vi "BIMS_SA.vi"() -> ()   [LabVIEW 2010]
doc: "This program is currently beta software. It is designed to address the data requirements defined primarily by the DHB Ballistic Test Report.\n\nThe general operation of this program is based on the Ballistics Version 2005 application developed internally by DuPont as a research tool for the Spruance Plant Ballistics Lab in Richmond, VA.\n\nPlease note that the original trigger control logic was modified and no longer depends on a safety interlock system to enable operation of a ballistic test.\n\nDuPont makes no warranties and assumes no liabilities in connection with any use of this program."
uses:
  Shot Record.ctl
  <vilib>/Utility/NIReport.llb/NI_report.lvclass
  <vilib>/Utility/config.llb/Write Key (String).vi
  <vilib>/Utility/NIReport.llb/Append Report Text (str wrap).vi
  <vilib>/Utility/NIReport.llb/Append Text Table to Report (wrap).vi
  <vilib>/addons/database/Connection.llb/DB Tools Open Connec (String).vi
  <vilib>/addons/database/Connection.llb/Conn Execute.vi
  <vilib>/addons/database/Recordset.llb/Rec Destroy - Connection.vi
  <vilib>/Utility/config.llb/Write Key (I32).vi
  <vilib>/addons/database/NI_Database_API.lvlib
  <vilib>/Utility/config.llb/NI_LVConfig.lvlib
  <vilib>/Analysis/NI_AALBase.lvlib
  <vilib>/Utility/NIReport.llb/Excel/NI_Excel.lvclass
panel:
  out "timestamp":string
  out "deployment":string
  in  "RESET All":bool
  in  "EXIT":bool
  in  "STOP":bool
  in  "mainTabCntrl":enum32{"SETUP", "MEASURE", "HISTORY", "ABOUT"}(tab)
  in  "setupTabCntrl":T1(tab)
  in  "rangeSetup":u16(ring) caption="Range\nSetup" items=["Select . . .", "Small frag (short)", "Handgun (standard)", "Rifle (long)"]
  out "mid_to_targ_dist":sgl=7.5 caption="Midpoint To Target (ft)"
  in  "Thickness":dbl caption="Thickness (in)" format="%.2f"
  in  "Model":u16(ring) caption="Model #"
  in  "clayCalArray":i16[](array[numeric])=[0, 0, 0, 0, 0] caption="Calibration" min=0 max=99 format="%02.0f"
  in  "Panel Dimensions":u16(ring)=6 caption="Panel Size" items=["15x15", "CHEST PLATE", "HELMET", "12x15", "16X16", "18X18", "20X16", "15\" x 18\"", "24 x 24", "13\"X13\"", "7.5\" X 7.5\"", "15x15", "VEST PANEL", "12X12", "101/4\" X 113/4\"", "15X16", "26X26", "NOT APPLICABLE", "8.5\" X 11\""]
  out "threatDetails":T2
  in  "projectileWt":u16(ring) caption="Weight (gr)" items=["Select . . .", "2", "4", "16", "17", "44", "45", "55", "62", "64", "85", "110", "115", "123", "124", "127", "148", "158", "166", "180", "207", "240"]
  out "clayAverage":sgl caption="Clay Average" format="%#.1f"
  in  "clayTemp":sgl caption="Clay Temperature" format="%.1f"
  in  "RoomT":sgl caption="Room Temperature" format="%.1f"
  in  "RoomHum":sgl caption="Room Humidity" min=0 max=100 format="%.1f"
  in  "Sample #":string
  in  "Comments":string caption="Remark"
  in  "recorder":u16(ring) caption="Recorder"
  in  "shooter":u16(ring) caption="Shooter"
  in  "rangeNum":u16(ring) caption="Range #" items=["1", "2", "Other"]
  in  "projectileType":u16(ring) caption="Projectile"
  in  "weapon":u16(ring) caption="Weapon"
  in  "minV50":i32=1500 caption="Min. V50"
  in  "covering":u16(ring) caption="Ballistic\nCover"
  in  "totalSampleWt":sgl caption="Total Wt (lbs)" format="%.2f"
  in  "serialNum":string caption="Serial #"
  in  "workType":u16(ring) caption="Work Type" items=["R&D", "QC", "Other"]
  in  "projNum":string caption="Project #"
  in  "projName":string caption="Project\nName"
  in  "standard":u16(ring) caption="Standard" items=["n/a", "NIJ 0101.04", "MIL-STD-662F"]
  in  "Powder Type":u16(ring) caption="Powder\nType" items=["WINCHESTER-231", "Alliant Herc. Bullseye", "Power Pistol", "ACCURATE, NO.9", "ACCURATE, NO. 2", "IMR-4756", "OTHER", "WINCHESTER-296", "Alliant 2400", "IMR-4198", "IMR-4895", "Hi-Skor 700x", "Hi-Skor 800x", "International Clay's", "Winchester Ball", "Hercules"]
  in  "Method":u16(ring) items=["V50", "N.I.J.", "Quasi N.I.J.", "VsVr", "CUSUM", "V(0)", "V(0) @ 1450", "V(0) @ 1500", "V(0) @ 1550"]
  in  "Layer_1":T3={"plyNum"=0, "LotNum"="n/a", "RollNum"="n/a", "Fabric.stitch"=1} caption="Fabric #1" {"plyNum" min=0 max=99 step=5}
  in  "Layer_2":T3={"plyNum"=0, "LotNum"="n/a", "RollNum"="n/a", "Fabric.stitch"=1} caption="Fabric #2" {"Fabric.stitch" items=["Corners", "Other", "n/a"]; "plyNum" min=0 max=99 step=5}
  in  "Layer_3":T3={"plyNum"=0, "LotNum"="n/a", "RollNum"="n/a", "Fabric.stitch"=1} caption="Fabric #3" {"Fabric.stitch" items=["Corners", "Other", "n/a"]; "plyNum" min=0 max=99 step=5}
  in  "Layer_4":T3={"plyNum"=0, "LotNum"="n/a", "RollNum"="n/a", "Fabric.stitch"=1} caption="Fabric #4" {"Fabric.stitch" items=["Corners", "Other", "n/a"]; "plyNum" min=0 max=99 step=5}
  in  "Layer_5":T3={"plyNum"=0, "LotNum"="n/a", "RollNum"="n/a", "Fabric.stitch"=1} caption="Fabric #5" {"Fabric.stitch" items=["Corners", "Other", "n/a"]; "plyNum" min=0 max=99 step=5}
  in  "Layer_6":T3={"plyNum"=0, "LotNum"="n/a", "RollNum"="n/a", "Fabric.stitch"=1} caption="Fabric #6" {"Fabric.stitch" items=["Corners", "Other", "n/a"]; "plyNum" min=0 max=99 step=5}
  out "fabAttribs_1":T4 caption="fabricAttribs_1"
  out "fabAttribs_2":T4 caption="fabricAttribs_2"
  out "fabAttribs_3":T4 caption="fabricAttribs_3"
  out "fabAttribs_4":T4 caption="fabricAttribs_4"
  out "fabAttribs_5":T4 caption="fabricAttribs_5"
  out "fabAttribs_6":T4 caption="fabricAttribs_6"
  in  "fabStyle_1":u16(ring)
  in  "fabStyle_2":u16(ring)
  in  "fabStyle_3":u16(ring)
  in  "fabStyle_4":u16(ring)
  in  "fabStyle_5":u16(ring)
  in  "fabStyle_6":u16(ring)
  in  "fabVendor_1":u16(ring) caption="vendor" items=[" Select Vendor . . .", "Barrday", "Cushman", "DSM", "FMS", "Hexcell", "Honeywell", "Lincoln", "Pro Systems", "TEIJIN", "TexTech"]
  in  "fabVendor_2":u16(ring) caption="vendor" items=[" Select Vendor . . .", "Barrday", "Cushman", "DSM", "FMS", "Hexcell", "Honeywell", "Lincoln", "Pro Systems", "TEIJIN", "TexTech"]
  in  "fabVendor_3":u16(ring) caption="vendor" items=[" Select Vendor . . .", "Barrday", "Cushman", "DSM", "FMS", "Hexcell", "Honeywell", "Lincoln", "Pro Systems", "TEIJIN", "TexTech"]
  in  "fabVendor_4":u16(ring) caption="vendor" items=[" Select Vendor . . .", "Barrday", "Cushman", "DSM", "FMS", "Hexcell", "Honeywell", "Lincoln", "Pro Systems", "TEIJIN", "TexTech"]
  in  "fabVendor_5":u16(ring) caption="vendor" items=[" Select Vendor . . .", "Barrday", "Cushman", "DSM", "FMS", "Hexcell", "Honeywell", "Lincoln", "Pro Systems", "TEIJIN", "TexTech"]
  in  "fabVendor_6":u16(ring) caption="vendor" items=[" Select Vendor . . .", "Barrday", "Cushman", "DSM", "FMS", "Hexcell", "Honeywell", "Lincoln", "Pro Systems", "TEIJIN", "TexTech"]
  out "fab6_totalWt":sgl caption="Fab6 Wt" min=0 max=99 step=5 format="%.2f"
  out "fab5_totalWt":sgl caption="Fab5 Wt" min=0 max=99 step=5 format="%.2f"
  out "fab4_totalWt":sgl caption="Fab4 Wt" min=0 max=99 step=5 format="%.2f"
  out "fab3_totalWt":sgl caption="Fab3 Wt" min=0 max=99 step=5 format="%.2f"
  out "fab2_totalWt":sgl caption="Fab2 Wt" min=0 max=99 step=5 format="%.2f"
  out "fab1_totalWt":sgl caption="Fab1 Wt" min=0 max=99 step=5 format="%.2f"
  out "totalNumPlies":i32 caption="Total # of Plies" min=0 max=100 step=5
  out "totalBAW":sgl caption="Total BAW (psf)" format="%.2f"
  in  "Next Shot":bool
  in  "Delete Button":bool
  in  "SHOTS":T5[](array[typedef]) {"UncorrectedAvgVel_PB" format="%.1f"; "strikeVel_PB" format="%.1f"; "velLoss_PB" format="%.1f"; "avgVel_PB" format="%.1f"; "Redundant_Velocity" format="%.1f"; "Energy Loss (J)" format="%.3e"; "Projectile Mass" min=0 step=1 format="%.4f"; "Corrected residual" format="%.2f"; "Uncorrected Residual" format="%.2f"; "Corrected Impact" format="%.2f"; "Uncorrected Impact" format="%.2f"; "Shot Angle" max=90 step=1; "SHOT STATUS" items=["Partial", "Complete"]; "IMPACT VELOCITY" min=0 max=10000 step=0.1 format="%.1f"; "Barrel Temperature" format="%.1f"; "Powder Loading" format="%.4f"; "RESIDUAL  VELOCITY" min=0 max=10000 step=0.1 format="%.1f"}
  in  "Refresh":bool
  in  "Accept Data":bool caption="RANGE SETUP must be selected before shots can be added."
  in  "Clear":bool
  out "Shot":i32
  out "Panel":i32
  out "rangeOfResults":i32 caption="Range of Results" min=0 max=10000 step=1
  out "lowComplete":i32 caption="LOW Complete" min=0 max=10000 step=1
  out "highPartial":i32 caption="HIGH Partial" min=0 max=10000 step=1
  out "Avg/speed":sgl caption="Average" min=0 max=10000 step=0.1 format="%.1f"
  in  "Current/avg/speed":sgl caption="Average" min=0 max=1000000 step=0.1 format="%.1f"
  out "Redundant/speed":sgl caption="Chronograph 2" min=0 max=10000 step=0.1 format="%.1f"
  in  "backfacedia":sgl caption="BF Diameter"
  in  "backdepth":sgl caption="BF Depth"
  out "% Difference":sgl format="%.1f"
  out "zmr 2":sgl caption="Z.M.R." format="%.1f"
  out "Pairs":i16 min=0 max=100 step=1
  out "computed_V50":sgl caption="Value" format="%.1f"
  in  "maxDev":sgl=125.0 caption="Maximum\nDeviation" min=0 max=300 step=25 format="%.1f"
  in  "B.F.S (mm)":u16 caption="B.F.S"
  in  "N.I.J":u16(ring) items=["Not Tested", "PASS", "FAIL"]
  in  "Projectile Mass":sgl caption="Proj Mass (g)" min=0 step=1 format="%.4f"
  in  "Shot Angle":u16 max=90 step=1
  in  "Powder Loading":sgl min=0 max=100 step=0.1 format="%.3f"
  in  "Shot Decription":string
  in  "Barrel Temp":sgl format="%.1f"
  out "DC_ factor":sgl caption="Correction Factor (Mid-Chrono 1&2)" format="%.4f"
  in  "Current/redundant/speed":sgl caption="Chronograph 2" min=0 max=1000000 step=0.1 format="%.1f"
  in  "currentDateTime":string caption="SUBMIT DATE/TIME"
  in  "Current/residual/speed":sgl caption="Residual" min=0 max=10000 step=0.1 format="%.1f"
  in  "Current/sthotstatus":u16(ring) caption="Penetration" items=["Partial", "Complete"]
  in  "Current/impact/speed":sgl caption="Chronograph 1" min=0 max=10000 step=0.1 format="%.1f"
  out "BACKFACE DEPTH":sgl caption="Backface\nDepth" min=0 max=200 step=5
  out "BACKFACE DIAMETER":sgl caption="Backface\nDiameter" min=0 max=100 step=5
  in  "Reject shot":bool
  out "SUBMIT DATE/TIME":string
  out "residual/speed":sgl caption="Residual" min=0 max=10000 step=0.1 format="%.1f"
  out "SHOT STATUS":u16(ring) caption="Penetration" items=["Partial", "Complete"]
  out "Impact/speed":sgl caption="Chronograph 1" min=0 max=10000 step=0.1 format="%.1f"
  in  "Table of Shots":string[][](table) caption="Shot Table"
  in  "RANGE RESET":bool=TRUE caption="ARMED"
  in  "Save":bool caption="Number of plies must be in FABRIC INFORMATION and \nSHOTS must exst in above table to enable saving"
  in  "Report_PB":bool caption="Report"
  in  "Report Path":path=path "c:/ballistics"
  out "instruct_addShot":string="RANGE SETUP must be selected before shots can be added."
  in  "historyTabCntrl":T6(tab)
  in  "srchParams":T7={"maxPanels"=1001, "lkupPanelStartDate"=timestamp(0 s since 1904-01-01), "lkupPanelEndDate"=timestamp(3253624514.0909824 s since 1904-01-01), "qWorkType"=0, "Model"=0, "fabStyle_0"=0, "fabVendor_0"=0} {"fabVendor_0" items=[" Select Vendor . . .", "Barrday", "Cushman", "DSM", "FMS", "Hexcell", "Honeywell", "Lincoln", "Pro Systems", "TEIJIN", "TexTech"]; "Model" items=["All Models", "n/a", "undefined", "other"]; "qWorkType" items=["All Types", "R&D", "QC", "Other"]; "lkupPanelEndDate" format="%<%x>T"; "lkupPanelStartDate" format="%<%x>T"; "maxPanels" min=1 max=10000 step=100}
  out "actualNumPanels":i32=1001 caption="Actual # Returned"
  out "pastPanels":string[][](table)
  in  "Record #":i32=1 min=0 max=37
  in  "getRecord":bool
  out "fabAttribs_0":T4 caption="fabricAttribs_1"
  in  "QueryLoad":bool
  in  "lkupEndDate":timestamp caption="End Date" format="%<%x>T"
  in  "lkupStartDate":timestamp caption="Begin Date" format="%<%x>T"
  out "Vel.vs.Loading":cluster{dbl[], dbl[]}(graph)
  out "v50_table":string[][](table)
  in  "maxRecs":u16=1001 caption="Max # of SHOT Records" min=1 max=10000 step=100
  out "ActualNumRecs":i32=1001 caption="Actual # Returned"
  out "Previous V50 Data":cluster{dbl, dbl, dbl[][]}(graph)={0.0, 1.0, []}
  out "v50 data":string[][](table)
  out "Average Velocity":dbl format="%.1f"
  out "CUSUM_lastVel":dbl caption="Latest Velocity" format="%.1f"
  out "CUSUM_stdDev":dbl caption="Std. Deviation" format="%.1f"
  in  "queryThreat":u16(ring) caption="Threat" items=["115-GRAIN,9mm LUGER,REFERENCE ROUND,10\" .38 cal TEST BBL.", "158-grain,WIN. 357 MAG, JHP REFERENCE ROUND, 10\" SAMMI TEST BBL.", "180-grain,WIN. 308 POWER-POINT REFERENCE ROUND, 308 TEST BBL.", "240-grain,REM. .44 mag, JSP REFERENCE ROUND, 8\" SAMMI TEST BBL."]
  out "In Control":bool=TRUE caption="Control Status"
  in  "Panel Search":bool
  in  "beginCUSUM":string="1/1/1900" caption="Begin Date"
  in  "endCUSUM":string="1/1/2100" caption="End Date"
  in  "aboutTabCntrl":T8(tab)
  out "Device S/N":string="DEVICE NOT READY!" caption="Timing Device S/N"
  in  "Data Source":u16(ring)=2 items=["Simulated", "Radar", "Screens", "Manual"]
  out "Distance Units":string="FEET"
  out "Weight Units":string="GRAMS"
  out "dbConn":string caption="Database Connection"
  in  "Sort by AVG":bool=TRUE caption="Sort shots by average velocity"
  out "configPath":path caption="Configuration Path (INI)"
  in  "Add Disclaimer":bool
  in  "Report":bool
  out "Shot Graph":cluster{i32[], sgl[]}[](graph)
  out "Corrected Average":sgl=2206.6846 format="%.2f"
  out "Corrected Redundant":sgl=2256.401 format="%.2f"
  out "conversion factor":sgl=0.3048037 format="%.5f"
  out "number of completes":i32=2
  out "number of partials":i32=2
  in  "percent warning":sgl=1.0 format="%.2f"
  in  "Version":dbl format="%.2f"
  out "impact/ID":u32=83886081 format="%.0x"
  out "residual/ID":u32=83951617 format="%.0x"
  out "Red/ID":u32=84017153 format="%.0x"
  out "correction coefficient":sgl=0.0252 format="%.8f"
  out "Corrected Residual":sgl=1210.3492 format="%.2f"
  out "Corrected Impact":sgl=2171.1157 format="%.2f"
  out "Impact/Separation":sgl=4.0 format="%.2f"
  out "Barrel to Screen":sgl=7.8333 format="%.2f"
  in  "Impact/Target Dist":sgl=7.083333 format="%.2f"
  out "Residual/Separation":sgl=4.0 format="%.2f"
  in  "Residual/Target Dist":sgl=7.083333 format="%.2f"
  out "Z.M.R.":sgl min=0 step=0.1 format="%.1f"
  in  "old threat":u16
  out "Complete":sgl[](array[numeric]) format="%.2f"
  out "factor array":sgl[](array[numeric])=[0.0252, 0.0191, 0.0191, 0.0441, 0.0425, 0.0131, 0.018] format="%.4f"
  out "Partial":sgl[](array[numeric]) format="%.2f"
  in  "DAQ Card":i16=1
  in  "Impact Timer":i16 min=0 max=3 step=1
  in  "Redundant Timer":i16=1 min=0 max=3 step=1
  in  "Residual  Timer":i16=2 min=0 max=3 step=1
  in  "Drag Corrected":bool
  out "Impact factor":sgl=0.94704616 caption="Impact" min=0 max=1 format="%.5f"
  out "Residual factor":sgl=1.0559148 caption="Residual" min=0 max=1 format="%.5f"
  in  "ballistician":u16(ring) caption="Ballistician" items=["n.a."]
  in  "Threat 2":u16(ring) caption="Threat" items=["110-grain(non-toxic)NYLON, 38 SPECIAL, POLY-TUNGSTEN, 10\" SAMMI TEST BBL.", "115-GRAIN,9mm LUGER,REFERENCE ROUND,.38 caliber chamber,10\" TEST BBL.", "115-GRAIN,9mm LUGER,REFERENCE ROUND,10\", 9mm, TEST BBL.", "115-grain, 9 mm, HI-SHOK JHP, +P+ FEDERAL, 10\" SAMMI TEST BBL.", "115-grain, 9 mm, HI-SHOK JHP, +P+ FEDERAL, 5\" SAMMI TEST BBL.", "115-grain,9mm,SMJ,SVENKA-BULLET,CHILE,S.A. 10\"SAMMI TEST BBL.", "123-grain,7.62mm AK-47            7.62mm SAAMI test bbl.", "124-grain,9mm FMJ Rem.#23558, 10\".357cal.SAAMI test bbl.", "124-grain,9mm,FMJ,Rem.#23558, .38 caliber chamber, 10\"SAAMI test bbl.1/10\" TWIST", "124-grain,9mm,FMJ,Rem.#23558, 10\"SAAMI test bbl.", "124-grain,9mm,FMJ,Rem.#23558, 5\"SAAMI test bbl.", "127-grain,9mm,SXT/Blck Tln, +P+,Win.RA9SXT SAAMI test bbl.", "148 grain 7.62 x 51 mm M80 ball", "148-grain,7.62mm FMJ  M80     7.62mm SAAMI test bbl.", "158-grain,0.357, JSP, Rem.#22487 10\"SAAMI test bbl.", "158-grain,0.357, JSP,SPEER.#4217,10\"SAAMI test bbl.", "158-grain,WIN. 357 MAG, JHP REFERENCE ROUND, 10\" SAMMI TEST BBL.", "16-grain,  saboted RCC,.308cal.SAAMI test bbl.,DC", "166-grain,.30 cal. M2 AP, 7.62mm SAAMI test bbl.", "17-grain,sabot,STANAG 2920, FSP,.308 cal. SAMMI test bbl., DC", "17-grain,sabot.Type 1,FSP,.308cal.SAAMI test bbl.,DC", "17-grain,sabot.Type 2,FSP,.308cal.SAAMI test bbl.,DC", "180-grain,40 cal. S&W, 5\"SAMMI test bbl.", "180-grain,WIN. 308 POWER-POINT REFERENCE ROUND, 308 TEST BBL.", "2-grain, saboted RCC FSP,.223cal.SAAMI test bbl.,DC", "207 grain, FSP, 50 Cal", "240 grain,0.44, SWC Speer #4660 no gc,8\"SAAMI test bbl.", "240-grain,0.44, FMJ Speer #4459, 8\" SAMMI test bbl.", "240-grain,0.44, JSP Speer #4457       8\"SAAMI test bbl.", "240-grain,0.44, SJHP,  REM.  # 23592,   8\"SAAMI test bbl.", "240-grain,0.44, SWC PMC w/Gas Check   8\"SAAMI test bbl.", "240-grain,REM. .44 mag, JSP REFERENCE ROUND, 8\" SAMMI TEST BBL.", "4-grain, saboted RCC FSP ,.223cal.SAAMI test bbl.,DC", "44-grain, 0.30-cal FSP - no sabot", "44-grain, 0.30-cal FSP - no sabot", "44-grain,sabot.      FSP,.458cal.SAAMI test bbl.,DC", "45-grain,JHP(WIN), .223 cal. SAMMI test bbl.", "55-grain, 0.223 M-193 FMJ        .223cal.SAAMI test bbl.", "62-grain, 0.223 M-855 Green Tip  .223cal SAAMI test bbl.", "64-grain,sabot.  RCC,.458cal.SAAMI test bbl.,DC", "85-grain(non-toxic), 38 SPECIAL FRANGIBLE,WIN # RA38DF,10\" SAMMI TEST BBL.", "85-grain(non-toxic), 9mm FRANGIBLE +P+,WIN # RA9DF, 5\" SAMMI TEST BBL.", "85-grain(non-toxic), 9mm FRANGIBLE +P+,WIN # RA9DF,10\" SAMMI TEST BBL.", "85-grain, 7.62mm Tokarev(LEAD CORE-STEEL JACKET,1992)Tokarev SAAMI test bbl."]
  in  "Panel Backing":u16(ring) items=["miscellaneous", "Clay (ROMA Plastilina # 1)", "Aluminum, 24 ga. (.020,.2024-T3) Witness Plate", "None"]
  in  "Submitter":u16(ring) items=["other"]
  in  "Test Conditions":u16(ring) items=["Dry", "Wet", "Hot 160 DEG. F", "Cold", "WEAPON LUBRICANT", "MOTOR OIL", "CONDITIONED", "ACCELERATED AGEING"]
  in  "Panel Stitch":u16(ring)=5 items=["TEST PANEL/NORMAL STITCH", "TEST PANEL/CUSTOM STITCH", "VEST PANEL/CUSTOM STITCH", "HARD PANEL", "CAR ARMOR LAMINATE PANEL", "N.A."]
  in  "Panel Type":u16(ring)=4 items=["FABRIC ARMOR", "COMPOSITE ARMOR", "LG.RIGHT FRONT VEST PANEL", "HELMET", "N.A."]
  in  "Type":u16(ring) items=["none"]
  in  "Manufacturer":u16(ring)=1 caption="Mfr" items=["Point Blank-Marine Interceptor"]
  in  "Areal Density":dbl format="%.2f"
  in  "Areal density text":string
  in  "Fabric Description":string
  in  "Weight of Panel":dbl format="%.4f"
  in  "Panel Technician":u16(ring) items=["Not Known", "none", "POINT BLANK"]
  in  "clayCalib":string="##-##-##-##-##" caption="Calibration"
  in  "lookupRec":bool caption="lookup"
  out "connStr":string
  in  "message control":bool
  # "yes"
  # "BIMS"
  # "Version 2011 for"
  # "No"
  # "GENERAL"
  # "SAMPLE"
  # "THREAT"
  # "RANGE"
  # "° F"
  # "%"
  # "° F"
  # "mm"
  # "mm"
  # "in"
  # "STRIKE FACE -------------------------------------------------------- MODEL CONSTRUCTION -------------------------------------------------------- BODY SIDE"
  # "Fabric 1"
  # "Fabric 2"
  # "Fabric 3"
  # "Fabric 4"
  # "Fabric 5"
  # "Fabric 6"
  # "Vendor"
  # "Style #"
  # "# of Plies"
  # "Lot#"
  # "Roll#"
  # "Stitch"
  # "ID#"
  # "Fiber"
  # "Denier"
  # "Pick"
  # "Weave"
  # "Finish"
  # "oz/yd²"
  # "Total Wt"
  # "Edit any non-date field by placing cursor in field. \n\nProperties not listed are controlled by the current shot, test description or Fabric information.  \nIf the entry is changed for the current shot, then all previous shots are changed"
  # "V50"
  # "Current Shot Data"
  # "(mm)"
  # "Number of plies must be in FABRIC INFORMATION and \nSHOTS must exst in above table to enable saving"
  # "Last Assigned\nRecord Numbers"
  # "ID#"
  # "Fiber"
  # "Denier"
  # "Pick"
  # "Weave"
  # "Finish"
  # "oz/yd²"
  # "BIMS\n\nBallistics Information Management System\n\nVersion 2011 (stand-alone)\n\nDecember 2006"
  # "Copyright © 2011 DuPont Company\n\nTech Support\n+1-302-545-3539"
  # "This software may be subject to revisions as additional experience and knowledge are gained. It is offered solely to provide possible suggestions for your own experimentation. It is not intended, however, to substitute for any testing you may need to conduct to determine for yourself the suitability of our software for your particular purposes. It is the user’s responsibility to determine the level of risk and the proper personal protection equipment needed. Because conditions are outside of our control, DUPONT MAKES NO WARRANTIES, EXPRESSED OR IMPLIED, AND ASSUMES NO LIABILITY WHATSOEVER AS TO THE PERFORMANCE OF THIS PRODUCT FOR A PARTICULAR USE. Nothing in this software is to be considered as a license to operate under or a recommendation to infringe any patent or trademark right. © 2011 E.I. du Pont de Nemours and Company. All rights reserved. DuPont™, the DuPont oval, the miracles of science®, KEVLAR ®, KEVLAR KM2 ®, are all trademarks or registered  trademarks of DuPont or its affiliates."
  # "Correction Factors"
  # "Yes"
  # "No"
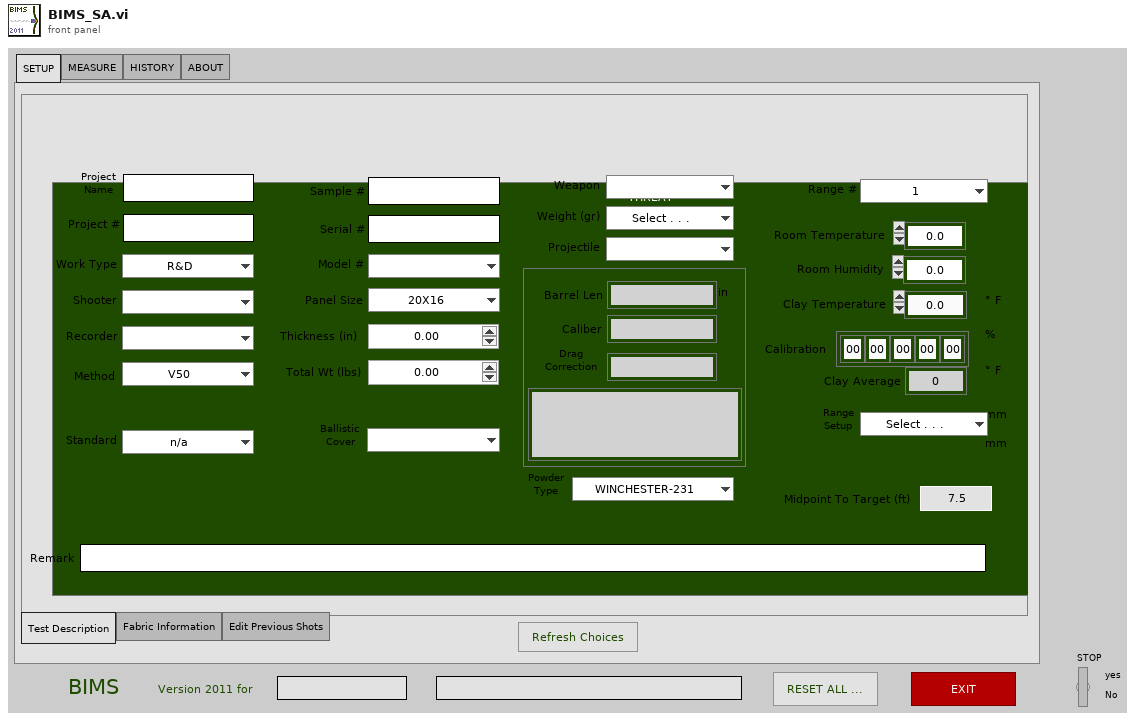
[diagram p1: front panel]
types:
  T1 = enum32{"Test Description", "Fabric Information", "Edit Previous Shots"}
  T2 = cluster{"barrelLength":string, "barrelCaliber":string, "dragCorrection":string, "detailDescription":string, "FK_threat":string}
  T3 = cluster{"plyNum":i32, "LotNum":string, "RollNum":string, "Fabric.stitch":u16}
  T4 = cluster{"Fabric.fiber":string, "Fabric.denier":string, "pick":string, "weave":string, "finish":string, "ozPerYd2":string, "fabricID_DHB":string, "SAK_fabric":string}
  T5 = typedef "Shot Record.ctl" = cluster{"avgVel_PB":sgl, "IMPACT VELOCITY":sgl, "RESIDUAL  VELOCITY ":sgl, "Shot Description":string, "Powder Loading ":sgl, "Barrel Temperature":sgl, "TIME / DATE":string, "shot order":i32, "SHOT STATUS":u16, "Shot Angle":u16, "Uncorrected Impact":sgl, "Corrected Impact":sgl, "Uncorrected Residual":sgl, "Corrected residual":sgl, "Projectile Mass":sgl, "usedv50":bool, "Energy Loss (J)":sgl, "BackFace\nDepth":sgl, "BackFace\nDiameter":sgl, "Redundant_Velocity":sgl, "velLoss_PB":sgl, "strikeVel_PB":sgl, "UncorrectedRed_PB":sgl, "CorrectedRed_PB":sgl, "UncorrectedAvgVel_PB":sgl}
  T6 = enum32{"Panel Lookup", "Powder Loading", "CUSUM"}
  T7 = cluster{"maxPanels":u16, "lkupPanelStartDate":timestamp, "lkupPanelEndDate":timestamp, "qWorkType":u16, "Model":u16, "fabStyle_0":u16, "fabVendor_0":u16}
  T8 = enum32{"About BIMS", "NIJ Reference", "MIL Spec", "System", "Internal Use"}
  T9 = cluster{"impactCntrID":u32, "redundantCntrID":u32, "residualCntrID":u32}
  T10 = cluster{"Charset (-1)":i16, "Weight (-1)":i16, "Name":string, "Size":string}
  T11 = cluster{"Italic":enum16{"Italic Unchanged", "Italic On", "Italic Off"}, "Strike Through":enum16{"Strike Through Unchanged", "Strike Through On", "Strike Through Off"}, "Underline":enum16{"Underline Unchanged", "Underline On", "Underline Off"}, "Bold":enum16{"Bold Unchanged", "Bold On", "Bold Off"}}
  T12 = enum16{"Standard Report", "HTML", "Word", "Excel"}
  T13 = cluster{"[0]":string, "[1]":string, "[2]":string, "[3]":string, "[4]":string, "[5]":string, "[6]":string, "[7]":string, "[8]":string, "[9]":string}[]
  T14 = cluster{"plyNum":i32, "LotNum":string, "RollNum":string, "Fabric.stitch":u16}[]
  T15 = cluster{"Fabric.fiber":string, "Fabric.denier":string, "pick":string, "weave":string, "finish":string, "ozPerYd2":string, "fabricID_DHB":string, "SAK_fabric":string}[]
  T16 = cluster{string, string, string, string, string, string, string, string, "clayCalib":string, string}
  T17 = cluster{string, string, string, string, string, string, string}
  T18 = cluster{"Sample #":string, "element":string, "element":string, "serialNum":string, "element":string, string, string, string, "element":string, string}
  T19 = cluster{"[0]":string, "[1]":string, "[2]":string, "[3]":string, "[4]":string, "[5]":string, "[6]":string, "[7]":string, "[8]":string, "[9]":string}
  T20 = cluster{"element":string, "element":string, "element":string, "element":string, "barrelLength":string, string, "element":string, "element":string, "element":string}
  T21 = typedef "NI_Database_API.lvlib/Conn ObjectReference.ctl" = refnum<k1>
  T22 = typedef "NI_Database_API.lvlib/Rec ObjectReference.ctl" = refnum<k1>
  T23 = typedef "NI_LVConfig.lvlib/Config Data RefNum.ctl" = refnum<k1>
  T24 = cluster{"task ID out":u32, "task ID out":u32, "task ID out":u32}
  T25 = enum32{"invalid app kind", "Development System", "Run Time System", "Student Edition", "Embedded LabVIEW", "Evaluation", "Custom"}
  T26 = typedef "LVRowAndColumnTypeDef.ctl" = cluster{"Row":i32, "Column":i32}
  T27 = cluster{"fiber":string, "denier":string, "pick":string, "weave":string, "finish":string, "ozPerYd2":string, "fabricStyle_DHB":string, "fabricStyle_DHB 2":string}
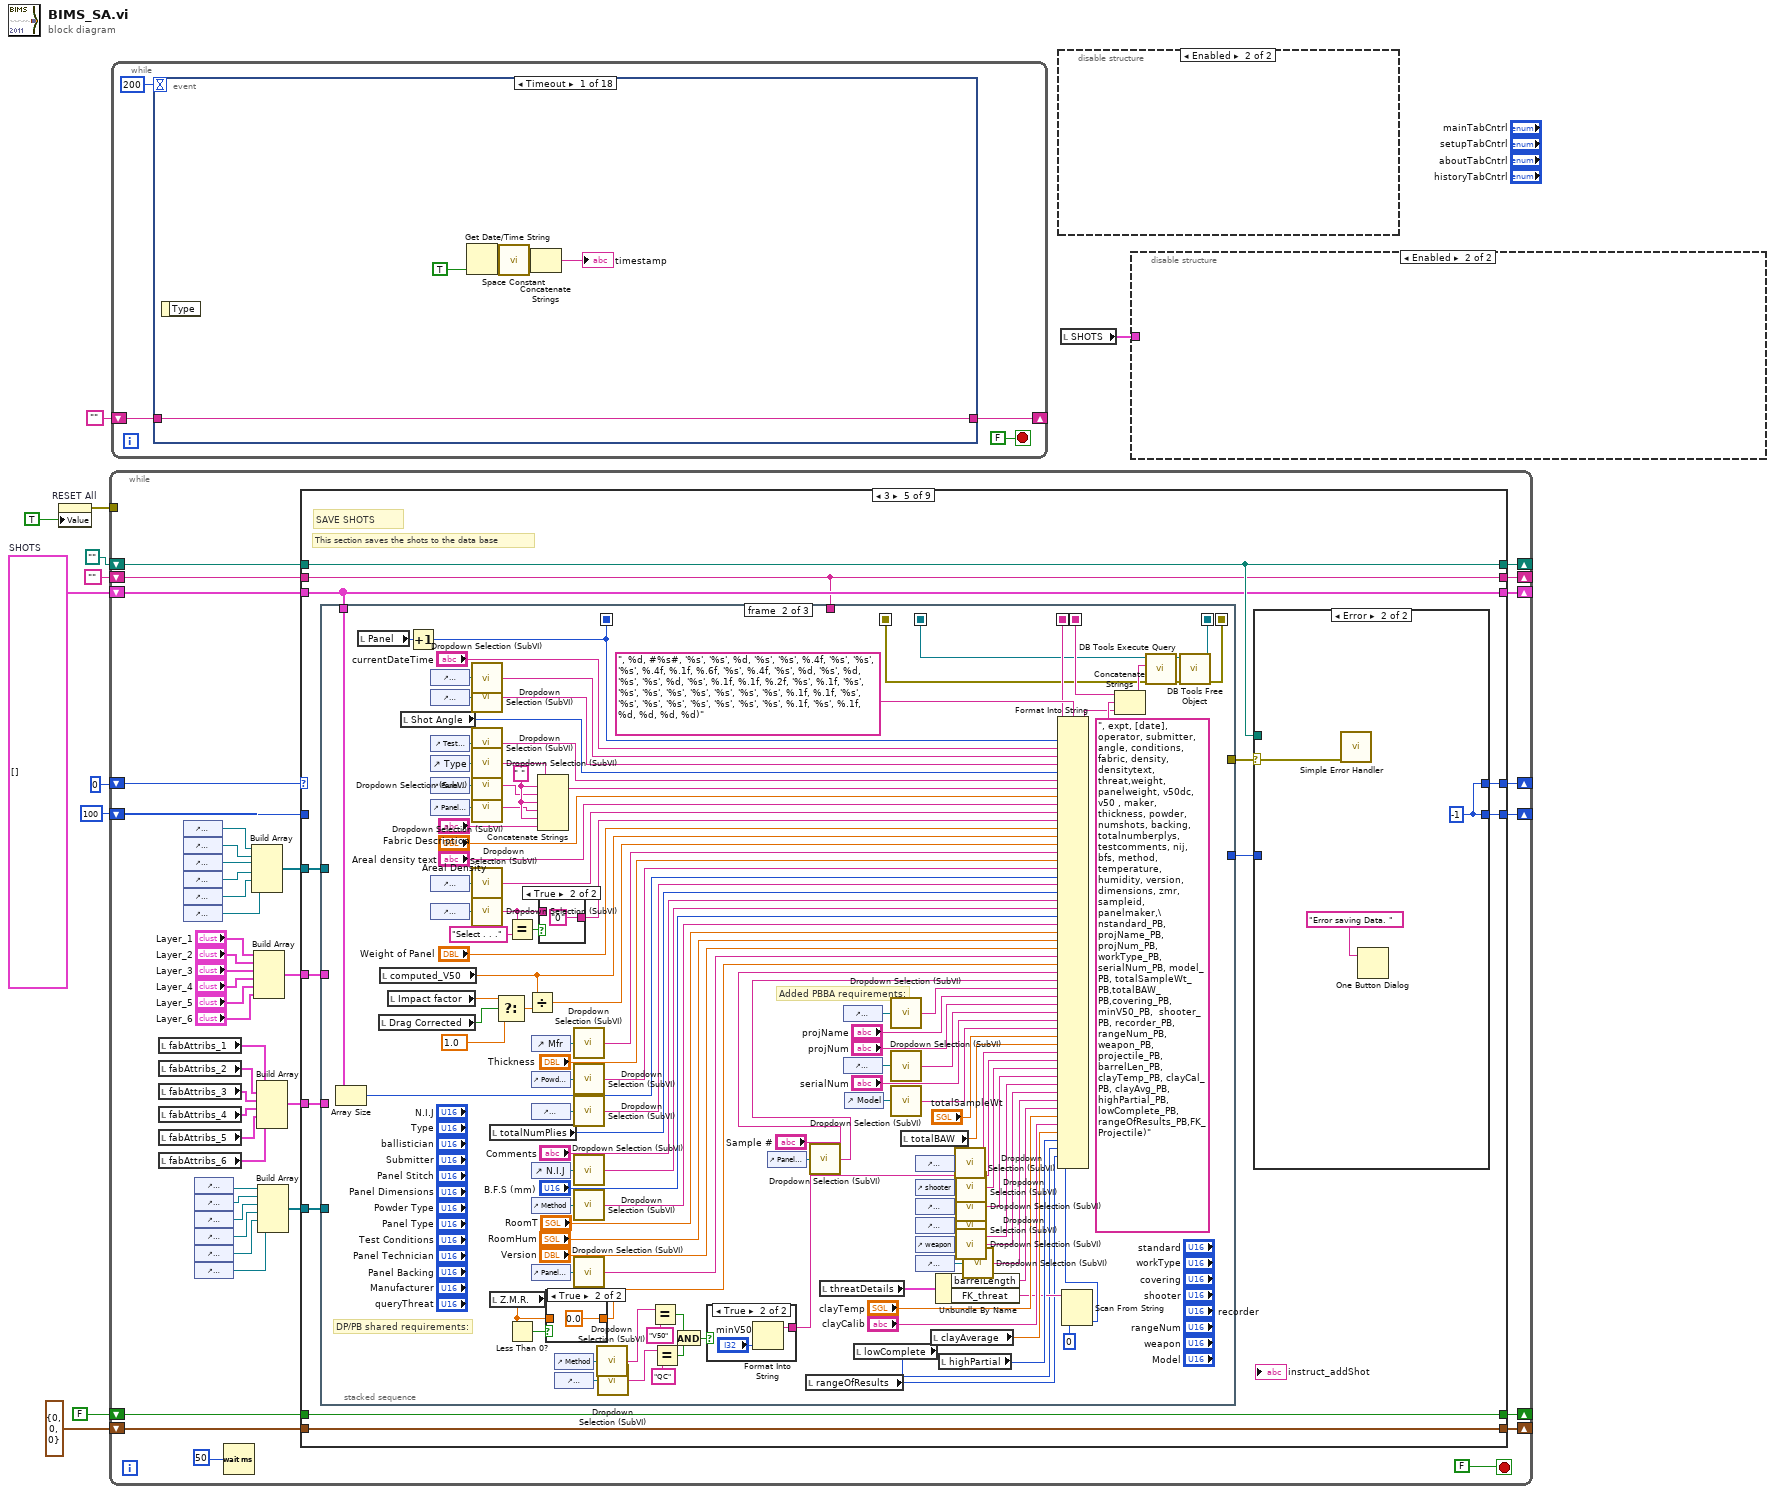
[diagram p0: block diagram]
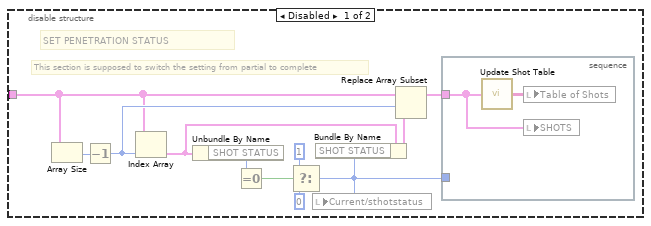
[diagram p2: hidden frame]
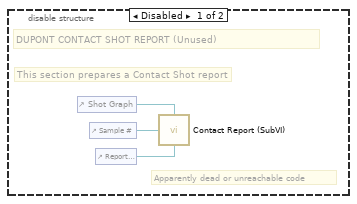
[diagram p3: hidden frame]
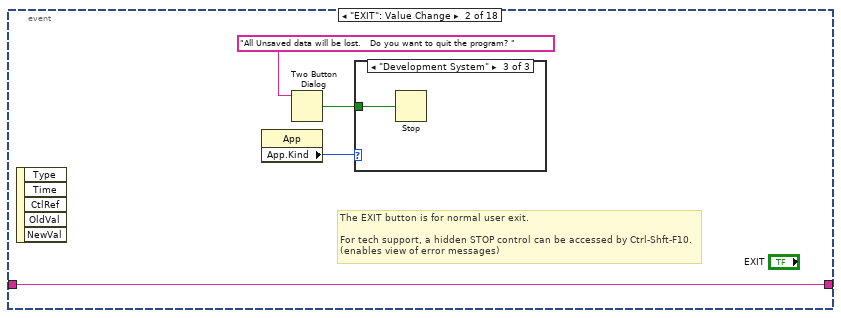
[diagram p4: hidden frame]
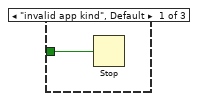
[diagram p5: hidden frame]
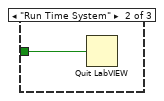
[diagram p6: hidden frame]
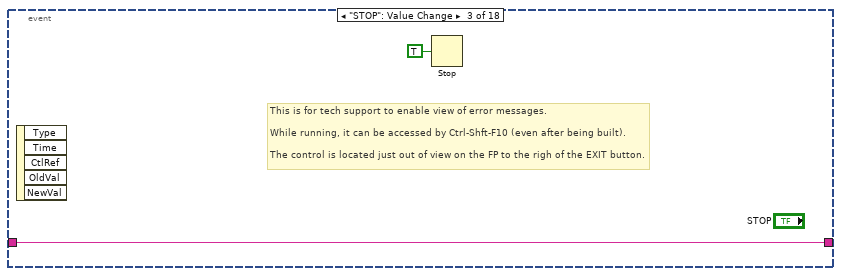
[diagram p7: hidden frame]
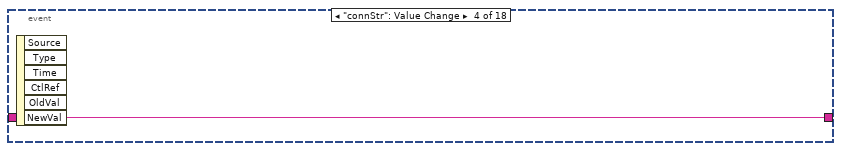
[diagram p8: hidden frame]
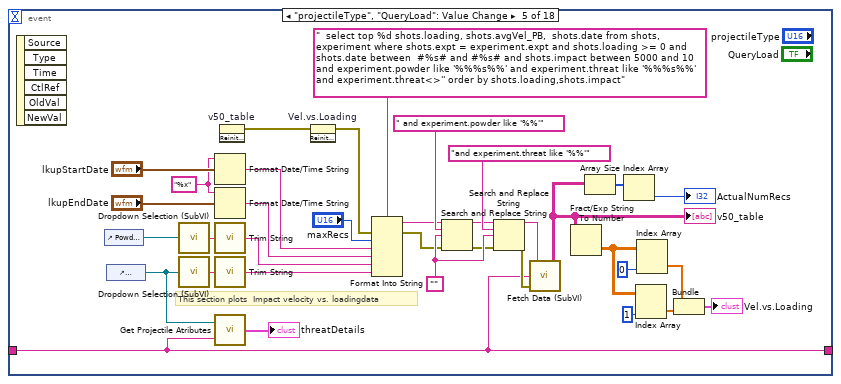
[diagram p9: hidden frame]
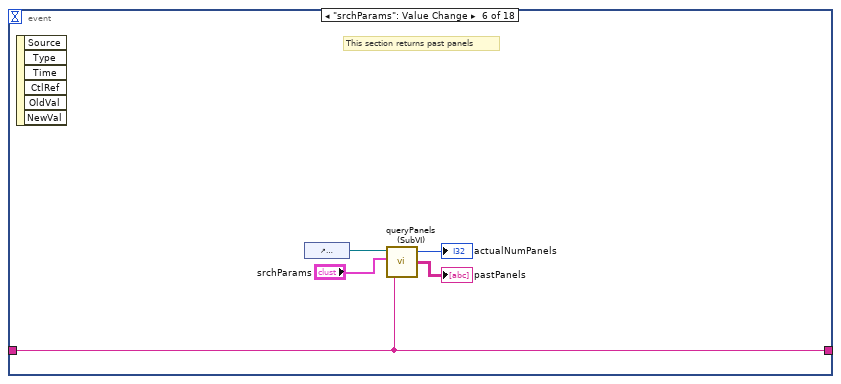
[diagram p10: hidden frame]
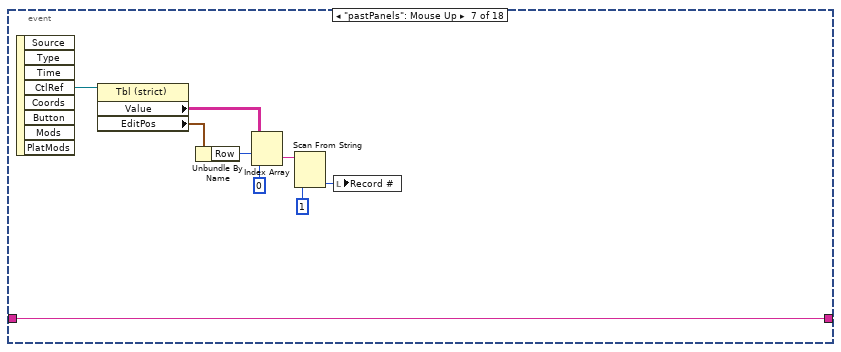
[diagram p11: hidden frame]
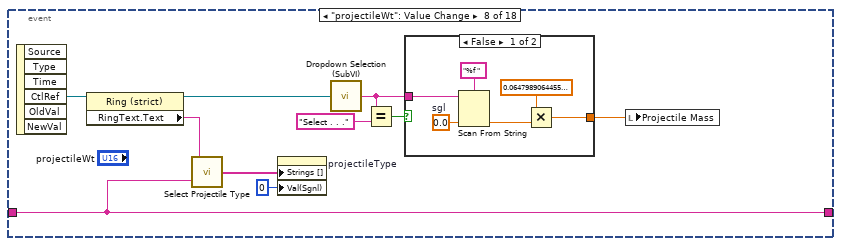
[diagram p12: hidden frame]
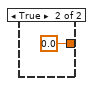
[diagram p13: hidden frame]
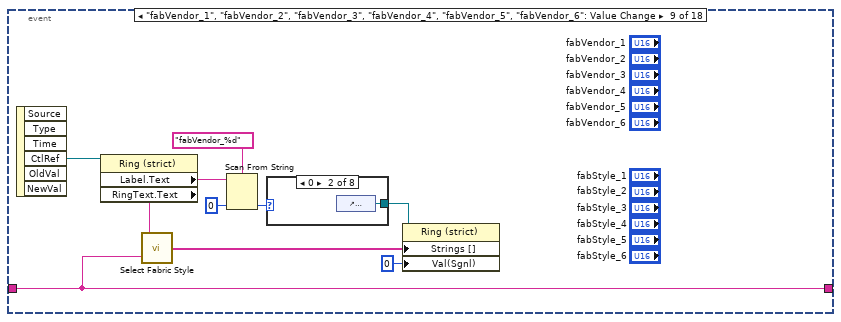
[diagram p14: hidden frame]
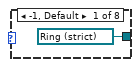
[diagram p15: hidden frame]
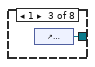
[diagram p16: hidden frame]
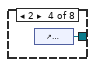
[diagram p17: hidden frame]
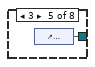
[diagram p18: hidden frame]
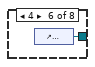
[diagram p19: hidden frame]
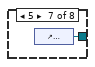
[diagram p20: hidden frame]
diagram:
  w5 = T5[] []  # SHOTS
  n1 = property on="RESET All" class="Bool (strict)"("Value"=TRUE ("RESET")) -> (error out=w8:errorcluster)  [unwired: 2 in, 1 out]
  n2 = while {
    shift-left: 100 -> [w51]
    shift-right: [w52] -> _
    shift-left: 0 ("index of element") -> [w55]
    shift-right: [w53] -> _
    tunnel: w8 -> [_]
    shift-right: [w49] -> _
    shift-left: T9 {"impactCntrID"=0, "redundantCntrID"=0, "residualCntrID"=0} -> [w48]
    shift-right: [w46] -> _
    shift-left: FALSE ("old drag") -> [w47]
    shift-right: [w44] -> _
    shift-left: w5 -> [w45]
    shift-right: [w15] -> _
    shift-left: path "" ("appended path OUT") -> [w14]
    shift-right: [w12] -> _
    shift-left: "" ("connectString") -> [w13]
    stop <- FALSE stop-if-true
    n3 = local read "fabAttribs_1"() -> (w43:T4)
    n4 = local read "fabAttribs_2"() -> (w41:T4)
    n5 = local read "fabAttribs_3"() -> (w40:T4)
    n6 = local read "fabAttribs_4"() -> (w39:T4)
    n7 = local read "fabAttribs_5"() -> (w38:T4)
    n8 = local read "fabAttribs_6"() -> (w42:T4)
    n9 = control-ref of="fabStyle_1"() -> (w22:refnum<vi>)
    n10 = control-ref of="fabStyle_2"() -> (w21:refnum<vi>)
    n11 = control-ref of="fabStyle_3"() -> (w20:refnum<vi>)
    n12 = control-ref of="fabStyle_4"() -> (w19:refnum<vi>)
    n13 = control-ref of="fabStyle_5"() -> (w18:refnum<vi>)
    n14 = control-ref of="fabStyle_6"() -> (w17:refnum<vi>)
    n15 = control-ref of="fabVendor_1"() -> (w29:refnum<vi>)
    n16 = control-ref of="fabVendor_2"() -> (w28:refnum<vi>)
    n17 = control-ref of="fabVendor_3"() -> (w27:refnum<vi>)
    n18 = control-ref of="fabVendor_4"() -> (w26:refnum<vi>)
    n19 = control-ref of="fabVendor_5"() -> (w25:refnum<vi>)
    n20 = control-ref of="fabVendor_6"() -> (w24:refnum<vi>)
    n21 = Wait (ms)(milliseconds to wait=u32 50 ("millisecond timer value")) -> ()  [unwired: 1 out]
    n22 = Build Array(w22, w21, w20, w19, w18, w17) -> (w16:refnum<vi>[])
    n23 = Build Array("Layer_1", "Layer_2", "Layer_3", "Layer_4", "Layer_5", "Layer_6") -> (w30:T14)
    n24 = Build Array(w43, w41, w40, w39, w38, w42) -> (w37:T15)
    n25 = Build Array(w29, w28, w27, w26, w25, w24) -> (w23:refnum<vi>[])
    n26 = case shown="3" w55 {
      tunnel: [w62 w470 w745 w797 w1102 w1418 w1424 w1434 w1491] -> w53
      tunnel: [w63 w470 w745 w797 w1101 w1418 w1424 w1434 w1491] -> w52
      tunnel: w51 -> [_ w473 _ _ _ _ _ _ _]
      tunnel: w45 -> [w64 w467 w605 w760 w1091 w1379 _ w1432 w1483]
      tunnel: w14 -> [w56 w472 w603 w762 w1092 w1377 w1420 w1428 w1482]
      tunnel: w13 -> [w57 w471 w602 w761 w1090 w1376 w1419 w1427 w1481]
      tunnel: [w61 w469 w623 w796 w1099 w1395 w1426 w1431 w1487] -> w49
      tunnel: w48 -> [w61 w469 w623 w796 w1099 w1395 w1426 w1431 w1486]
      tunnel: w47 -> [w59 w468 w606 w774 w1097 w1381 w1425 w1430 w1484]
      tunnel: [w60 w468 w606 w774 w1097 w1380 w1425 w1430 w1484] -> w46
      tunnel: [w58 w466 w605 w760 w1091 w1378 T5[] [] ("SHOTS") w1429 w1483] -> w44
      tunnel: w37 -> [_ _ _ w773 w1095 _ _ _ _]
      tunnel: w30 -> [_ _ _ w772 w1096 _ _ _ _]
      tunnel: w23 -> [_ w461 _ w771 w1093 _ _ _ _]
      tunnel: w16 -> [_ w465 _ w770 w1094 _ _ _ _]
      tunnel: [w56 w464 w603 w762 w1092 w1377 w1420 w1428 w1482] -> w15
      tunnel: [w57 w463 w602 w761 w1090 w1376 w1419 w1427 w1481] -> w12
      frame -1, Default {
        # "POLL"
        # "This section checks for any buttons, maintains routine check of the paramters"
        n27 = stacked-sequence {
          seq-local: [_ _ _ w339 _ _] -> [_ _ _ _ w373 _]
          seq-local: [_ _ w254 _ _ _] -> [_ _ _ w339 _ _]
          seq-local: [w67 _ _ _ _ _] -> [_ _ w232 _ _ _]
          tunnel: w64 -> [_ _ w231 _ w364 _]
          tunnel: [_ _ _ _ _ w430] -> w62
          tunnel: [_ _ _ _ _ -1] -> w63
          tunnel: w61 -> [w68 _ _ _ _ _]
          tunnel: [_ _ w233 _ _ _] -> w60
          tunnel: w59 -> [w66 _ _ _ _ _]
          tunnel: [_ _ _ _ w362 _] -> w58
          tunnel: w57 -> [_ _ _ _ _ w426]
          frame #0 {
            # "This section checks to see if the counters have been fired.  If they have then the counter times are read"
            n28 = local read "Data Source"() -> (w72:u16)
            n29 = Concatenate Strings("-1|", "F0|") -> (w69:string)
            n30 = case shown="3" w72 {
              tunnel: [errorcluster {"status"=FALSE, "code"=0, "source"=""} ("error out") errorcluster {"status"=FALSE, "code"=0, "source"=""} ("error out") w117 errorcluster {"status"=FALSE, "code"=0, "source"=""} ("error out")] -> w71
              tunnel: w69 -> [_ _ w113 _]
              tunnel: w68 -> [_ _ w109 _]
              tunnel: w66 -> [w74 w105 w108 w189]
              tunnel: [w73 w105 w107 w189] -> w67
              frame 0, Default {
                # "Simulated"
                n31 = local read "minV50"() -> (w78:i32)
                n32 = local read "Powder Loading"() -> (w98:sgl)
                n33 = To Single Precision Float(number=w78) -> (single precision float=w77:sgl)
                n34 = Not(x=w74) -> (.not. x?=w73:bool)
                n35 = call "Get Shell Speed.vi"("loading"=w98, "v50"=w77) -> ("impact"=w83:sgl, "residual"=w92:sgl)  [unwired: 2 in, 1 out]
                n36 = Random Number (0-1)() -> (number: 0 to 1=w90:dbl)
                n37 = To Single Precision Float(number=w90) -> (single precision float=w84:sgl)
                n38 = Multiply(x=w84, y=sgl 0.1) -> (x*y=w89:sgl)
                n39 = Add(x=w89, y=sgl 0.95) -> (x+y=w87:sgl)
                n40 = Greater Than 0?(x=w92) -> (x > 0?=w95:bool)
                n41 = Multiply(x=w83, y=w87) -> (x*y=w82:sgl)
                n42 = Add(x=w83, y=w82) -> (x+y=w80:sgl)
                n43 = Select(t=u16 1, s=w95, f=u16 0) -> (s? t:f=w93:u16)
                n44 = Divide(x=w80, y=sgl 2.0 ("v50")) -> (x/y=w79:sgl)
                n45 = local write "Current/impact/speed"(w83) -> ()
                n46 = local write "Current/residual/speed"(w92) -> ()
                n47 = local write "Current/sthotstatus"(w93) -> ()
                n48 = local write "SHOT STATUS"(w93) -> ()
                n49 = local write "Current/redundant/speed"(w82) -> ()
                n50 = local write "Current/avg/speed"(w79) -> ()
                n51 = Divide(x=sgl 2000.0, y=sgl 2.0 ("v50")) -> (x/y=w99:sgl)
                n52 = To Unsigned Long Integer(number=w99) -> (unsigned 32bit integer=w85:u32)
                n53 = local write "RANGE RESET"(TRUE ("RANGE RESET")) -> ()
                n54 = Wait (ms)(milliseconds to wait=w85) -> ()  [unwired: 1 out]
              }
              frame 1 {
                # "Radar -- (future)"
                n55 = local read "Current/redundant/speed"() -> (w100:sgl)
                n56 = local read "Current/impact/speed"() -> (w101:sgl)
                n57 = Add(x=w101, y=w100) -> (x+y=w103:sgl)
                n58 = Divide(x=w103, y=sgl 2.0) -> (x/y=w102:sgl)
                n59 = local write "Current/avg/speed"(w102) -> ()
              }
              frame 2 {
                # "Error -10600 occurrs in \"Read Count.vi\"\n\n  Possible reason(s):\n\n  NI-DAQ LV:\n    No setup operation has been performed for the specified resources. Or, some resources require a specific ordering of calls for proper setup.  \n\n  Solution: \n  To avoid this error, you must call the Dig_Line_Config function to setup the direction for each digital line prior to calling the Dig_Grp_Config function."
                # "Screens"
                n60 = Concatenate Strings(w113, "2|") -> (w112:string)
                n61 = Unbundle By Name(w109) -> ("impactCntrID"=w110:u32)
                n62 = call "Check Status.vi"("error in (no error)"=errorcluster {"status"=FALSE, "code"=0, "source"=""}, "TL Calling Location"=w112, "Task ID"=w110) -> ("error out"=w115:errorcluster, "Armed?"=w111:bool)  [unwired: 1 in]
                n63 = case shown="False" w111 {
                  tunnel: w115 -> [w143 w187]
                  tunnel: [w120 w187] -> w117
                  tunnel: w110 -> [w126 _]
                  tunnel: w112 -> [w139 _]
                  tunnel: w109 -> [w129 _]
                  tunnel: w108 -> [w119 w181]
                  tunnel: [w118 w181] -> w107
                  frame False {
                    n64 = Concatenate Strings(w139, "F|") -> (w134:string)
                    n65 = Not(x=w119) -> (.not. x?=w118:bool)
                    n66 = local read "Impact/Separation"() -> (w146:sgl)
                    n67 = call "Read Counter.vi"("TL Calling Location"=w134, "error In"=w143, "TASK ID"=w126) -> ("error out"=w128:errorcluster, "time (secs)"=w148:sgl)  [unwired: 3 in, 2 out]
                    n68 = Divide(x=w146, y=w148) -> (x/y=w122:sgl)
                    n69 = call "Arm One Channel.vi"("error IN"=w128, "task ID IN"=w126) -> ("error out"=w127:errorcluster)  [unwired: 2 in, 1 out]
                    n70 = Unbundle By Name(w129) -> ("redundantCntrID"=w131:u32)
                    n71 = Concatenate Strings(w134, "a|") -> (w137:string)
                    n72 = call "Check Status.vi"("error in (no error)"=w127, "TL Calling Location"=w137, "Task ID"=w131) -> ("error out"=w142:errorcluster, "Armed?"=w133:bool)  [unwired: 1 in]
                    n73 = case shown="False" w133 {
                      tunnel: [w159 sgl 0.0] -> w123
                      tunnel: w142 -> [w158 w163]
                      tunnel: [w153 w163] -> w144
                      tunnel: w131 -> [w152 _]
                      tunnel: w134 -> [w156 _]
                      frame False {
                        n74 = local read "Impact/Separation"() -> (w160:sgl)
                        n75 = Concatenate Strings(w156, "Fa|") -> (w155:string)
                        n76 = call "Read Counter.vi"("TL Calling Location"=w155, "error In"=w158, "TASK ID"=w152) -> ("error out"=w154:errorcluster, "time (secs)"=w161:sgl)  [unwired: 3 in, 2 out]
                        n77 = Divide(x=w160, y=w161) -> (x/y=w159:sgl)
                        n78 = call "Arm One Channel.vi"("error IN"=w154, "task ID IN"=w152) -> ("error out"=w153:errorcluster)  [unwired: 2 in, 1 out]
                      }
                      frame True {
                      }
                    }
                    n79 = Unbundle By Name(w129) -> ("residualCntrID"=w130:u32)
                    n80 = Concatenate Strings(w134, "b|") -> (w135:string)
                    n81 = call "Check Status.vi"("error in (no error)"=w144, "TL Calling Location"=w135, "Task ID"=w130) -> ("error out"=w141:errorcluster, "Armed?"=w132:bool)  [unwired: 1 in]
                    n82 = case shown="False" w132 {
                      tunnel: w141 -> [w170 w179]
                      tunnel: [w175 w180] -> w147
                      tunnel: w130 -> [w165 _]
                      tunnel: [w164 w179] -> w120
                      tunnel: [w172 sgl 0.0] -> w145
                      tunnel: w134 -> [w167 _]
                      frame False {
                        w176 = u16 1 items=["Partial", "Complete"] ("SHOT STATUS")
                        w177 = u16 0 items=["Partial", "Complete"] ("SHOT STATUS")
                        n83 = local read "Residual/Separation"() -> (w171:sgl)
                        n84 = Concatenate Strings(w167, "Fb|") -> (w168:string)
                        n85 = call "Read Counter.vi"("TL Calling Location"=w168, "error In"=w170, "TASK ID"=w165) -> ("error out"=w166:errorcluster, "counter overflow?"=w173:bool, "time (secs)"=w174:sgl)  [unwired: 3 in, 1 out]
                        n86 = Divide(x=w171, y=w174) -> (x/y=w172:sgl)
                        n87 = call "Arm One Channel.vi"("error IN"=w166, "task ID IN"=w165) -> ("error out"=w164:errorcluster)  [unwired: 2 in, 1 out]
                        n88 = Select(t=w177, s=w173, f=w176) -> (s? t:f=w175:u16)
                      }
                      frame True {
                        w180 = u16 1 items=["Partial", "Complete"] ("SHOT STATUS")
                      }
                    }
                    n89 = Add(x=w122, y=w123) -> (x+y=w124:sgl)
                    n90 = Divide(x=w124, y=sgl 2.0) -> (x/y=w121:sgl)
                    n91 = local write "Current/impact/speed"(w122) -> ()
                    n92 = local write "Current/avg/speed"(w121) -> ()
                    n93 = local write "Current/redundant/speed"(w123) -> ()
                    n94 = local write "Current/residual/speed"(w145) -> ()
                    n95 = local write "Current/sthotstatus"(w147) -> ()
                    n96 = local write "SHOT STATUS"(w147) -> ()
                    n97 = case shown="No Error" w120 {
                      selector: w120 -> [w151 _]
                      frame No Error {
                        n98 = Unbundle By Name(w151) -> ("status"=w150:bool)
                        n99 = Not(x=w150) -> (.not. x?=w149:bool)
                        n100 = local write "RANGE RESET"(w149) -> ()
                      }
                      frame Error {
                      }
                    }
                  }
                  frame True {
                    n101 = local read "Current/redundant/speed"() -> (w182:sgl)
                    n102 = local read "Current/impact/speed"() -> (w183:sgl)
                    n103 = Add(x=w183, y=w182) -> (x+y=w185:sgl)
                    n104 = Divide(x=w185, y=sgl 2.0) -> (x/y=w184:sgl)
                    n105 = local write "Current/avg/speed"(w184) -> ()
                  }
                }
              }
              frame 3 {
                n106 = local read "Current/redundant/speed"() -> (w190:sgl)
                n107 = local read "Current/impact/speed"() -> (w191:sgl)
                n108 = Add(x=w191, y=w190) -> (x+y=w193:sgl)
                n109 = Divide(x=w193, y=sgl 2.0) -> (x/y=w192:sgl)
                n110 = local write "Current/avg/speed"(w192) -> ()
              }
            }
            n111 = call <vilib>:"Simple Error Handler.vi"("error in (no error)"=w71) -> ()  [unwired: 4 in, 5 out]
          }
          frame #1 {
            n112 = local read "Current/impact/speed"() -> (w214:sgl)
            n113 = local read "Z.M.R."() -> (w217:sgl)
            n114 = local read "Current/redundant/speed"() -> (w215:sgl)
            n115 = Absolute Value(x=w217) -> (abs(x)=→"zmr 2":sgl)
            n116 = Add(x=w215, y=w214) -> (x+y=w213:sgl)
            n117 = Subtract(x=w215, y=w214) -> (x-y=w216:sgl)
            n118 = Divide(x=w213, y=sgl 200.0) -> (x/y=w212:sgl)
            n119 = Divide(x=w216, y=w212) -> (x/y=w208:sgl)
            "% Difference" <- w208
            n120 = Less Than 0?(x=w217) -> (x < 0?=w223:bool)
            n121 = Select(t="Lo C.- Hi P.", s=w223, f="Z.M.R.") -> (s? t:f=w220:string)
            n122 = Absolute Value(x=w208) -> (abs(x)=w205:sgl)
            n123 = Select(t=u32 65336, s=w223, f=u32 16755266) -> (s? t:f=w219:u32)
            n124 = Less?(x=w205, y="percent warning") -> (x < y?=w206:bool)
            n125 = property on="zmr 2" class="DigNum (strict)"("Caption.Text"=w220, "Numeric Text.Text Colors:BG Color"=w219) -> ()  [unwired: 2 in, 2 out]
            n126 = Select(t=u32 65343, s=w206, f=u32 15668992) -> (s? t:f=w204:u32)
            n127 = property on="% Difference" class="DigNum (strict)"("Numeric Text.Text Colors:BG Color"=w204) -> ()  [unwired: 2 in, 2 out]
            n128 = local read "Data Source"() -> (w195:u16)
            n129 = case shown="..2" w195 {
              frame 3, Default {
              }
              frame ..2 {
                n130 = Get Date/Time In Seconds() -> (seconds since 1Jan1904=w227:timestamp)
                n131 = To Double Precision Float(number=w227) -> (double precision float=w229:dbl)
                n132 = Format Date/Time String(time format string (%c)="%x   %H:%M:%S", seconds (now)=w229) -> (date/time string=w226:string)  [unwired: 1 in]
                n133 = local write "currentDateTime"(w226) -> ()
              }
            }
            n134 = local read "Fabric Description"() -> (w201:string)
            n135 = local read "Shot Decription"() -> (w198:string)
            n136 = String Subset(string=w201, length (rest)=75 ("length (rest)")) -> (substring=w200:string)  [unwired: 1 in]
            n137 = String Subset(string=w198, length (rest)=30 ("length (rest)")) -> (substring=w196:string)  [unwired: 1 in]
            n138 = local write "Fabric Description"(w200) -> ()
            n139 = local write "Shot Decription"(w196) -> ()
            "BACKFACE DIAMETER" <- "backfacedia"
            "BACKFACE DEPTH" <- "backdepth"
          }
          frame #2 {
            n140 = disable-structure shown="Enabled" {
              disable-tunnel: "Threat 2" -> [w264 _]
              disable-tunnel: [w262 w268] -> w239
              frame Disabled {
                n141 = local read "factor array"() -> (w265:sgl[])
                n142 = To Long Integer(number=w264) -> (32bit integer=w263:i32)
                n143 = Index Array(array=w265, index=w263) -> (element=w262:sgl)
              }
              frame Enabled {
                n144 = local read "threatDetails"() -> (w266:T2)
                n145 = Unbundle By Name(w266) -> ("dragCorrection"=w267:string)
                n146 = Scan From String(input string=w267, default 1=sgl 0.0 ("default value 1")) -> (output 1=w268:sgl)  [unwired: 3 in, 3 out]
              }
            }
            "correction coefficient" <- w239
            n147 = local read "mid_to_targ_dist"() -> (w230:sgl)
            n148 = local read "Distance Units"() -> (w240:string)
            n149 = call "Compute Strike Velocity.vi"("drag coefficient"=w239, "decay distance"=w230, "raw velocity"="Current/avg/speed", "distance units"=w240) -> ("correction factor"=w234:sgl, "strike velocity"=w235:sgl)  [unwired: 1 out]
            "DC_ factor" <- w234
            "Corrected Average" <- w235
            n150 = call "Velocity Correction.vi"("raw impact"="Current/impact/speed", "distance units"=w240, "raw redundant"="Current/redundant/speed", "raw residual"="Current/residual/speed", "impact screen to target"="Impact/Target Dist", "residual screen to target"="Residual/Target Dist", "correction coefficient"=w239) -> ("corrected impact"=w250:sgl, "corrected redundant"=w243:sgl, "corrected residual"=w248:sgl, "impact factor"=w246:sgl, "conversion factor"=→"conversion factor":sgl, "residual factor"=w245:sgl)  [unwired: 3 in]
            "Residual factor" <- w245
            "Impact factor" <- w246
            "Corrected Impact" <- w250
            "Corrected Residual" <- w248
            "Corrected Redundant" <- w243
            n151 = Not Equal?(x="Drag Corrected", y=w232) -> (x != y?=w256:bool)
            n152 = Select(t=w243, s="Drag Corrected", f="Current/redundant/speed") -> (s? t:f=→"Redundant/speed":sgl)
            n153 = Select(t=w235, s="Drag Corrected", f="Current/avg/speed") -> (s? t:f=→"Avg/speed":sgl)
            n154 = Select(t=w250, s="Drag Corrected", f="Current/impact/speed") -> (s? t:f=→"Impact/speed":sgl)
            n155 = Select(t=w248, s="Drag Corrected", f="Current/residual/speed") -> (s? t:f=→"residual/speed":sgl)
            n156 = Not Equal?(x="Threat 2", y="old threat") -> (x != y?=w257:bool)
            n157 = Or(x=w257, y=w256) -> (x .or. y?=w255:bool)
            n158 = case shown="True" w255 {
              tunnel: "Threat 2" -> [_ w278]
              tunnel: w231 -> [w271 w277]
              tunnel: w245 -> [_ w276]
              tunnel: w246 -> [_ w275]
              tunnel: "Drag Corrected" -> [w270 w272]
              tunnel: [w271 w274] -> w254
              tunnel: w234 -> [_ w273]
              tunnel: [w270 w272] -> w233
              frame False {
              }
              frame True {
                n159 = local write "old threat"(w278) -> ()
                n160 = disable-structure shown="Disabled" {
                  frame Disabled {
                    w279 = sgl 0.0  # sgl
                    n161 = property on="Threat 2" class="Ring (strict)"() -> ("Strings []"=w287:string[], "Value"=w286:u16)  [unwired: 2 in, 2 out]
                    n162 = To Long Integer(number=w286) -> (32bit integer=w281:i32)
                    n163 = Index Array(array=w287, index=w281) -> (element=w285:string)
                    n164 = Scan From String(format string="%f " ("Format String"), input string=w285, default 1=w279) -> (output 1=w280:sgl)  [unwired: 2 in, 3 out]
                    n165 = Multiply(x=sgl 0.06479891, y=w280) -> (x*y=w282:sgl)
                    n166 = local write "Projectile Mass"(w282) -> ()
                  }
                  frame Enabled {
                  }
                }
                n167 = for {
                  tunnel: w277 -> [w294] mode=indexing
                  tunnel: w276 -> [w304]
                  tunnel: w275 -> [w299]
                  tunnel: w272 -> [w291]
                  tunnel: [w306] -> w274 mode=indexing
                  tunnel: w273 -> [w292]
                  n168 = Unbundle By Name(w294) -> ("UncorrectedAvgVel_PB"=w293:sgl)
                  n169 = Unbundle By Name(w294) -> ("UncorrectedRed_PB"=w301:sgl)
                  n170 = Unbundle By Name(w294) -> ("Uncorrected Impact"=w298:sgl)
                  n171 = Unbundle By Name(w294) -> ("Uncorrected Residual"=w303:sgl)
                  n172 = Multiply(x=w292, y=w293) -> (x*y=w289:sgl)
                  n173 = Multiply(x=w299, y=w301) -> (x*y=w300:sgl)
                  n174 = Multiply(x=w299, y=w298) -> (x*y=w296:sgl)
                  n175 = Multiply(x=w304, y=w303) -> (x*y=w295:sgl)
                  n176 = Select(t=w289, s=w291, f=w293) -> (s? t:f=w290:sgl)
                  n177 = Select(t=w300, s=w291, f=w301) -> (s? t:f=w302:sgl)
                  n178 = Select(t=w295, s=w291, f=w303) -> (s? t:f=w305:sgl)
                  n179 = Select(t=w296, s=w291, f=w298) -> (s? t:f=w297:sgl)
                  n180 = Subtract(x=w290, y=w289) -> (x-y=w288:sgl)
                  n181 = Bundle By Name(cluster=w294, "velLoss_PB"=w288, "strikeVel_PB"=w289, "avgVel_PB"=w290, "CorrectedRed_PB"=w300, "Redundant_Velocity"=w302, "Corrected Impact"=w296, "IMPACT VELOCITY"=w297, "Corrected residual"=w295, "RESIDUAL  VELOCITY"=w305) -> (w306:T5)
                }
              }
            }
            "SHOT STATUS" <- "Current/sthotstatus"
          }
          frame #3 {
            w308 = sgl[] [] ("Partial")
            # "This section calculates the V50"
            n182 = Array Size(array=w339) -> (size(s)=w338:i32)
            n183 = local read "totalNumPlies"() -> (w335:i32)
            n184 = Equal To 0?(x=w338) -> (x = 0?=w329:bool)
            n185 = Equal To 0?(x=w335) -> (x = 0?=w334:bool)
            n186 = Or(x=w329, y=w334) -> (x .or. y?=w307:bool)
            n187 = Select(t=u8 2, s=w329, f=u8 0) -> (s? t:f=w330:u8)
            n188 = Select(t=u8 2, s=w307, f=u8 0) -> (s? t:f=w333:u8)
            n189 = property on="Save" class="Bool"("Disabled"=w333) -> ()  [unwired: 2 in, 2 out]
            n190 = property on="Clear" class="Bool"("Disabled"=w330) -> ()  [unwired: 2 in, 2 out]
            n191 = for {
              shift-right: [w348] -> w311
              shift-left: w308 -> [w349]
              shift-right: [w346] -> w310
              shift-left: w308 -> [w347]
              tunnel: w339 -> [w344] mode=indexing
              shift-right: [w342] -> w309
              shift-left: w308 -> [w341]
              # "Here, DuPont uses:\n\nIMPACT VELOCITY"
              n192 = Unbundle By Name(w344) -> ("strikeVel_PB"=w340:sgl, "SHOT STATUS"=w345:u16)
              n193 = Unbundle By Name(w344) -> ("usedv50"=w343:bool)
              n194 = case shown="True" w343 {
                tunnel: [w350 w353] -> w342
                tunnel: w341 -> [w350 w352]
                tunnel: w340 -> [_ w351]
                frame False {
                }
                frame True {
                  n195 = Build Array (concatenate)(w352, w351) -> (w353:sgl[])
                }
              }
              n196 = case shown="0, Default" w345 {
                tunnel: w340 -> [w354 w358]
                tunnel: [w357 w359] -> w348
                tunnel: w349 -> [w356 w359]
                tunnel: w347 -> [w355 w361]
                tunnel: [w355 w360] -> w346
                frame 0, Default {
                  n197 = Build Array (concatenate)(w356, w354) -> (w357:sgl[])
                }
                frame 1 {
                  n198 = Build Array (concatenate)(w361, w358) -> (w360:sgl[])
                }
              }
            }
            n199 = Sort 1D Array(array=w311) -> (sorted array=w328:sgl[])
            n200 = Sort 1D Array(array=w310) -> (sorted array=w316:sgl[])
            "Complete" <- w316
            n201 = Array Max & Min(array=w309) -> (max value=w320:sgl, min value=w319:sgl)  [unwired: 2 out]
            n202 = Array Size(array=w316) -> (size(s)=→"number of completes":i32)
            n203 = Reverse 1D Array(array=w328) -> (reversed array=w314:sgl[])
            "Partial" <- w314
            n204 = Array Max & Min(array=w316) -> (min value=w322:sgl)  [unwired: 3 out]
            n205 = Subtract(x=w320, y=w319) -> (x-y=w318:sgl)
            n206 = Array Size(array=w314) -> (size(s)=→"number of partials":i32)
            n207 = Array Max & Min(array=w314) -> (max value=w324:sgl)  [unwired: 3 out]
            n208 = call "Compute V50.vi"("Maximum Deviation"="maxDev", "Partial"=w314, "Complete"=w316) -> ("zmr"=→"Z.M.R.":sgl, "Points"=→"Pairs":i16, "V50"=→"computed_V50":sgl)
            n209 = To Long Integer(number=w318) -> (32bit integer=→"rangeOfResults":i32)
            n210 = To Long Integer(number=w324) -> (32bit integer=→"highPartial":i32)
            n211 = To Long Integer(number=w322) -> (32bit integer=→"lowComplete":i32)
          }
          frame #4 {
            n212 = local read "Pairs"() -> (w370:i16)
            n213 = Sort 1D Array(array=w373) -> (sorted array=w367:T5[])
            n214 = for {
              tunnel: w367 -> [w418] mode=indexing
              tunnel: w370 -> [w409]
              shift-right: [w408] -> _
              shift-left: i16 0 -> [w407]
              tunnel: [w401] -> w368 mode=indexing
              # "this section marks the lowest completes that are used in V50"
              n215 = Unbundle By Name(w418) -> ("SHOT STATUS"=w405:u16, "Projectile Mass"=w403:sgl, "avgVel_PB"=w402:sgl, "RESIDUAL  VELOCITY"=w404:sgl)
              n216 = local read "conversion factor"() -> (w411:sgl)
              n217 = case shown="1" w405 {
                tunnel: w409 -> [_ w425]
                tunnel: [FALSE w424] -> w406
                tunnel: [w420 w423] -> w408
                tunnel: w407 -> [w420 w421]
                frame 0, Default {
                }
                frame 1 {
                  n218 = Less?(x=w421, y=w425) -> (x < y?=w424:bool)
                  n219 = Add(x=w421, y=i16 1 ("t")) -> (x+y=w423:i16)
                }
              }
              n220 = Multiply(x=w411, y=w404) -> (x*y=w412:sgl)
              n221 = Multiply(x=w402, y=w411) -> (x*y=w413:sgl)
              n222 = Multiply(x=w413, y=w413) -> (x*y=w417:sgl)
              n223 = Multiply(x=w412, y=w412) -> (x*y=w416:sgl)
              n224 = Subtract(x=w417, y=w416) -> (x-y=w415:sgl)
              n225 = Compound Arithmetic op=MULTIPLY(w403, w415, sgl 0.0005 ("Input")) -> (w410:sgl)
              n226 = Bundle By Name(cluster=w418, "usedv50"=w406, "Energy Loss (J)"=w410) -> (w401:T5)
            }
            n227 = Reverse 1D Array(array=w368) -> (reversed array=w366:T5[])
            n228 = for {
              tunnel: w366 -> [w378] mode=indexing
              tunnel: w370 -> [w381]
              shift-right: [w379] -> _
              shift-left: i16 0 -> [w380]
              tunnel: [w376] -> w363 mode=indexing
              # "chooses highest partials used in v50"
              n229 = Unbundle By Name(w378) -> ("SHOT STATUS"=w382:u16, "usedv50"=w375:bool)
              n230 = case shown="0, Default" w382 {
                tunnel: w381 -> [w386 _]
                tunnel: [w385 w389] -> w377
                tunnel: w380 -> [w383 w388]
                tunnel: [w384 w388] -> w379
                tunnel: w375 -> [_ w389]
                frame 0, Default {
                  n231 = Less?(x=w383, y=w386) -> (x < y?=w385:bool)
                  n232 = Add(x=w383, y=i16 1) -> (x+y=w384:i16)
                }
                frame 1 {
                }
              }
              n233 = Bundle By Name(cluster=w378, "usedv50"=w377) -> (w376:T5)
            }
            n234 = case shown="True" "Next Shot" {
              tunnel: w363 -> [w390 w392]
              tunnel: [w390 w391] -> w362
              frame False {
              }
              frame True {
                n235 = property on="SHOTS" class="Arr (strict)"() -> ("Index Values"=w394:u32[])  [unwired: 2 in, 2 out]
                n236 = local write "Next Shot"(FALSE ("Boolean")) -> ()
                n237 = Array Size(array=w392) -> (size(s)=w397:i32)
                n238 = Index Array(array=w394) -> (element=w399:u32)  [unwired: 1 in]
                n239 = To Unsigned Long Integer(number=w397) -> (unsigned 32bit integer=w393:u32)
                n240 = Increment(x=w399) -> (x+1=w398:u32)
                n241 = Quotient & Remainder(x=w398, y=w393) -> (x-y*floor(x/y)=w396:u32)  [unwired: 1 out]
                n242 = Replace Array Subset(array=w394, new element=w396) -> (w395:u32[])  [unwired: 1 in]
                n243 = property on="SHOTS" class="Arr (strict)"("Index Values"=w395) -> ("Value"=w391:T5[])  [unwired: 2 in, 2 out]
              }
            }
            n244 = Not Equal?(x=w364, y=w362) -> (x != y?=w365:bool)
            n245 = case shown="True" w365 {
              tunnel: w362 -> [_ w374]
              frame False {
              }
              frame True {
                n246 = property on="SHOTS" class="Arr (strict)"("Val(Sgnl)"=w374) -> ()  [unwired: 2 in, 2 out]
              }
            }
          }
          frame #5 {
            w438 = TRUE  # element
            n247 = Or(x="RESET All", y="Refresh") -> (x .or. y?=w446:bool)
            n248 = Or(x="Report_PB", y="getRecord") -> (x .or. y?=w428:bool)
            n249 = Or(x="Reject shot", y="Delete Button") -> (x .or. y?=w441:bool)
            n250 = Build Array(w446, "Report", w428, "Save", "Accept Data", "Clear", w441, "RANGE RESET") -> (w437:bool[])
            n251 = Search 1D Array(1D array=w437, element=w438) -> (index of element=w431:i32)  [unwired: 1 in]
            n252 = Equal?(x=w431, y=3) -> (x = y?=w432:bool)
            n253 = case shown="False" w432 {
              tunnel: w431 -> [w448 w453]
              tunnel: [w448 w458] -> w430
              tunnel: w426 -> [_ w449]
              frame False {
              }
              frame True {
                # "Before allowing data record to be saved,\nprompt user to validate."
                n254 = call "Get Last Record (SubVI).vi"("connect Str"=w449) -> ("shot record"=w451:i32, "experiment record"=w450:i32)  [unwired: 1 out]
                n255 = Two Button Dialog(message="Are ALL Data Valid?", 1:"NO" ("F button name (\"Cancel\")"), 2:"YES" ("T button name (\"OK\")")) -> (T button?=w457:bool)
                n256 = To Double Precision Float(number=w450) -> (double precision float=w452:dbl)
                n257 = case shown="False" w457 {
                  tunnel: [-1 ("index of element") w460] -> w458
                  tunnel: w453 -> [_ w460]
                  frame False {
                  }
                  frame True {
                  }
                }
                n258 = local write "Shot"(w451) -> ()
                n259 = local write "Panel"(w450) -> ()
                n260 = property on="Record #" class="DigNum (strict)"("Maximum"=w452) -> ()  [unwired: 2 in, 2 out]
              }
            }
          }
        }
      }
      frame 0 {
        # "INITIALIZE"
        # "This section reads the ini file"
        n261 = case shown="0, Default" w473 {
          tunnel: [w477 w482] -> w474
          tunnel: [w475 w482] -> w462
          frame 0, Default {
            n262 = local read "RESET All"() -> (w476:bool)
            n263 = case shown="True" w476 {
              tunnel: [TRUE w480] -> w477
              tunnel: [FALSE w480] -> w475
              frame False {
                # "Refresh"
              }
              frame True {
                n264 = Two Button Dialog(message="Reset will remove all unsaved data.  Do you want to RESET? ") -> (T button?=w480:bool)  [unwired: 2 in]
              }
            }
          }
          frame 100 {
            w482 = TRUE
          }
        }
        n265 = case shown="True" w474 {
          tunnel: w472 -> [w484 w505]
          tunnel: w471 -> [w483 w504]
          tunnel: [-1 ("index of element") w503] -> w470
          tunnel: w467 -> [w485 w501]
          tunnel: [w485 w500] -> w466
          tunnel: w461 -> [_ w499]
          tunnel: w465 -> [_ w498]
          tunnel: [w484 w493] -> w464
          tunnel: [w483 w490] -> w463
          tunnel: w462 -> [_ w488]
          frame False {
            n266 = local write "RESET All"(FALSE ("RESET")) -> ()
          }
          frame True {
            n267 = flat-sequence {
              tunnel: w498 -> [w508]
              tunnel: w499 -> [w511]
              tunnel: w501 -> [_]
              tunnel: w504 -> [w514]
              tunnel: w505 -> [w516]
              tunnel: [w506] -> w497
              tunnel: [w510] -> w496
              tunnel: [w507] -> w495
              tunnel: w488 -> [w517]
              tunnel: [w515] -> w492
              tunnel: [w513] -> w489
              tunnel: [w561] -> w502
              tunnel: w497 -> [w533]
              tunnel: w496 -> [w541]
              tunnel: w495 -> [w538]
              tunnel: [w533] -> w494
              tunnel: w492 -> [w536]
              tunnel: [w536] -> w491
              tunnel: w489 -> [w537]
              tunnel: [w601] -> w503
              tunnel: w502 -> [w601]
              tunnel: ["SHOTS"] -> w500
              tunnel: [w598] -> w493
              tunnel: w494 -> [w598]
              tunnel: [w597] -> w490
              tunnel: w491 -> [w597]
              frame #0 {
                n268 = case shown="True" w517 {
                  tunnel: [w520 w525] -> w506
                  tunnel: w516 -> [w520 _]
                  tunnel: [w519 w524] -> w515
                  tunnel: w514 -> [w519 _]
                  tunnel: [w518 w522] -> w513
                  frame False {
                    w518 = FALSE  # Reset All
                    # "Refresh"
                  }
                  frame True {
                    w522 = TRUE
                    # "Is the message center needed?"
                    # "This section resets\nentire program"
                    n269 = control-ref of="This VI"() -> (w529:refnum<vi>)
                    n270 = invoke class="VI" method="Default Vals.Reinit All"(reference=w529) -> (error out=w523:errorcluster)  [unwired: 2 in, 2 out]
                    n271 = call "Initialize (SubVI).vi"("error IN"=w523) -> ("appended path OUT"=w525:path, "connectString"=w524:string, "Database Connection"=→"dbConn":string, "Weight Units"=→"Weight Units":string, "Distance Units"=→"Distance Units":string)  [unwired: 2 in]
                    n272 = local write "message control"(FALSE ("message control")) -> ()
                    n273 = property on="minV50" class="DigNum (strict)"("Visible"=w522) -> ()  [unwired: 2 in, 2 out]
                  }
                }
                "configPath" <- w506
                n274 = control-ref of="fabStyle_0"() -> (w509:refnum<vi>)
                n275 = control-ref of="fabVendor_0"() -> (w512:refnum<vi>)
                n276 = Build Array (concatenate)(w509, w508) -> (w507:refnum<vi>[])
                n277 = Build Array (concatenate)(w512, w511) -> (w510:refnum<vi>[])
              }
              frame #1 {
                # "New for PBBA"
                n278 = call "Load Vendors.vi"("Vendor array"=w541, "connectString"=w536) -> ()  [unwired: 1 out]
                n279 = property on="connStr" class="Str"("Val(Sgnl)"=w536) -> ()  [unwired: 2 in, 2 out]
                n280 = control-ref of="ballistician"() -> (w553:refnum<vi>)
                n281 = control-ref of="Panel Technician"() -> (w552:refnum<vi>)
                n282 = control-ref of="Manufacturer"() -> (w551:refnum<vi>)
                n283 = control-ref of="Test Conditions"() -> (w550:refnum<vi>)
                n284 = control-ref of="Type"() -> (w549:refnum<vi>)
                n285 = call "Read INI Section 2.vi"("section"="Threat with Correction Factor", "configuration file path"=w533) -> ("Array"=w571:string[])  [unwired: 4 in, 1 out]
                n286 = control-ref of="Panel Backing"() -> (w542:refnum<vi>)
                n287 = control-ref of="Submitter"() -> (w543:refnum<vi>)
                n288 = control-ref of="Panel Dimensions"() -> (w544:refnum<vi>)
                n289 = control-ref of="Powder Type"() -> (w545:refnum<vi>)
                n290 = control-ref of="Panel Type"() -> (w546:refnum<vi>)
                n291 = control-ref of="Method"() -> (w547:refnum<vi>)
                n292 = control-ref of="Panel Stitch"() -> (w548:refnum<vi>)
                n293 = call "Get INI Section.vi"("Ring Refnum"=w553, "configuration file path"=w533) -> ()  [unwired: 4 in, 2 out]
                n294 = call "Get INI Section.vi"("Ring Refnum"=w552, "configuration file path"=w533) -> ()  [unwired: 4 in, 2 out]
                n295 = call "Get INI Section.vi"("Ring Refnum"=w551, "configuration file path"=w533) -> ()  [unwired: 4 in, 2 out]
                n296 = call "Get INI Section.vi"("Ring Refnum"=w550, "configuration file path"=w533) -> ()  [unwired: 4 in, 2 out]
                n297 = call "Get INI Section.vi"("Ring Refnum"=w549, "configuration file path"=w533) -> ()  [unwired: 4 in, 2 out]
                n298 = call "Split Factor Array.vi"("Split character"=":", "STRING INPUT"=w571) -> ("FACTOR OUTPUT"=→"factor array":sgl[], "STRING OUTPUT"=w569:string[])
                n299 = call "Read Parameters.vi"("appended path"=w533) -> ("midpt_to_target_dist"=→"mid_to_targ_dist":sgl, "max dev"=w565:sgl, "residual separation"=→"Residual/Separation":sgl, "impact separation"=→"Impact/Separation":sgl, "barrel screen dist"=→"Barrel to Screen":sgl, "impact target dist"=w564:sgl, "resid target dist"=w563:sgl)  [unwired: 3 in]
                n300 = call "Get INI Section.vi"("Ring Refnum"=w542, "configuration file path"=w533) -> ()  [unwired: 4 in, 2 out]
                n301 = call "Get INI Section.vi"("Ring Refnum"=w543, "configuration file path"=w533) -> ()  [unwired: 4 in, 2 out]
                n302 = call "Get INI Section.vi"("Ring Refnum"=w544, "configuration file path"=w533) -> ()  [unwired: 4 in, 2 out]
                n303 = call "Get INI Section.vi"("Ring Refnum"=w545, "configuration file path"=w533) -> ()  [unwired: 4 in, 2 out]
                n304 = call "Get INI Section.vi"("Ring Refnum"=w546, "configuration file path"=w533) -> ()  [unwired: 4 in, 2 out]
                n305 = call "Get INI Section.vi"("Ring Refnum"=w547, "configuration file path"=w533) -> ()  [unwired: 4 in, 2 out]
                n306 = call "Get INI Section.vi"("Ring Refnum"=w548, "configuration file path"=w533) -> ()  [unwired: 4 in, 2 out]
                n307 = property on="Threat 2" class="Ring (strict)"("Strings []"=w569) -> ()  [unwired: 2 in, 2 out]
                n308 = local write "Impact/Target Dist"(w564) -> ()
                n309 = local write "maxDev"(w565) -> ()
                n310 = local write "Residual/Target Dist"(w563) -> ()
                n311 = control-ref of="deployment"() -> (w531:refnum<vi>)
                n312 = Bundle("deployment"=w531) -> (w530:cluster{"deployment":refnum<vi>})  [unwired: 1 in]
                n313 = control-ref of="covering"() -> (w554:refnum<vi>)
                n314 = control-ref of="shooter"() -> (w555:refnum<vi>)
                n315 = control-ref of="recorder"() -> (w556:refnum<vi>)
                n316 = control-ref of="weapon"() -> (w557:refnum<vi>)
                n317 = control-ref of="Fabric.stitch"() -> (w540:refnum<vi>)
                n318 = control-ref of="Model"() -> (w534:refnum<vi>)
                n319 = call "Initialize Variables.vi"("subkey"="Software\\DuPont\\BIMS", "InitCluster"=w530) -> ()  [unwired: 7 in, 1 out]
                n320 = case shown="True" w537 {
                  tunnel: [errorcluster {"status"=FALSE, "code"=0, "source"=""} ("error out") w587] -> w562
                  tunnel: [-1 ("index of element") w585] -> w561
                  tunnel: w536 -> [_ w584]
                  tunnel: w538 -> [_ w581]
                  frame False {
                    # "Refresh"
                  }
                  frame True {
                    w583 = u8 2 ("Disabled")
                    n321 = control-ref of="projectileType"() -> (w577:refnum<vi>)
                    n322 = local read "Data Source"() -> (w586:u16)
                    n323 = call "Get Last Record (SubVI).vi"("connect Str"=w584) -> ("shot record"=→"Shot":i32, "experiment record"=w579:i32, "error out"=w587:errorcluster)
                    "Panel" <- w579
                    n324 = Build Array (concatenate)(w581, w577) -> (w580:refnum<vi>[])
                    n325 = for {
                      tunnel: w580 -> [w589] mode=indexing
                      n326 = property class="Ring (strict)"(reference=w589, "Strings []"=string[] []) -> ()  [unwired: 1 in, 2 out]
                    }
                    n327 = To Double Precision Float(number=w579) -> (double precision float=w578:dbl)
                    n328 = case shown="2" w586 {
                      tunnel: [-1 ("index of element") -1 ("index of element") 7 ("index of element") -1 ("index of element")] -> w585
                      frame 0, Default {
                        # "Simulated"
                      }
                      frame 1 {
                        # "Radar"
                      }
                      frame 2 {
                        # "check for\nPCI 6602"
                      }
                      frame 3 {
                        # "Manual"
                      }
                    }
                    n329 = property on="Accept Data" class="Bool (strict)"("Disabled"=u8 0) -> ()  [unwired: 2 in, 2 out]
                    n330 = property on="Reject shot" class="Bool"("Disabled"=w583) -> ()  [unwired: 2 in, 2 out]
                    n331 = property on="Save" class="Bool"("Disabled"=w583) -> ()  [unwired: 2 in, 2 out]
                    n332 = property on="Clear" class="Bool"("Disabled"=w583) -> ()  [unwired: 2 in, 2 out]
                    n333 = property on="Record #" class="DigNum (strict)"("Maximum"=w578) -> ()  [unwired: 2 in, 2 out]
                  }
                }
                n334 = call "Get INI Section.vi"("Ring Refnum"=w554, "configuration file path"=w533) -> ()  [unwired: 4 in, 2 out]
                n335 = call "Get INI Section.vi"("Ring Refnum"=w555, "configuration file path"=w533) -> ()  [unwired: 4 in, 2 out]
                n336 = call "Get INI Section.vi"("Ring Refnum"=w556, "configuration file path"=w533) -> ()  [unwired: 4 in, 2 out]
                n337 = call "Get INI Section.vi"("Ring Refnum"=w557, "configuration file path"=w533) -> ()  [unwired: 4 in, 2 out]
                n338 = call "Get INI Section.vi"("Ring Refnum"=w540, "configuration file path"=w533) -> ()  [unwired: 4 in, 2 out]
                n339 = call "Get INI Section.vi"("Ring Refnum"=w534, "configuration file path"=w533) -> ()  [unwired: 4 in, 2 out]
                n340 = Path To String(path=w533) -> (string=w566:string)
                n341 = case shown="True" "message control" {
                  tunnel: w562 -> [_ _]
                  tunnel: w566 -> [_ w573]
                  frame False {
                  }
                  frame True {
                    n342 = local write "message control"(FALSE) -> ()
                    n343 = call "Ballistics Message Center.vi"("INI File Name"=w573) -> ()
                  }
                }
                n344 = control-ref of="projectileWt"() -> (w539:refnum<vi>)
                n345 = call "Load Threats.vi"("projectileWt"=w539, "connectString"=w536) -> ()  [unwired: 1 out]
                "connStr" <- w536
              }
              frame #2 {
                n346 = property on="rangeSetup" class="Ring (strict)"("Val(Sgnl)"=u16 0 ("Value (Signaling)")) -> ()  [unwired: 2 in, 2 out]
                n347 = property on="workType" class="Ring (strict)"("Val(Sgnl)"=u16 0 ("Value (Signaling)")) -> ()  [unwired: 2 in, 2 out]
                n348 = One Button Dialog(message="Ready") -> ()  [unwired: 1 in, 1 out]
              }
            }
          }
        }
      }
      frame 1 {
        w661 = TRUE  # append on new line? (F)
        w701 = TRUE  # append on new line? (F)
        w733 = FALSE  # show grid lines
        w745 = -1 ("index of element")
        # "DUPONT V50 REPORT"
        # "This section prepares a DuPont V50 report (HTML)"
        # "add graph to 3rd box"
        n349 = invoke on="Shot Graph" class="XYGraph (strict)" method="Reinit To Default"() -> (error out=w714:errorcluster)  [unwired: 3 in, 2 out]
        n350 = property on="Submitter" class="Ring (strict)"() -> ("Strings []"=w648:string[], "Value"=w647:u16)  [unwired: 2 in, 2 out]
        n351 = control-ref of="Complete"() -> (w622:refnum<vi>)
        n352 = control-ref of="Points"() -> (w711:refnum<vi>)
        n353 = control-ref of="Partial"() -> (w710:refnum<vi>)
        n354 = To Long Integer(number=w647) -> (32bit integer=w621:i32)
        n355 = control-ref of="Value"() -> (w712:refnum<vi>)
        n356 = call "Graph V50.vi"("valueRef"=w712, "completeRef"=w622, "pointsRef"=w711, "partialRef"=w710, "error IN"=w714) -> ("shotGraph"=→"Shot Graph":cluster{i32[], sgl[]}[])
        n357 = Index Array(array=w648, index=w621) -> (element=w644:string)
        n358 = call <vilib>:"New Report.vi"("report type"=T12."HTML", "error in (no error)"=w714) -> ("report out"=w735:refnum<class "NI_report.lvclass">, "error out"=w734:errorcluster)  [unwired: 12 in]
        n359 = local read "Panel"() -> (w643:i32)
        n360 = Format Into String(format string="Serial Number: %5d<newline>Submitter: %s" ("Format String"), w643, w644) -> (resulting string=w642:string)  [unwired: 2 in, 1 out]
        n361 = call-dynamic "Set Report Font.vi"("report in"=w735, "text options"=T11 {"Italic"=enum."Italic Unchanged", "Strike Through"=enum."Strike Through Unchanged", "Underline"=enum."Underline Unchanged", "Bold"=enum."Bold On"}, "font settings"=T10 {"Charset (-1)"=-1, "Weight (-1)"=-1, "Name"="Arial", "Size"="4 "}, "error in (no error)"=w734) -> ("report out"=w719:refnum<class "NI_report.lvclass">, "error out"=w720:errorcluster)  [unwired: 9 in, 1 out]
        n362 = call-dynamic "Set Report Header Text.vi"("report in"=w719, "left header text"=w642, "center header text"="Ballistic V50 Report", "error in (no error)"=w720, "HTML header size"=enum16{"H1", "H2", "H3", "H4", "H5", "H6", "H7"}."H2") -> ("report out"=w722:refnum<class "NI_report.lvclass">, "error out"=w723:errorcluster)  [unwired: 9 in]
        n363 = local read "Fabric Description"() -> (w673:string)
        n364 = local read "Impact factor"() -> (w670:sgl)
        n365 = local read "Projectile Mass"() -> (w627:sgl)
        n366 = property on="Manufacturer" class="Ring (strict)"() -> ("Strings []"=w680:string[], "Value"=w679:u16)  [unwired: 2 in, 2 out]
        n367 = property on="Panel Backing" class="Ring (strict)"() -> ("Strings []"=w678:string[], "Value"=w677:u16)  [unwired: 2 in, 2 out]
        n368 = property on="Powder Type" class="Ring (strict)"() -> ("Strings []"=w676:string[], "Value"=w675:u16)  [unwired: 2 in, 2 out]
        n369 = property on="Threat 2" class="Ring (strict)"() -> ("Strings []"=w672:string[], "Value"=w671:u16)  [unwired: 2 in, 2 out]
        n370 = local read "RoomT"() -> (w629:sgl)
        n371 = call-dynamic "Set Report Font.vi"("report in"=w722, "text options"=T11 {"Italic"=enum."Italic Unchanged", "Strike Through"=enum."Strike Through Unchanged", "Underline"=enum."Underline Unchanged", "Bold"=enum."Bold Off"}, "font settings"=T10 {"Charset (-1)"=-1, "Weight (-1)"=-1, "Name"="Arial", "Size"="1"}, "error in (no error)"=w723) -> ("report out"=w698:refnum<class "NI_report.lvclass">, "error out"=w699:errorcluster)  [unwired: 9 in, 1 out]
        n372 = Select(t="Disclosure on Ballistic and Stab Test Data<newline>The attached ballistic test data was generated by DuPont and corresponds to DuPont's current knowledge on the performance of the subject test panels against certain ballistic threats.  This information is offered solely to provide possible suggestions for your own experimentation and validation.  It is not intended as a substitute for your own testing or any testing you may need to submit for a bid package, you should undertake your own testing whether you do so yourself with the supplier of the materials to be tested or with an independent, third party, certified testing facility and the supplier of the materials to be tested (i.e., the fabric weaver).  DuPont makes no warranties, and assumes no liabilities in connection with any use of the information supplied with this disclosure statement." ("text"), s="Add Disclaimer", f="" ("t")) -> (s? t:f=w657:string)
        n373 = To Long Integer(number=w679) -> (32bit integer=w610:i32)
        n374 = To Long Integer(number=w677) -> (32bit integer=w613:i32)
        n375 = To Long Integer(number=w675) -> (32bit integer=w612:i32)
        n376 = To Long Integer(number=w671) -> (32bit integer=w611:i32)
        n377 = Index Array(array=w680, index=w610) -> (element=w674:string)
        n378 = call-poly <vilib>:"Append Report Text.vi"("report in"=w698, "text"=w657, "error in (no error)"=w699) -> ("report out"=w697:refnum<class "NI_report.lvclass">, "error out"=w695:errorcluster)  [unwired: 9 in, 2 out]
        n379 = Index Array(array=w678, index=w613) -> (element=w626:string)
        n380 = Index Array(array=w676, index=w612) -> (element=w664:string)
        n381 = Index Array(array=w672, index=w611) -> (element=w632:string)
        n382 = property on="Test Conditions" class="Ring (strict)"() -> ("Strings []"=w669:string[], "Value"=w668:u16)  [unwired: 2 in, 2 out]
        n383 = property on="Panel Type" class="Ring (strict)"() -> ("Strings []"=w667:string[], "Value"=w666:u16)  [unwired: 2 in, 2 out]
        n384 = call-dynamic "Set Report Font.vi"("report in"=w697, "text options"=T11 {"Italic"=enum."Italic Unchanged", "Strike Through"=enum."Strike Through Unchanged", "Underline"=enum."Underline Unchanged", "Bold"=enum."Bold Unchanged"}, "font settings"=T10 {"Charset (-1)"=-1, "Weight (-1)"=-1, "Name"="Arial", "Size"="3 "}, "error in (no error)"=w695) -> ("report out"=w696:refnum<class "NI_report.lvclass">, "error out"=w694:errorcluster)  [unwired: 9 in, 1 out]
        n385 = local read "Z.M.R."() -> (w655:sgl)
        n386 = local read "Areal Density"() -> (w625:dbl)
        n387 = local read "Weight of Panel"() -> (w628:dbl)
        n388 = local read "Sample #"() -> (w624:string)
        n389 = local read "Shot Angle"() -> (w663:u16)
        n390 = local read "RoomHum"() -> (w631:sgl)
        n391 = call-dynamic "New Report Line.vi"("report in"=w696, "error in (no error)"=w694) -> ("report out"=w736:refnum<class "NI_report.lvclass">, "error out"=w737:errorcluster)  [unwired: 12 in]
        n392 = To Long Integer(number=w668) -> (32bit integer=w609:i32)
        n393 = To Long Integer(number=w666) -> (32bit integer=w608:i32)
        n394 = Index Array(array=w669, index=w609) -> (element=w662:string)
        n395 = call-dynamic "New Report Line.vi"("report in"=w736, "error in (no error)"=w737) -> ("report out"=w703:refnum<class "NI_report.lvclass">, "error out"=w702:errorcluster)  [unwired: 12 in]
        n396 = Index Array(array=w667, index=w608) -> (element=w630:string)
        n397 = Format Into String(format string="<table border=\"0\" cellspacing=\"6\"><tr><td align=\"left\"><b>Fabric Parameters</b></td><td>&nbsp;</td><td>&nbsp;</td><td align=\"left\"><b>Test Parameters</b></td><td>&nbsp;</td></tr><tr><td align=\"right\">Sample ID: </td><td align=\"left\">%s</td><td>&nbsp;</td><td align=\"right\">Method: </td><td align=\"left\">V50</td></tr><tr><td align=\"right\">Areal Density: </td><td align=\"left\">%.3f</td><td>&nbsp;</td><td align=\"right\">Threat: </td><td align=\"left\">%s</td></tr><tr><td align=\"right\">Manufacturer: </td><td align=\"left\">%s</td><td>&nbsp;</td><td align=\"right\">Room Temperature: </td><td align=\"left\">%.0f</td></tr><tr><td align=\"right\">Group Data: </td><td align=\"left\">%s</td><td>&nbsp;</td><td align=\"right\">Correction Factor: </td><td align=\"left\">%0.4f</td></tr><tr><td align=\"right\">Projectile Weight: </td><td align=\"left\">%0.3f</td><td>&nbsp;</td><td align=\"right\">Panel Backing: </td><td align=\"left\">%s</td></tr><tr><td align=\"right\">Powder Type: </td><td align=\"left\">%s</td><td>&nbsp;</td><td align=\"right\">Shot Angle: </td><td align=\"left\">%.0f</td></tr><tr><td align=\"right\">Test Conditions: </td><td align=\"left\">%s</td><td>&nbsp;</td><td align=\"right\">Room Humidity: </td><td align=\"left\">%.0f</td></tr><tr><td align=\"right\">Panel Weight: </td><td align=\"left\">%.4f</td><td>&nbsp;</td><td>&nbsp;</td></tr><tr><td align=\"right\">Descripton: </td><td align=\"left\">%s</td><td>&nbsp;</td><td>&nbsp;</td></tr></table>", w624, w625, w632, w674, w629, w673, w670, w627, w626, w664, w663, w662, w631, w628, w630) -> (resulting string=w659:string)  [unwired: 2 in, 1 out]
        n398 = property on="ballistician" class="Ring (strict)"() -> ("Strings []"=w684:string[], "Value"=w683:u16)  [unwired: 2 in, 2 out]
        n399 = call-poly <vilib>:"Append Report Text.vi"("report in"=w703, "text"=w659, "append on new line? (F)"=w701, "error in (no error)"=w702) -> ("report out"=w636:refnum<class "NI_report.lvclass">, "error out"=w637:errorcluster)  [unwired: 8 in, 2 out]
        n400 = To Long Integer(number=w683) -> (32bit integer=w607:i32)
        n401 = call-dynamic "New Report Line.vi"("report in"=w636, "error in (no error)"=w637) -> ("report out"=w730:refnum<class "NI_report.lvclass">, "error out"=w731:errorcluster)  [unwired: 12 in]
        n402 = local read "computed_V50"() -> (w700:sgl)
        n403 = Get Date/Time String(date format (0)=enum16{"short", "long", "abbreviated"}."abbreviated") -> (date string=w691:string)  [unwired: 2 in, 1 out]
        n404 = Index Array(array=w684, index=w607) -> (element=w682:string)
        n405 = local read "Sample #"() -> (w646:string)
        n406 = property on="Table of Shots" class="Tbl (strict)"() -> ("Column Header Strings[]"=w713:string[])  [unwired: 2 in, 2 out]
        n407 = Less Than 0?(x=w655) -> (x < 0?=w656:bool)
        n408 = call-dynamic "New Report Line.vi"("report in"=w730, "error in (no error)"=w731) -> ("report out"=w729:refnum<class "NI_report.lvclass">, "error out"=w728:errorcluster)  [unwired: 12 in]
        n409 = Concatenate Strings(w691, " © " ("right footer text"), "  DuPont ") -> (w707:string)
        n410 = local read "Pairs"() -> (w681:i16)
        n411 = Select(t="Low Complete-High Partial: ", s=w656, f="Zone of Mixed Results: ") -> (s? t:f=w651:string)
        n412 = Format Value(format string="Panel %s.html  " ("string (\"\")"), value (0)=w646) -> (output string=w706:string)  [unwired: 1 in]
        n413 = call-poly <vilib>:"Append Table to Report.vi"("report in"=w729, "column width (1)"=1.1, "column headers"=w713, "text data"="Table of Shots", "error in (no error)"=w728, "show grid lines"=w733) -> ("report out"=w685:refnum<class "NI_report.lvclass">, "error out"=w689:errorcluster)  [unwired: 6 in, 2 out]
        n414 = Build Path(base path="Report Path", name or relative path=w706) -> (appended path=w704:path)
        n415 = Concatenate Strings(" V50:  %10.1f<newline>Number of Pairs Used: %d<newline>  ", w651, "%.1f<newline><newline>Ballistician:%s<newline> ") -> (w649:string)
        n416 = Format Into String(format string=w649, w700, w681, w655, w682) -> (resulting string=w620:string)  [unwired: 2 in, 1 out]
        n417 = call-dynamic "Set Report Font.vi"("report in"=w685, "text options"=T11 {"Italic"=enum."Italic Unchanged", "Strike Through"=enum."Strike Through Unchanged", "Underline"=enum."Underline On", "Bold"=enum."Bold Off"}, "font settings"=T10 {"Charset (-1)"=-1, "Weight (-1)"=-1, "Name"="Arial", "Size"="3 "}, "error in (no error)"=w689) -> ("report out"=w686:refnum<class "NI_report.lvclass">, "error out"=w687:errorcluster)  [unwired: 9 in, 1 out]
        n418 = call-dynamic "New Report Line.vi"("report in"=w686, "error in (no error)"=w687) -> ("report out"=w727:refnum<class "NI_report.lvclass">, "error out"=w726:errorcluster)  [unwired: 12 in]
        n419 = control-ref of="Shot Graph"() -> (w660:refnum<vi>)
        n420 = call-poly <vilib>:"Append Report Text.vi"("report in"=w727, "text"=w620, "append on new line? (F)"=w661, "error in (no error)"=w726) -> ("report out"=w634:refnum<class "NI_report.lvclass">, "error out"=w633:errorcluster)  [unwired: 8 in, 2 out]
        n421 = call-dynamic "Append Control Image to Report.vi"("report in"=w634, "image file type (.jpg)"=enum16{".jpg", ".png"}.".jpg" ("image file type(.png)"), "ctrl reference"=w660, "description"="Graph of Test Results" ("control name"), "error in (no error)"=w633) -> ("report out"=w619:refnum<class "NI_report.lvclass">, "error out"=w618:errorcluster)  [unwired: 7 in, 2 out]
        n422 = call-dynamic "Set Report Footer Text.vi"("report in"=w619, "right footer text"=w707, "error in (no error)"=w618) -> ("report out"=w724:refnum<class "NI_report.lvclass">, "error out"=w725:errorcluster)  [unwired: 11 in]
        n423 = call-dynamic "Get Report Type.vi"("report in"=w724, "error in (no error)"=w725) -> ("report out"=w741:refnum<class "NI_report.lvclass">, "report type"=w740:T12, "error out"=w744:errorcluster)  [unwired: 11 in]
        n424 = case shown="\"Standard Report\", Default" w740 {
          tunnel: w741 -> [w750 w755 w757 w759]
          tunnel: [w749 w754 w757 w759] -> w742
          tunnel: [w748 w753 w756 w758] -> w743
          tunnel: w744 -> [w747 w752 w756 w758]
          tunnel: w704 -> [_ w751 _ _]
          frame "Standard Report", Default {
            n425 = call-dynamic "Print Report.vi"("report in"=w750, "error in (no error)"=w747) -> ("report out"=w749:refnum<class "NI_report.lvclass">, "error out"=w748:errorcluster)  [unwired: 12 in]
          }
          frame "HTML" {
            n426 = call-dynamic "Save Report to File.vi"("report in"=w755, "report file path"=w751, "error in (no error)"=w752) -> ("report out"=w754:refnum<class "NI_report.lvclass">, "error out"=w753:errorcluster)  [unwired: 11 in]
          }
          frame "Word" {
          }
          frame "Excel" {
          }
        }
        n427 = call-dynamic "Dispose Report.vi"("report in"=w742, "error in (no error)"=w743) -> ("error out"=w638:errorcluster)  [unwired: 13 in]
        n428 = call <vilib>:"Simple Error Handler.vi"("error in (no error)"=w638) -> ("error out"=w639:errorcluster)  [unwired: 4 in, 4 out]
        n429 = case shown="No Error" w639 {
          frame No Error {
            n430 = One Button Dialog(message="A V50 Report is ready.") -> ()  [unwired: 1 in, 1 out]
          }
          frame Error {
          }
        }
      }
      frame 2 {
        w794 = TRUE  # Enable
        w797 = -1 ("index of element")
        # "DHB BALLISTIC TEST REPORT"
        # "The custom Excel template file is \nexpected in the C:\\Ballistics folder."
        # "Create DHB Ballistic Test Report"
        n431 = case shown="False" "lookupRec" {
          selector: "lookupRec" -> [_ w1079]
          tunnel: [w815 w1058] -> w792
          tunnel: [w814 w1042] -> w791
          tunnel: [w813 w1062] -> w790
          tunnel: [w812 w1067] -> w789
          tunnel: [w811 w1060] -> w788
          tunnel: [w810 w1064] -> w787
          tunnel: w773 -> [w809 _]
          tunnel: w772 -> [w808 _]
          tunnel: w771 -> [w807 _]
          tunnel: w770 -> [w806 _]
          tunnel: [w805 w1070] -> w769
          tunnel: [w804 w1074] -> w768
          tunnel: [w803 w1073] -> w767
          tunnel: [w802 "Record #"] -> w766
          tunnel: [w801 w1061] -> w765
          tunnel: [w800 w1072] -> w764
          tunnel: w761 -> [_ w1059]
          tunnel: w760 -> [w799 _]
          frame False {
            n432 = stacked-sequence {
              tunnel: [_ _ _ _ _ w1002 _] -> w810
              tunnel: [_ w878 _ _ _ _ _] -> w814
              tunnel: [_ _ _ _ w961 _ _] -> w811
              tunnel: [_ _ _ w927 _ _ _] -> w812
              tunnel: [_ _ w899 _ _ _ _] -> w813
              tunnel: [w820 _ _ _ _ _ _] -> w815
              tunnel: w808 -> [w819 _ _ _ _ _ _]
              tunnel: w809 -> [w818 _ _ _ _ _ _]
              tunnel: w807 -> [w817 _ _ _ _ _ _]
              tunnel: w806 -> [w816 _ _ _ _ _ _]
              tunnel: [_ _ _ _ _ _ w1027] -> w805
              tunnel: [_ _ _ _ _ _ w1026] -> w804
              tunnel: [_ _ _ _ _ _ w1025] -> w803
              tunnel: [_ _ _ _ _ _ w1024] -> w802
              tunnel: [_ _ _ _ _ _ w1023] -> w801
              tunnel: [_ _ _ _ _ _ w1022] -> w800
              tunnel: w799 -> [_ _ w898 _ w954 _ _]
              tunnel: "Method" -> [_ _ w889 _ w953 _ _]
              frame #0 {
                # "FABRIC"
                n433 = local read "fab1_totalWt"() -> (w823:sgl)
                n434 = local read "fab3_totalWt"() -> (w825:sgl)
                n435 = local read "fab5_totalWt"() -> (w827:sgl)
                n436 = local read "fab2_totalWt"() -> (w824:sgl)
                n437 = local read "fab4_totalWt"() -> (w826:sgl)
                n438 = local read "fab6_totalWt"() -> (w828:sgl)
                n439 = Build Array(w823, w824, w825, w826, w827, w828) -> (w822:sgl[])
                n440 = for {
                  tunnel: w822 -> [w829] mode=indexing
                  tunnel: [w836] -> w821 mode=indexing
                  tunnel: w818 -> [w834] mode=indexing
                  tunnel: w819 -> [w833] mode=indexing
                  tunnel: w817 -> [w832] mode=indexing
                  tunnel: w816 -> [w831] mode=indexing
                  n441 = Unbundle By Name(w833) -> ("plyNum"=w830:i32)
                  n442 = Less Or Equal To 0?(x=w829) -> (x <= 0?=w835:bool)
                  n443 = case shown="True" w835 {
                    tunnel: [w860 w862] -> w836
                    tunnel: w829 -> [w859 _]
                    tunnel: w834 -> [w855 _]
                    tunnel: w833 -> [w854 _]
                    tunnel: w832 -> [w847 _]
                    tunnel: w831 -> [w844 _]
                    tunnel: w830 -> [w840 _]
                    frame False {
                      n444 = Unbundle By Name(w855) -> ("fabricID_DHB"=w841:string, "Fabric.fiber"=w842:string, "Fabric.denier"=w849:string, "pick"=w848:string, "weave"=w837:string, "finish"=w838:string, "ozPerYd2"=w852:string)
                      n445 = Unbundle By Name(w854) -> ("LotNum"=w850:string, "RollNum"=w851:string, "Fabric.stitch"=w853:u16)
                      n446 = Format Into String(w840) -> (resulting string=w846:string)  [unwired: 3 in, 1 out]
                      n447 = To Long Integer(number=w853) -> (32bit integer=w858:i32)
                      n448 = call "Dropdown Selection (SubVI).vi"("reference"=w847) -> ("element"=w845:string)
                      n449 = call "Dropdown Selection (SubVI).vi"("reference"=w844) -> ("element"=w843:string)
                      n450 = property on="Fabric.stitch" class="Ring (strict)"() -> ("Strings []"=w839:string[])  [unwired: 2 in, 2 out]
                      n451 = Index Array(array=w839, index=w858) -> (element=w856:string)
                      n452 = Format Into String(w859) -> (resulting string=w857:string)  [unwired: 3 in, 1 out]
                      n453 = Build Array(w846, w845, w843, w841, w842, w849, w848, w837, w838, w850, w851, w852, w857, w856) -> (w860:string[])
                    }
                    frame True {
                      n454 = call <vilib>:"Space Constant.vi"() -> ("String"=w863:string)
                      n455 = Initialize Array(w863, 12 ("dimension size")) -> (w862:string[])
                    }
                  }
                }
                n456 = Transpose 2D Array(2D array=w821) -> (transposed array=w820:string[][])
              }
              frame #1 {
                w864 = "%.1f" ("format string")
                # "muzzel / midpoint"
                # "muzzle / scr#1"
                # "muzzle / target"
                # "scr#2 / target"
                # "RANGE"
                n457 = local read "Impact/Separation"() -> (w871:sgl)
                n458 = local read "mid_to_targ_dist"() -> (w868:sgl)
                n459 = local read "Barrel to Screen"() -> (w865:sgl)
                n460 = Divide(x=w871, y=sgl 2.0) -> (x/y=w866:sgl)
                n461 = local read "clayAverage"() -> (w886:sgl)
                n462 = local read "RoomHum"() -> (w881:sgl)
                n463 = local read "clayTemp"() -> (w884:sgl)
                n464 = local read "clayCalib"() -> (w887:string)
                n465 = local read "RoomT"() -> (w882:sgl)
                n466 = Add(x=w865, y=w868) -> (x+y=w872:sgl)
                n467 = Subtract(x=w865, y=w866) -> (x-y=w867:sgl)
                n468 = Subtract(x=w868, y=w866) -> (x-y=w869:sgl)
                n469 = Format Into String(w872) -> (resulting string=w873:string)  [unwired: 3 in, 1 out]
                n470 = Format Into String(w867) -> (resulting string=w874:string)  [unwired: 3 in, 1 out]
                n471 = Format Into String(w871) -> (resulting string=w875:string)  [unwired: 3 in, 1 out]
                n472 = Format Into String(w869) -> (resulting string=w876:string)  [unwired: 3 in, 1 out]
                n473 = Format Into String(w868) -> (resulting string=w877:string)  [unwired: 3 in, 1 out]
                n474 = Format Into String(w881) -> (resulting string=w879:string)  [unwired: 3 in, 1 out]
                n475 = Format Into String(format string=w864, w882) -> (resulting string=w880:string)  [unwired: 2 in, 1 out]
                n476 = Format Into String(format string=w864, w884) -> (resulting string=w883:string)  [unwired: 2 in, 1 out]
                n477 = Format Into String(format string=w864, w886) -> (resulting string=w885:string)  [unwired: 2 in, 1 out]
                n478 = Bundle(w873, w874, w875, w876, w877, w879, w880, w883, "clayCalib"=w887, w885) -> (w888:T16)  [unwired: 1 in]
                n479 = Cluster To Array(cluster=w888) -> (array=w878:string[])
              }
              frame #2 {
                # "RESULTS"
                n480 = for {
                  tunnel: w898 -> [w926] mode=indexing
                  tunnel: [w925] -> w897 mode=indexing
                  tunnel: [w924] -> w896
                  i -> [w924]
                  n481 = Unbundle By Name(w926) -> ("BackFace\nDepth"=w925:sgl)
                }
                n482 = Increment(x=w896) -> (x+1=w894:i32)
                n483 = Add Array Elements(numeric array=w897) -> (sum=w895:sgl)
                n484 = To Single Precision Float(number=w894) -> (single precision float=w893:sgl)
                n485 = Divide(x=w895, y=w893) -> (x/y=w892:sgl)
                n486 = Format Into String(format string="%1.1f", w892) -> (resulting string=w891:string)  [unwired: 2 in, 1 out]
                n487 = case shown="0, Default" w889 {
                  tunnel: [w914 w923] -> w901
                  tunnel: w891 -> [w902 w922]
                  frame 0, Default {
                    w908 = "%1d" ("format string")
                    n488 = local read "Z.M.R."() -> (w906:sgl)
                    n489 = Less Than 0?(x=w906) -> (x < 0?=w907:bool)
                    n490 = local read "rangeOfResults"() -> (w910:i32)
                    n491 = local read "computed_V50"() -> (w913:sgl)
                    n492 = local read "lowComplete"() -> (w911:i32)
                    n493 = local read "highPartial"() -> (w912:i32)
                    n494 = case shown="True" w907 {
                      tunnel: w906 -> [w919 _]
                      tunnel: [w919 sgl 0.0 ("Z.M.R.")] -> w905
                      frame False {
                      }
                      frame True {
                      }
                    }
                    n495 = Format Into String(format string="%1.1f", w913) -> (resulting string=w917:string)  [unwired: 2 in, 1 out]
                    n496 = Format Into String(format string=w908, w912) -> (resulting string=w916:string)  [unwired: 2 in, 1 out]
                    n497 = Format Into String(format string=w908, w911) -> (resulting string=w915:string)  [unwired: 2 in, 1 out]
                    n498 = Format Into String(format string=w908, w910) -> (resulting string=w918:string)  [unwired: 2 in, 1 out]
                    n499 = Format Into String(format string="%1.1f", w905) -> (resulting string=w904:string)  [unwired: 2 in, 1 out]
                    n500 = Bundle(w917, w916, w915, w918, w904, w902, w902) -> (w914:T17)  [unwired: 1 in]
                  }
                  frame 1, 2 {
                    w921 = ""
                    n501 = Bundle(w921, w921, w921, w921, w921, w922, w922) -> (w923:T17)  [unwired: 1 in]
                  }
                }
                n502 = Cluster To Array(cluster=w901) -> (array=w900:string[])
                n503 = Build Array(w900) -> (w899:string[][])
              }
              frame #3 {
                # "SAMPLE"
                n504 = control-ref of="Method"() -> (w928:refnum<vi>)
                n505 = call "Dropdown Selection (SubVI).vi"("reference"=w928) -> ("element"=w930:string)
                n506 = Equal?(x=w930, y="V50") -> (x = y?=w929:bool)
                n507 = local read "totalSampleWt"() -> (w940:sgl)
                n508 = case shown="True" w929 {
                  tunnel: ["n/a" w952] -> w934
                  frame False {
                  }
                  frame True {
                    n509 = local read "minV50"() -> (w951:i32)
                    n510 = Format Into String(w951) -> (resulting string=w952:string)  [unwired: 3 in, 1 out]
                  }
                }
                n511 = control-ref of="Panel Dimensions"() -> (w947:refnum<vi>)
                n512 = control-ref of="workType"() -> (w948:refnum<vi>)
                n513 = control-ref of="covering"() -> (w949:refnum<vi>)
                n514 = control-ref of="Model"() -> (w933:refnum<vi>)
                n515 = local read "Sample #"() -> (w945:string)
                n516 = local read "serialNum"() -> (w942:string)
                n517 = local read "Thickness"() -> (w937:dbl)
                n518 = local read "totalBAW"() -> (w936:sgl)
                n519 = call "Dropdown Selection (SubVI).vi"("reference"=w947) -> ("element"=w944:string)
                n520 = call "Dropdown Selection (SubVI).vi"("reference"=w948) -> ("element"=w943:string)
                n521 = call "Dropdown Selection (SubVI).vi"("reference"=w933) -> ("element"=w932:string)
                n522 = call "Dropdown Selection (SubVI).vi"("reference"=w949) -> ("element"=w941:string)
                n523 = Format Into String(w940) -> (resulting string=w939:string)  [unwired: 3 in, 1 out]
                n524 = Format Into String(w937) -> (resulting string=w938:string)  [unwired: 3 in, 1 out]
                n525 = Format Into String(w936) -> (resulting string=w935:string)  [unwired: 3 in, 1 out]
                n526 = Bundle("Sample #"=w945, "element"=w944, "element"=w943, "serialNum"=w942, "element"=w932, w939, w938, w935, "element"=w941, w934) -> (w946:T18)  [unwired: 1 in]
                n527 = Cluster To Array(cluster=w946) -> (array=w927:string[])
              }
              frame #4 {
                # "SHOT TABLE"
                n528 = for {
                  tunnel: w954 -> [w993] mode=indexing
                  shift-right: [w970] -> _
                  shift-left: T13 [] -> [w972]
                  tunnel: [w970] -> w957
                  tunnel: w953 -> [w966]
                  n529 = Unbundle By Name(w993) -> ("shot order"=w992:i32, "Powder Loading"=w991:sgl, "Uncorrected Impact"=w990:sgl, "UncorrectedRed_PB"=w989:sgl, "UncorrectedAvgVel_PB"=w988:sgl, "velLoss_PB"=w987:sgl, "strikeVel_PB"=w986:sgl, "SHOT STATUS"=w975:u16, "usedv50"=w985:bool, "Shot Angle"=w967:u16, "BackFace\nDepth"=w968:sgl)
                  n530 = case shown="0, Default" w966 {
                    tunnel: w985 -> [w995 _]
                    tunnel: [w994 w999] -> w984
                    tunnel: w967 -> [_ w998]
                    frame 0, Default {
                      n531 = case shown="True" w995 {
                        tunnel: ["" ("Empty String Constant") "*"] -> w994
                        frame False {
                        }
                        frame True {
                        }
                      }
                    }
                    frame 1, 2 {
                      n532 = Format Into String(w998) -> (resulting string=w999:string)  [unwired: 3 in, 1 out]
                    }
                  }
                  n533 = case shown="1" w975 {
                    tunnel: ["P" "C"] -> w974
                    frame 0, Default {
                    }
                    frame 1 {
                    }
                  }
                  n534 = Format Into String(format string="%2d", w992) -> (resulting string=w977:string)  [unwired: 2 in, 1 out]
                  n535 = Format Into String(w991) -> (resulting string=w978:string)  [unwired: 3 in, 1 out]
                  n536 = Format Into String(w990) -> (resulting string=w979:string)  [unwired: 3 in, 1 out]
                  n537 = Format Into String(w989) -> (resulting string=w980:string)  [unwired: 3 in, 1 out]
                  n538 = Format Into String(w988) -> (resulting string=w981:string)  [unwired: 3 in, 1 out]
                  n539 = Format Into String(w987) -> (resulting string=w982:string)  [unwired: 3 in, 1 out]
                  n540 = Format Into String(w986) -> (resulting string=w983:string)  [unwired: 3 in, 1 out]
                  n541 = Format Into String(w968) -> (resulting string=w976:string)  [unwired: 3 in, 1 out]
                  n542 = Build Array(w977, w978, w979, w980, w981, w982, w983, w974, w984, w976) -> (w971:string[])
                  n543 = Array To Cluster(array=w971) -> (cluster=w973:T19)
                  n544 = Build Array (concatenate)(w972, w973) -> (w970:T13)
                }
                n545 = Array Size(array=w957) -> (size(s)=w959:i32)
                n546 = Equal To 0?(x=w959) -> (x = 0?=w955:bool)
                n547 = case shown="True" w955 {
                  tunnel: [w962 T13 [{"[0]"="", "[1]"="", "[2]"="", "[3]"="", "[4]"="", "[5]"="", "[6]"="", "[7]"="", "[8]"="", "[9]"=""}]] -> w956
                  tunnel: w957 -> [w962 _]
                  frame False {
                  }
                  frame True {
                  }
                }
                n548 = Sort 1D Array(array=w956) -> (sorted array=w958:T13)
                n549 = for {
                  tunnel: w958 -> [w965] mode=indexing
                  tunnel: [w964] -> w961 mode=indexing
                  n550 = Cluster To Array(cluster=w965) -> (array=w964:string[])
                }
              }
              frame #5 {
                # "THREAT"
                n551 = local read "threatDetails"() -> (w1006:T2)
                n552 = Unbundle By Name(w1006) -> ("barrelLength"=w1005:string)
                n553 = local read "Shot Angle"() -> (w1007:u16)
                n554 = control-ref of="weapon"() -> (w1018:refnum<vi>)
                n555 = control-ref of="projectileType"() -> (w1017:refnum<vi>)
                n556 = control-ref of="projectileWt"() -> (w1003:refnum<vi>)
                n557 = control-ref of="Powder Type"() -> (w1016:refnum<vi>)
                n558 = control-ref of="rangeNum"() -> (w1019:refnum<vi>)
                n559 = control-ref of="shooter"() -> (w1021:refnum<vi>)
                n560 = control-ref of="recorder"() -> (w1020:refnum<vi>)
                n561 = Format Into String(w1007) -> (resulting string=w1008:string)  [unwired: 3 in, 1 out]
                n562 = call "Dropdown Selection (SubVI).vi"("reference"=w1018) -> ("element"=w1014:string)
                n563 = call "Dropdown Selection (SubVI).vi"("reference"=w1017) -> ("element"=w1013:string)
                n564 = call "Dropdown Selection (SubVI).vi"("reference"=w1003) -> ("element"=w1004:string)
                n565 = call "Dropdown Selection (SubVI).vi"("reference"=w1016) -> ("element"=w1012:string)
                n566 = call "Dropdown Selection (SubVI).vi"("reference"=w1019) -> ("element"=w1011:string)
                n567 = call "Dropdown Selection (SubVI).vi"("reference"=w1021) -> ("element"=w1010:string)
                n568 = call "Dropdown Selection (SubVI).vi"("reference"=w1020) -> ("element"=w1009:string)
                n569 = Bundle("element"=w1014, "element"=w1013, "element"=w1004, "element"=w1012, "barrelLength"=w1005, w1008, "element"=w1011, "element"=w1010, "element"=w1009) -> (w1015:T20)  [unwired: 1 in]
                n570 = Cluster To Array(cluster=w1015) -> (array=w1002:string[])
              }
              frame #6 {
                # "GENERAL"
                n571 = control-ref of="Method"() -> (w1028:refnum<vi>)
                n572 = control-ref of="standard"() -> (w1029:refnum<vi>)
                n573 = local read "Comments"() -> (w1023:string)
                n574 = local read "projName"() -> (w1026:string)
                n575 = local read "projNum"() -> (w1025:string)
                n576 = local read "Panel"() -> (w1030:i32)
                n577 = call "Dropdown Selection (SubVI).vi"("reference"=w1028) -> ("element"=w1027:string)
                n578 = call "Dropdown Selection (SubVI).vi"("reference"=w1029) -> ("element"=w1022:string)
                n579 = Increment(x=w1030) -> (x+1=w1024:i32)
              }
            }
          }
          frame True {
            # "method"
            # "general"
            # "remark"
            # "threat"
            # "shots"
            # "sample"
            # "results"
            # "range"
            # "fabric"
            # "query db with the entered record number and use result to populate the xlt"
            n580 = Not(x=w1079) -> (.not. x?=w1078:bool)
            n581 = local write "lookupRec"(w1078) -> ()
            n582 = Format Into String(format string="SELECT * FROM Experiment\nWHERE expt=%d;" ("query string"), "Record #") -> (resulting string=w1075:string)  [unwired: 2 in, 1 out]
            n583 = call "Fetch Data (SubVI).vi"("connectString"=w1059, "query string"=w1075) -> ("recordset data"=w1077:string[][])  [unwired: 1 in, 1 out]
            n584 = Index Array(array=w1077) -> (element=w1035:string[])  [unwired: 2 in]
            n585 = Index Array(array=w1035, index=4) -> (element=w1032:string)
            n586 = local read "Impact/Separation"() -> (w1049:sgl)
            n587 = call "Load Shots (SubVI).vi"("connectString"=w1059, "Record #"="Record #", "Method"=w1032) -> ("Shot Array"=w1060:string[][], "avgDef"=w1038:dbl)
            n588 = local read "mid_to_targ_dist"() -> (w1052:sgl)
            n589 = local read "Barrel to Screen"() -> (w1055:sgl)
            n590 = Format Into String(w1038) -> (resulting string=w1036:string)  [unwired: 3 in, 1 out]
            n591 = Match Pattern(string=w1032, regular expression="N.I.J.") -> (offset past match=w1034:i32)  [unwired: 1 in, 3 out]
            n592 = Greater Or Equal To 0?(x=w1034) -> (x >= 0?=w1031:bool)
            n593 = Divide(x=w1049, y=sgl 2.0) -> (x/y=w1054:sgl)
            n594 = case shown="True" w1031 {
              tunnel: [w1082 w1086] -> w1037
              tunnel: w1036 -> [w1081 w1088]
              tunnel: w1035 -> [w1080 _]
              frame False {
                n595 = Array Subset(array=w1080, index=141, length=5) -> (w1083:string[])
                n596 = Build Array (concatenate)(w1083, w1081, w1081) -> (w1082:string[])
              }
              frame True {
                w1087 = ""
                n597 = Build Array(w1087, w1087, w1087, w1087, w1087, w1088, w1088) -> (w1086:string[])
              }
            }
            n598 = Add(x=w1055, y=w1052) -> (x+y=w1048:sgl)
            n599 = Subtract(x=w1055, y=w1054) -> (x-y=w1053:sgl)
            n600 = Subtract(x=w1052, y=w1054) -> (x-y=w1051:sgl)
            n601 = Array Subset(array=w1035, index=33, length=5) -> (w1041:string[])
            n602 = Format Into String(w1048) -> (resulting string=w1047:string)  [unwired: 3 in, 1 out]
            n603 = Format Into String(w1053) -> (resulting string=w1046:string)  [unwired: 3 in, 1 out]
            n604 = Format Into String(w1049) -> (resulting string=w1045:string)  [unwired: 3 in, 1 out]
            n605 = Format Into String(w1051) -> (resulting string=w1044:string)  [unwired: 3 in, 1 out]
            n606 = Format Into String(w1052) -> (resulting string=w1043:string)  [unwired: 3 in, 1 out]
            n607 = Array Subset(array=w1035, index=9, length=10) -> (w1067:string[])
            n608 = Build Array (concatenate)(w1047, w1046, w1045, w1044, w1043, w1041) -> (w1042:string[])
            n609 = Array Subset(array=w1035, index=19, length=9) -> (w1064:string[])
            n610 = Index Array(array=w1035, index #1=4 ("index")) -> (element #1=w1070:string, element #2=w1072:string, element #3=w1074:string, element #4=w1073:string)  [unwired: 3 in]
            n611 = Index Array(array=w1035, index=146) -> (element=w1061:string)
            n612 = Build Array(w1037) -> (w1062:string[][])
            n613 = call "Get Model Construction.vi"("panel record"=w1035) -> ("Fabric Array"=w1058:string[][])
          }
        }
        n614 = To Variant(anything=w792) -> (Variant=w786:variant)
        n615 = To Variant(anything=w791) -> (Variant=w785:variant)
        n616 = To Variant(anything=w790) -> (Variant=w784:variant)
        n617 = To Variant(anything=w789) -> (Variant=w783:variant)
        n618 = To Variant(anything=w788) -> (Variant=w782:variant)
        n619 = To Variant(anything=w787) -> (Variant=w781:variant)
        n620 = To Variant(anything=w769) -> (Variant=w780:variant)
        n621 = To Variant(anything=w768) -> (Variant=w779:variant)
        n622 = To Variant(anything=w767) -> (Variant=w778:variant)
        n623 = To Variant(anything=w766) -> (Variant=w775:variant)
        n624 = To Variant(anything=w765) -> (Variant=w776:variant)
        n625 = To Variant(anything=w764) -> (Variant=w777:variant)
        n626 = call "V50_OfficeReport.vi"("Enable"=w794, "blockFabric"=w786, "blockRange"=w785, "blockResults"=w784, "blockSample"=w783, "blockShotTbl"=w782, "blockThreat"=w781, "method"=w780, "projName"=w779, "projNum"=w778, "recNum"=w775, "remark"=w776, "standard"=w777) -> ("error out"=w793:errorcluster)  [unwired: 14 in]
        n627 = disable-structure shown="Disabled" {
          frame Disabled {
            n628 = call <vilib>:"Excel Set Cell Format.vi"() -> ()  [unwired: 14 in, 2 out]
            n629 = call <vilib>:"Excel Set Cell Dimension.vi"() -> ()  [unwired: 14 in, 2 out]
          }
          frame Enabled {
          }
        }
        n630 = call <vilib>:"Simple Error Handler.vi"("error in (no error)"=w793) -> ("error out"=w795:errorcluster)  [unwired: 4 in, 4 out]
        n631 = case shown="No Error" w795 {
          frame No Error {
            n632 = One Button Dialog(message="A Ballistic Test  Report is ready.") -> ()  [unwired: 1 in, 1 out]
          }
          frame Error {
          }
        }
      }
      frame 3 {
        # "SAVE SHOTS"
        # "This section saves the shots to the data base"
        n633 = stacked-sequence {
          seq-local: [w1110 _ _] -> [_ w1289 _]
          seq-local: [w1109 _ _] -> [_ w1283 _]
          seq-local: [_ w1269 _] -> [_ _ w1307]
          seq-local: [_ w1271 _] -> [_ _ w1306]
          seq-local: [_ w1267 _] -> [_ _ w1299]
          seq-local: [w1119 _ _] -> [_ w1266 _]
          seq-local: [w1118 _ _] -> [_ w1265 _]
          tunnel: [_ _ w1301] -> w1098
          tunnel: [_ _ w1304] -> w1100
          tunnel: w1096 -> [w1105 _ _]
          tunnel: w1095 -> [w1108 _ _]
          tunnel: w1094 -> [w1107 _ _]
          tunnel: w1093 -> [w1106 _ _]
          tunnel: w1091 -> [_ w1194 w1298]
          tunnel: w1090 -> [w1103 _ _]
          frame #0 {
            n634 = local read "fab1_totalWt"() -> (w1117:sgl)
            n635 = local read "fab2_totalWt"() -> (w1116:sgl)
            n636 = local read "fab3_totalWt"() -> (w1115:sgl)
            n637 = local read "fab4_totalWt"() -> (w1114:sgl)
            n638 = local read "fab5_totalWt"() -> (w1113:sgl)
            n639 = local read "fab6_totalWt"() -> (w1112:sgl)
            n640 = call "Get Number of Layers (SubVI).vi"("Layers Array"=w1105) -> ("numLayers"=w1104:i32)
            n641 = Format Into String(format string=" VALUES (%d ", w1104) -> (resulting string=w1122:string)  [unwired: 2 in, 1 out]
            n642 = Build Array(w1117, w1116, w1115, w1114, w1113, w1112) -> (w1111:sgl[])
            n643 = for {
              shift-right: [w1132] -> w1109
              shift-left: w1122 -> [w1133]
              shift-right: [w1129] -> w1110
              shift-left: "insert into experiment (plytypes " ("SQL statement") -> [w1130]
              tunnel: w1111 -> [w1123] mode=indexing
              tunnel: w1108 -> [w1128] mode=indexing
              tunnel: w1107 -> [w1127] mode=indexing
              tunnel: w1105 -> [w1125] mode=indexing
              tunnel: w1106 -> [w1126] mode=indexing
              i -> [w1131]
              n644 = Less Or Equal To 0?(x=w1123) -> (x <= 0?=w1124:bool)
              n645 = case shown="False" w1124 {
                tunnel: w1133 -> [w1169 w1172]
                tunnel: [w1168 w1172] -> w1132
                tunnel: w1131 -> [w1167 _]
                tunnel: w1130 -> [w1165 w1171]
                tunnel: [w1164 w1171] -> w1129
                tunnel: w1123 -> [w1158 _]
                tunnel: w1125 -> [w1157 _]
                tunnel: w1128 -> [w1153 _]
                tunnel: w1127 -> [w1152 _]
                tunnel: w1126 -> [w1150 _]
                frame False {
                  # "fabric style"
                  n646 = Unbundle By Name(w1157) -> ("plyNum"=w1143:i32, "LotNum"=w1154:string, "RollNum"=w1155:string, "Fabric.stitch"=w1156:u16)
                  n647 = Unbundle By Name(w1153) -> ("Fabric.fiber"=w1148:string, "Fabric.denier"=w1146:string, "pick"=w1142:string, "weave"=w1147:string, "fabricID_DHB"=w1140:string, "finish"=w1139:string, "SAK_fabric"=w1136:string, "ozPerYd2"=w1138:string)
                  n648 = property on="Fabric.stitch" class="Ring (strict)"() -> ("Strings []"=w1141:string[])  [unwired: 2 in, 2 out]
                  n649 = To Long Integer(number=w1156) -> (32bit integer=w1160:i32)
                  n650 = call <vilib>:"Space Constant.vi"() -> ("String"=w1161:string)
                  n651 = Increment(x=w1167) -> (x+1=w1137:i32)
                  n652 = Index Array(array=w1141, index=w1160) -> (element=w1159:string)
                  n653 = Concatenate Strings(w1154, w1161) -> (w1163:string)
                  n654 = Concatenate Strings(w1155, w1161) -> (w1162:string)
                  n655 = call "Dropdown Selection (SubVI).vi"("reference"=w1150) -> ("element"=w1149:string)
                  n656 = call "Dropdown Selection (SubVI).vi"("reference"=w1152) -> ("element"=w1151:string)
                  n657 = Format Into String(format string=", ply%1dnumber, fab%1d_vendor_PB, fab%1d_styleNum_PB, fab%1d_fiberType_PB, fab%1d_denier_PB, fab%1d_pick_PB, fab%1d_weave_PB, fab%1d_lotNum_PB, fab%1d_rollNum_PB, fab%1d_ozPerYd2_PB,fab%1d_stitch_PB, fab%1d_totalWeight_PB, fab%1d_fabricID_DHB, fab%1d_finishType_PB, FK_styleFabric%1d", initial string=w1165, w1137, w1137, w1137, w1137, w1137, w1137, w1137, w1137, w1137, w1137, w1137, w1137, w1137, w1137, w1137) -> (resulting string=w1164:string)  [unwired: 1 in, 1 out]
                  n658 = Scan From String(input string=w1138, default 1=sgl 0.0 ("default value 1")) -> (output 1=w1145:sgl)  [unwired: 3 in, 3 out]
                  n659 = Scan From String(input string=w1136, default 1=0) -> (output 1=w1135:i32)  [unwired: 3 in, 3 out]
                  n660 = Format Into String(format string=", %d,  '%s',  '%s',  '%s',  '%s',  '%s',  '%s',  '%s',  '%s', %.1f,  '%s', %.2f ,  '%s',  '%s', %d", initial string=w1169, w1143, w1149, w1151, w1148, w1146, w1142, w1147, w1163, w1162, w1145, w1159, w1158, w1140, w1139, w1135) -> (resulting string=w1168:string)  [unwired: 1 in, 1 out]
                }
                frame True {
                }
              }
            }
            n661 = call-poly <vilib>:"DB Tools Open Connection.vi"("connection information"=w1103) -> ("error out"=w1118:errorcluster, "connection reference"=w1119:T21)  [unwired: 7 in]
          }
          frame #1 {
            w1281 = " " ("Substring")
            # "DP/PB shared requirements:"
            # "Added PBBA requirements:"
            n662 = Array Size(array=w1194) -> (size(s)=w1263:i32)
            n663 = local read "Panel"() -> (w1268:i32)
            n664 = local read "Drag Corrected"() -> (w1274:bool)
            n665 = local read "computed_V50"() -> (w1279:sgl)
            n666 = local read "Impact factor"() -> (w1276:sgl)
            n667 = local read "Shot Angle"() -> (w1290:u16)
            n668 = Increment(x=w1268) -> (x+1=w1267:i32)
            n669 = control-ref of="ballistician"() -> (w1219:refnum<vi>)
            n670 = control-ref of="Submitter"() -> (w1218:refnum<vi>)
            n671 = control-ref of="Test Conditions"() -> (w1217:refnum<vi>)
            n672 = control-ref of="Type"() -> (w1224:refnum<vi>)
            n673 = control-ref of="Panel Stitch"() -> (w1225:refnum<vi>)
            n674 = control-ref of="Panel Type"() -> (w1226:refnum<vi>)
            n675 = control-ref of="projectileType"() -> (w1208:refnum<vi>)
            n676 = control-ref of="projectileWt"() -> (w1209:refnum<vi>)
            n677 = call "Dropdown Selection (SubVI).vi"("reference"=w1219) -> ("element"=w1216:string)
            n678 = call "Dropdown Selection (SubVI).vi"("reference"=w1218) -> ("element"=w1215:string)
            n679 = call "Dropdown Selection (SubVI).vi"("reference"=w1217) -> ("element"=w1214:string)
            n680 = call "Dropdown Selection (SubVI).vi"("reference"=w1224) -> ("element"=w1223:string)
            n681 = call "Dropdown Selection (SubVI).vi"("reference"=w1225) -> ("element"=w1222:string)
            n682 = call "Dropdown Selection (SubVI).vi"("reference"=w1226) -> ("element"=w1221:string)
            n683 = call "Dropdown Selection (SubVI).vi"("reference"=w1208) -> ("element"=w1189:string)
            n684 = call "Dropdown Selection (SubVI).vi"("reference"=w1209) -> ("element"=w1190:string)
            n685 = local read "totalNumPlies"() -> (w1262:i32)
            n686 = local read "Z.M.R."() -> (w1201:sgl)
            n687 = Select(t=w1276, s=w1274, f=sgl 1.0) -> (s? t:f=w1275:sgl)
            n688 = Equal?(x=w1190, y="Select . . .") -> (x = y?=w1192:bool)
            n689 = Less Than 0?(x=w1201) -> (x < 0?=w1200:bool)
            n690 = Divide(x=w1279, y=w1275) -> (x/y=w1278:sgl)
            n691 = control-ref of="Mfr"() -> (w1237:refnum<vi>)
            n692 = control-ref of="Powder Type"() -> (w1235:refnum<vi>)
            n693 = control-ref of="PanelBack"() -> (w1234:refnum<vi>)
            n694 = control-ref of="N.I.J"() -> (w1232:refnum<vi>)
            n695 = control-ref of="Method"() -> (w1180:refnum<vi>)
            n696 = control-ref of="Panel Dimensions"() -> (w1229:refnum<vi>)
            n697 = Concatenate Strings(w1223, w1281, w1222, w1281, w1221, w1281, "Fabric Description") -> (w1256:string)
            n698 = case shown="True" w1192 {
              tunnel: [w1291 "0" ("element")] -> w1191
              tunnel: w1190 -> [w1291 _]
              frame False {
              }
              frame True {
              }
            }
            n699 = case shown="True" w1200 {
              tunnel: w1201 -> [w1296 _]
              tunnel: [w1296 sgl 0.0 ("Z.M.R.")] -> w1199
              frame False {
              }
              frame True {
              }
            }
            n700 = control-ref of="Method"() -> (w1230:refnum<vi>)
            n701 = control-ref of="workType"() -> (w1184:refnum<vi>)
            n702 = call "Dropdown Selection (SubVI).vi"("reference"=w1237) -> ("element"=w1236:string)
            n703 = call "Dropdown Selection (SubVI).vi"("reference"=w1235) -> ("element"=w1188:string)
            n704 = call "Dropdown Selection (SubVI).vi"("reference"=w1234) -> ("element"=w1233:string)
            n705 = call "Dropdown Selection (SubVI).vi"("reference"=w1232) -> ("element"=w1231:string)
            n706 = call "Dropdown Selection (SubVI).vi"("reference"=w1180) -> ("element"=w1178:string)
            n707 = call "Dropdown Selection (SubVI).vi"("reference"=w1229) -> ("element"=w1228:string)
            n708 = call "Dropdown Selection (SubVI).vi"("reference"=w1230) -> ("element"=w1179:string)
            n709 = call "Dropdown Selection (SubVI).vi"("reference"=w1184) -> ("element"=w1176:string)
            n710 = Equal?(x=w1179, y="V50") -> (x = y?=w1175:bool)
            n711 = Equal?(x=w1176, y="QC") -> (x = y?=w1174:bool)
            n712 = And(x=w1175, y=w1174) -> (x .and. y?=w1173:bool)
            n713 = case shown="True" w1173 {
              tunnel: ["n/a" w1295] -> w1181
              frame False {
              }
              frame True {
                n714 = Format Into String("minV50") -> (resulting string=w1295:string)  [unwired: 3 in, 1 out]
              }
            }
            n715 = control-ref of="Panel Technician"() -> (w1227:refnum<vi>)
            n716 = local read "rangeOfResults"() -> (w1186:i32)
            n717 = call "Dropdown Selection (SubVI).vi"("reference"=w1227) -> ("element"=w1182:string)
            n718 = local read "threatDetails"() -> (w1206:T2)
            n719 = control-ref of="standard"() -> (w1255:refnum<vi>)
            n720 = control-ref of="workType"() -> (w1198:refnum<vi>)
            n721 = control-ref of="Model"() -> (w1196:refnum<vi>)
            n722 = local read "lowComplete"() -> (w1187:i32)
            n723 = call "Dropdown Selection (SubVI).vi"("reference"=w1255) -> ("element"=w1254:string)
            n724 = call "Dropdown Selection (SubVI).vi"("reference"=w1198) -> ("element"=w1251:string)
            n725 = call "Dropdown Selection (SubVI).vi"("reference"=w1196) -> ("element"=w1197:string)
            n726 = local read "totalBAW"() -> (w1220:sgl)
            n727 = control-ref of="covering"() -> (w1248:refnum<vi>)
            n728 = control-ref of="shooter"() -> (w1246:refnum<vi>)
            n729 = control-ref of="recorder"() -> (w1244:refnum<vi>)
            n730 = control-ref of="rangeNum"() -> (w1212:refnum<vi>)
            n731 = control-ref of="weapon"() -> (w1241:refnum<vi>)
            n732 = control-ref of="projectileType"() -> (w1238:refnum<vi>)
            n733 = local read "clayAverage"() -> (w1203:sgl)
            n734 = Unbundle By Name(w1206) -> ("barrelLength"=w1207:string, "FK_threat"=w1202:string)
            n735 = local read "highPartial"() -> (w1213:i32)
            n736 = call "Dropdown Selection (SubVI).vi"("reference"=w1248) -> ("element"=w1247:string)
            n737 = call "Dropdown Selection (SubVI).vi"("reference"=w1246) -> ("element"=w1245:string)
            n738 = call "Dropdown Selection (SubVI).vi"("reference"=w1244) -> ("element"=w1243:string)
            n739 = call "Dropdown Selection (SubVI).vi"("reference"=w1212) -> ("element"=w1211:string)
            n740 = call "Dropdown Selection (SubVI).vi"("reference"=w1241) -> ("element"=w1240:string)
            n741 = call "Dropdown Selection (SubVI).vi"("reference"=w1238) -> ("element"=w1239:string)
            n742 = Scan From String(input string=w1202, default 1=0) -> (output 1=w1204:i32)  [unwired: 3 in, 3 out]
            n743 = Format Into String(format string=", %d, #%s#, '%s', '%s', %d, '%s', '%s', %.4f, '%s', '%s', '%s', %.4f, %.1f, %.6f, '%s', %.4f, '%s', %d, '%s', %d, '%s', '%s', %d, '%s', %.1f, %.1f, %.2f, '%s', %.1f, '%s', '%s', '%s', '%s', '%s', '%s', '%s', '%s', %.1f, %.1f, '%s', '%s', '%s', '%s', '%s', '%s', '%s', '%s', %.1f, '%s', %.1f, %d, %d, %d, %d)" ("Format String"), initial string=w1283, w1267, "currentDateTime", w1216, w1215, w1290, w1214, w1256, "Areal Density", "Areal density text", w1189, w1191, "Weight of Panel", w1279, w1278, w1236, "Thickness", w1188, w1263, w1233, w1262, "Comments", w1231, "B.F.S (mm)", w1178, "RoomT", "RoomHum", "Version", w1228, w1199, "Sample #", w1182, w1254, "projName", "projNum", w1251, "serialNum", w1197, "totalSampleWt", w1220, w1247, w1181, w1245, w1243, w1211, w1240, w1239, w1207, "clayTemp", "clayCalib", w1203, w1213, w1187, w1186, w1204) -> (resulting string=w1282:string)  [unwired: 1 in, 1 out]
            n744 = Concatenate Strings(w1289, ", expt, [date], operator, submitter, angle, conditions, fabric, density, densitytext, threat,weight, panelweight, v50dc, v50 , maker, thickness, powder, numshots, backing, totalnumberplys, testcomments, nij, bfs, method, temperature, humidity, version, dimensions, zmr, sampleid, panelmaker,\nstandard_PB, projName_PB, projNum_PB, workType_PB, serialNum_PB, model_PB, totalSampleWt_PB,totalBAW_PB,covering_PB, minV50_PB,  shooter_PB, recorder_PB, rangeNum_PB, weapon_PB, projectile_PB, barrelLen_PB, clayTemp_PB, clayCal_PB, clayAvg_PB, highPartial_PB, lowComplete_PB, rangeOfResults_PB,FK_Projectile)" ("Substring"), w1282) -> (w1273:string)
            n745 = call-poly <vilib>:"DB Tools Execute Query.vi"("error in (no error)"=w1265, "SQL query"=w1273, "connection reference"=w1266) -> ("error out"=w1272:errorcluster, "recordset reference"=w1270:T22)  [unwired: 5 in]
            n746 = call-poly <vilib>:"DB Tools Free Object.vi"("error in (no error)"=w1272, "recordset reference"=w1270) -> ("error out"=w1271:errorcluster, "connection reference"=w1269:T21)  [unwired: 8 in]
          }
          frame #2 {
            # "Experiment.expt"
            n747 = local read "Shot"() -> (w1305:i32)
            n748 = Increment(x=w1305) -> (x+1=w1303:i32)
            n749 = for {
              tunnel: w1298 -> [w1351] mode=indexing
              tunnel: w1307 -> [w1323]
              tunnel: w1306 -> [w1325]
              tunnel: [w1321] -> w1300
              tunnel: [w1322] -> w1302
              tunnel: w1303 -> [w1329]
              tunnel: [w1320] -> w1304
              tunnel: w1299 -> [w1316]
              i -> [w1320]
              # "Shot.id"
              n750 = Add(x=w1329, y=w1320) -> (x+y=w1328:i32)
              n751 = local read "Drag Corrected"() -> (w1309:bool)
              n752 = local read "Residual factor"() -> (w1334:sgl)
              n753 = local read "Impact factor"() -> (w1308:sgl)
              n754 = Unbundle By Name(w1351) -> ("IMPACT VELOCITY"=w1337:sgl, "Redundant_Velocity"=w1312:sgl, "RESIDUAL  VELOCITY"=w1311:sgl, "Shot Description"=w1313:string, "Powder Loading"=w1341:sgl, "Barrel Temperature"=w1342:sgl, "TIME / DATE"=w1343:string, "shot order"=w1344:i32, "Shot Angle"=w1345:u16, "BackFace\nDepth"=w1346:sgl, "BackFace\nDiameter"=w1347:sgl, "SHOT STATUS"=w1349:u16, "Projectile Mass"=w1340:sgl, "usedv50"=w1339:bool, "Energy Loss (J)"=w1338:sgl, "avgVel_PB"=w1319:sgl, "velLoss_PB"=w1318:sgl, "strikeVel_PB"=w1317:sgl)
              n755 = Select(t=w1308, s=w1309, f=sgl 1.0) -> (s? t:f=w1332:sgl)
              n756 = Select(t=w1308, s=w1309, f=sgl 1.0) -> (s? t:f=w1314:sgl)
              n757 = Select(t=w1334, s=w1309, f=sgl 1.0) -> (s? t:f=w1333:sgl)
              n758 = Greater Than 0?(x=w1349) -> (x > 0?=w1348:bool)
              n759 = Divide(x=w1337, y=w1332) -> (x/y=w1330:sgl)
              n760 = Divide(x=w1312, y=w1314) -> (x/y=w1310:sgl)
              n761 = Divide(x=w1311, y=w1333) -> (x/y=w1336:sgl)
              n762 = Format Into String(format string="INSERT INTO shots (impactdc, redundantdc, residualdc,  comment, loading, barreltemp, [date], [order], shotangle, bfdepth, bfdiameter, [complete], expt, id, weight,usedv50, loss, residual, impact, redundant, avgVel_PB, velLoss_PB, strikeVel_PB)  VALUES (%.1f, %.1f, %.1f, '%s', %.4f, %.1f, #%s#, %d, %d, %.3f, %.3f, %d, %d, %d, %.4f, %d, %.4f, %.1f, %.1f, %.1f, %.1f, %.1f, %.1f)" ("Substring"), w1337, w1312, w1311, w1313, w1341, w1342, w1343, w1344, w1345, w1346, w1347, w1348, w1316, w1328, w1340, w1339, w1338, w1336, w1330, w1310, w1319, w1318, w1317) -> (resulting string=w1324:string)  [unwired: 2 in, 1 out]
              n763 = call-poly <vilib>:"DB Tools Execute Query.vi"("error in (no error)"=w1325, "SQL query"=w1324, "connection reference"=w1323) -> ("error out"=w1327:errorcluster, "recordset reference"=w1326:T22)  [unwired: 5 in]
              n764 = call-poly <vilib>:"DB Tools Free Object.vi"("error in (no error)"=w1327, "recordset reference"=w1326) -> ("error out"=w1321:errorcluster, "connection reference"=w1322:T21)  [unwired: 8 in]
            }
            n765 = call <vilib>:"DB Tools Close Connection.vi"("error in (no error)"=w1300, "connection reference"=w1302) -> ("error out"=w1301:errorcluster)  [unwired: 5 in]
          }
        }
        n766 = case shown="Error" w1098 {
          selector: w1098 -> [w1356 w1373]
          tunnel: [w1355 w1375] -> w1101
          tunnel: [w1355 w1375] -> w1102
          tunnel: w1100 -> [w1368 _]
          tunnel: w1092 -> [w1357 _]
          frame No Error {
            w1358 = "Data Base Parameters" ("section")
            w1355 = 5
            n767 = local read "Shot"() -> (w1369:i32)
            n768 = Increment(x=w1369) -> (x+1=w1363:i32)
            n769 = call <vilib>:"Open Config Data (compatibility).vi"("error in (no error)"=w1356, "configuration file path"=w1357) -> ("error out"=w1362:errorcluster, "refnum"=w1361:T23)  [unwired: 7 in, 1 out]
            n770 = Add(x=w1363, y=w1368) -> (x+y=w1364:i32)
            n771 = flat-sequence {
              tunnel: w1354 -> [_]
              frame #0 {
                w1370 = u8 2 ("Disabled")
                n772 = One Button Dialog(message="Data Saved") -> ()  [unwired: 1 in, 1 out]
                n773 = property on="Clear" class="Bool"("Disabled"=u8 0) -> ()  [unwired: 2 in, 2 out]
                n774 = property on="Accept Data" class="Bool (strict)"("Disabled"=w1370) -> ()  [unwired: 2 in, 2 out]
                n775 = property on="Reject shot" class="Bool"("Disabled"=w1370) -> ()  [unwired: 2 in, 2 out]
                n776 = property on="Save" class="Bool"("Disabled"=w1370) -> ()  [unwired: 2 in, 2 out]
              }
            }
            n777 = local write "Shot"(w1364) -> ()
            n778 = local read "Panel"() -> (w1365:i32)
            n779 = call-poly <vilib>:"Write Key.vi"("section"=w1358, "error in (no error)"=w1362, "value"=w1364, "key"="Last Shot Saved ", "refnum"=w1361) -> ("error out"=w1360:errorcluster, "refnum out"=w1359:T23)  [unwired: 4 in, 1 out]
            n780 = Increment(x=w1365) -> (x+1=w1352:i32)
            n781 = local write "Panel"(w1352) -> ()
            n782 = call-poly <vilib>:"Write Key.vi"("section"=w1358, "error in (no error)"=w1360, "value"=w1352, "key"="Last Panel Saved ", "refnum"=w1359) -> ()  [unwired: 4 in, 3 out]
            n783 = To Double Precision Float(number=w1352) -> (double precision float=w1353:dbl)
            n784 = call <vilib>:"Close Config Data.vi"("error in (no error)"=w1360, "refnum"=w1359) -> ("error out"=w1354:errorcluster)  [unwired: 8 in, 1 out]
            n785 = property on="Record #" class="DigNum (strict)"("Maximum"=w1353) -> ()  [unwired: 2 in, 2 out]
          }
          frame Error {
            w1375 = -1
            n786 = call <vilib>:"Simple Error Handler.vi"("error in (no error)"=w1373) -> ()  [unwired: 4 in, 5 out]
            n787 = One Button Dialog(message="Error saving Data. ") -> ()  [unwired: 1 in, 1 out]
          }
        }
      }
      frame 4 {
        w1418 = -1 ("index of element")
        # "ACCEPT DATA"
        # "Shot Order"
        # "This section accepts new data to the shot table."
        n788 = local read "residual/speed"() -> (w1394:sgl)
        n789 = local read "Impact/speed"() -> (w1389:sgl)
        n790 = Not(x=w1381) -> (.not. x?=w1380:bool)
        n791 = property on="Reject shot" class="Bool"("Disabled"=u8 0) -> ()  [unwired: 2 in, 2 out]
        n792 = local read "Current/redundant/speed"() -> (w1387:sgl)
        n793 = local read "Current/residual/speed"() -> (w1408:sgl)
        n794 = local read "BACKFACE DIAMETER"() -> (w1413:sgl)
        n795 = local read "Current/impact/speed"() -> (w1386:sgl)
        n796 = local read "Corrected Redundant"() -> (w1384:sgl)
        n797 = Array Size(array=w1379) -> (size(s)=w1411:i32)
        n798 = local read "Current/avg/speed"() -> (w1382:sgl)
        n799 = local read "Corrected Residual"() -> (w1409:sgl)
        n800 = local read "BACKFACE DEPTH"() -> (w1405:sgl)
        n801 = local read "Redundant/speed"() -> (w1385:sgl)
        n802 = local read "Corrected Impact"() -> (w1407:sgl)
        n803 = local read "conversion factor"() -> (w1397:sgl)
        n804 = local read "SHOT STATUS"() -> (w1412:u16)
        n805 = local read "Avg/speed"() -> (w1383:sgl)
        n806 = Increment(x=w1411) -> (x+1=w1388:i32)
        n807 = local write "Accept Data"(FALSE) -> ()
        n808 = Multiply(x=w1389, y=w1397) -> (x*y=w1399:sgl)
        n809 = Multiply(x=w1397, y=w1394) -> (x*y=w1398:sgl)
        n810 = Multiply(x=w1399, y=w1399) -> (x*y=w1404:sgl)
        n811 = Multiply(x=w1398, y=w1398) -> (x*y=w1403:sgl)
        n812 = Subtract(x=w1404, y=w1403) -> (x-y=w1401:sgl)
        n813 = Format Date/Time String(time format string (%c)="%x   %H:%M:%S") -> (date/time string=w1393:string)  [unwired: 2 in]
        "SUBMIT DATE/TIME" <- w1393
        n814 = Compound Arithmetic op=MULTIPLY("Projectile Mass", w1401, sgl 0.0005 ("Input")) -> (w1396:sgl)
        n815 = Index Array(array=w1379) -> (element=w1414:T5)  [unwired: 1 in]
        n816 = Bundle By Name(cluster=w1414, "TIME / DATE"=w1393, "shot order"=w1388, "IMPACT VELOCITY"=w1389, "RESIDUAL  VELOCITY"=w1394, "Shot Description"="Shot Decription", "Powder Loading"="Powder Loading", "Barrel Temperature"="Barrel Temp", "SHOT STATUS"=w1412, "BackFace\nDepth"=w1405, "BackFace\nDiameter"=w1413, "Shot Angle"="Shot Angle", "Uncorrected Impact"=w1386, "Corrected Impact"=w1407, "Uncorrected Residual"=w1408, "Corrected residual"=w1409, "Projectile Mass"="Projectile Mass", "Energy Loss (J)"=w1396, "UncorrectedRed_PB"=w1387, "Redundant_Velocity"=w1385, "CorrectedRed_PB"=w1384, "UncorrectedAvgVel_PB"=w1382, "avgVel_PB"=w1383) -> (w1410:T5)
        n817 = Build Array (concatenate)(w1379, w1410) -> (w1378:T5[])
      }
      frame 5 {
        w1422 = u8 2 ("Disabled")
        w1424 = -1
        # "This section will clear the shot table and re-enable the \"ADD SHOT\" button to get ready for a new test panel."
        # "CLEAR SHOTS"
        n818 = invoke on="Table of Shots" class="Tbl (strict)" method="Reinit To Default"() -> ()  [unwired: 3 in, 3 out]
        n819 = invoke on="SHOTS" class="Arr (strict)" method="Reinit To Default"() -> ()  [unwired: 3 in, 3 out]
        n820 = property on="Accept Data" class="Bool (strict)"("Disabled"=u8 0) -> ()  [unwired: 2 in, 2 out]
        n821 = property on="Clear" class="Bool"("Disabled"=w1422) -> ()  [unwired: 2 in, 2 out]
        n822 = property on="Reject shot" class="Bool"("Disabled"=w1422) -> ()  [unwired: 2 in, 2 out]
        n823 = property on="Save" class="Bool"("Disabled"=w1422) -> ()  [unwired: 2 in, 2 out]
      }
      frame 6 {
        w1434 = -1
        # "REJECT LAST SHOT OR DELETE SHOT RECORD"
        # "This section unaccepts new data  OR deletes the currently accessed previous shot"
        n824 = local read "Delete Button"() -> (w1433:bool)
        n825 = case shown="True" w1433 {
          tunnel: w1432 -> [w1437 w1449]
          tunnel: [w1438 w1450] -> w1429
          frame False {
            n826 = Array Size(array=w1437) -> (size(s)=w1435:i32)
            n827 = local write "SUBMIT DATE/TIME"("" ("Empty String Constant")) -> ()
            n828 = while {
              tunnel: [w1441] -> w1436
              tunnel: w1435 -> [w1443]
              tunnel: w1437 -> [w1445] mode=indexing
              i -> [w1441]
              stop <- w1444 stop-if-true
              n829 = Unbundle By Name(w1445) -> ("shot order"=w1442:i32)
              n830 = Equal?(x=w1442, y=w1443) -> (x = y?=w1444:bool)
            }
            n831 = Delete From Array "Delete From Array"(array=w1437, index=w1436) -> (array with subset deleted=w1438:T5[])  [unwired: 1 in, 1 out]
            n832 = property on="Reject shot" class="Bool"("Disabled"=u8 2) -> ()  [unwired: 2 in, 2 out]
          }
          frame True {
            n833 = property on="SHOTS" class="Arr (strict)"() -> ("Index Values"=w1458:u32[])  [unwired: 2 in, 2 out]
            n834 = local write "Delete Button"(FALSE) -> ()
            n835 = Index Array(array=w1458, index=0 ("Index")) -> (element=w1448:u32)
            n836 = Index Array(array=w1449, index=w1448) -> (element=w1447:T5)
            n837 = Unbundle By Name(w1447) -> ("shot order"=w1446:i32)
            n838 = Format Into String(format string="The currently displayed Shot, #%d", w1446) -> (resulting string=w1455:string)  [unwired: 2 in, 1 out]
            n839 = Concatenate Strings(w1455, ", will be deleted.  IT CANNOT RECOVERED!  Do you want to DELETE the shot?" ("message")) -> (w1454:string)
            n840 = Two Button Dialog(message=w1454, 1:"NO I do NOT want to delete.  Cancel Request" ("F button name (\"Cancel\")"), 2:"YES I want to delete the shot" ("T button name (\"OK\")")) -> (T button?=w1461:bool)
            n841 = case shown="True" w1461 {
              tunnel: w1449 -> [w1474 w1477]
              tunnel: [w1474 w1479] -> w1452
              tunnel: w1448 -> [_ w1476]
              tunnel: [10000 ("shot order") w1478] -> w1451
              frame False {
              }
              frame True {
                n842 = Index Array(array=w1477, index=w1476) -> (element=w1475:T5)
                n843 = Unbundle By Name(w1475) -> ("shot order"=w1478:i32)
                n844 = Delete From Array(array=w1477, index=w1476) -> (array with subset deleted=w1479:T5[])  [unwired: 1 in, 1 out]
              }
            }
            n845 = for {
              tunnel: [w1468] -> w1450 mode=indexing
              tunnel: w1452 -> [w1463] mode=indexing
              tunnel: w1451 -> [w1467]
              n846 = Unbundle By Name(w1463) -> ("shot order"=w1465:i32)
              n847 = Decrement(x=w1465) -> (x-1=w1464:i32)
              n848 = Greater?(x=w1465, y=w1467) -> (0:w1466:bool)
              n849 = case shown="True" w1466 {
                tunnel: w1464 -> [_ w1471]
                tunnel: w1463 -> [w1469 w1472]
                tunnel: [w1469 w1470] -> w1468
                frame False {
                }
                frame True {
                  n850 = Bundle By Name(cluster=w1472, "shot order"=w1471) -> (w1470:T5)
                }
              }
            }
          }
        }
        n851 = property on="SHOTS" class="Arr (strict)"("Val(Sgnl)"=w1429) -> ()  [unwired: 2 in, 2 out]
      }
      frame 7 {
        w1491 = -1
        # "RESET RANGE"
        # "This section will reset range"
        n852 = Concatenate Strings("L|", "6|") -> (w1485:string)
        n853 = case shown="2" "Data Source" {
          tunnel: [w1492 w1495 w1498 w1533] -> w1487
          tunnel: w1486 -> [w1492 w1495 w1497 w1533]
          tunnel: w1485 -> [_ _ w1496 _]
          frame 0, Default {
            n854 = flat-sequence {
              frame #0 {
                n855 = local write "RANGE RESET"(FALSE ("RANGE RESET")) -> ()
              }
              frame #1 {
                n856 = Wait (ms)(milliseconds to wait=u32 100) -> ()  [unwired: 1 out]
              }
            }
          }
          frame 1 {
          }
          frame 2 {
            w1506 = u32 22 items=["NI-DAQ version", "device name", "base address", "data transfer mode for analog input", "data transfer mode for analog output group 1", "data transfer mode for analog output group 2", "data transfer mode for GPCTR 0", "data transfer mode for GPCTR 1", "data transfer mode for digital I/O group 1", "data transfer mode for digital I/O group 2", "device type code", "DMA A level", "DMA B level", "DMA C level", "interrupt A level", "interrupt B level", "reserved", "lpt device mode", "DAQCard-700 counter 1 source", "interrupt generation mode", "device state during suspend mode", "computer name", "serial number", "counter type", "Scarab A Memory Size", "Scarab B Memory Size"] ("information type")
            w1505 = u32 1  # device
            # "Screens"
            n857 = Concatenate Strings(w1496, "2|") -> (w1501:string)
            n858 = call <vilib>:"Get DAQ Device Information.vi"("information type"=w1506, "task ID or device"=w1505) -> ("error out"=w1500:errorcluster, "information string"=w1504:string)  [unwired: 7 in, 1 out]
            n859 = disable-structure "Diagram Disable Structure" shown="Disabled" {
              disable-tunnel: w1501 -> [w1512 _]
              disable-tunnel: w1500 -> [w1509 w1514]
              disable-tunnel: [w1508 w1514] -> w1499
              frame Disabled {
                n860 = Current VI's Path() -> (path=w1513:path)
                n861 = call "Where Am I (SubVI).vi"("TL Calling Location"=w1512, "Call VI path"=w1513) -> ("I'm here"=w1511:string)
                n862 = call "Error Check (SubVI).vi"("calling VI"=w1511, "tag #"=0, "error IN"=w1509) -> ("error OUT"=w1508:errorcluster)  [unwired: 2 in]
              }
              frame Enabled {
                # "Debug code is disabled"
              }
            }
            n863 = Unbundle By Name(w1500) -> ("status"=w1507:bool)
            n864 = case shown="True" w1507 {
              tunnel: w1504 -> [w1524 _]
              tunnel: [w1524 "DEVICE NOT READY!" ("information string")] -> w1503
              tunnel: w1499 -> [w1523 _]
              tunnel: [w1516 w1529] -> w1498
              tunnel: w1497 -> [_ w1529]
              frame False {
                # "assign task IDs to counters"
                n865 = local write "RANGE RESET"(FALSE ("RANGE RESET")) -> ()
                n866 = call "Config Counter to Measure Two Edge Separation.vi"("error IN"=w1523, "Counter"="Impact Timer", "device"="DAQ Card") -> ("error out"=w1526:errorcluster, "task ID out"=w1519:u32)  [unwired: 1 in]
                "impact/ID" <- w1519
                n867 = call "Config Counter to Measure Two Edge Separation.vi"("error IN"=w1526, "Counter"="Residual  Timer", "device"="DAQ Card") -> ("error out"=w1528:errorcluster, "task ID out"=w1517:u32)  [unwired: 1 in]
                "residual/ID" <- w1517
                n868 = call "Config Counter to Measure Two Edge Separation.vi"("error IN"=w1528, "Counter"="Redundant Timer", "device"="DAQ Card") -> ("error out"=w1527:errorcluster, "task ID out"=w1518:u32)  [unwired: 1 in]
                "Red/ID" <- w1518
                n869 = Bundle("task ID out"=w1519, "task ID out"=w1518, "task ID out"=w1517) -> (w1516:T24)  [unwired: 1 in]
                n870 = call <vilib>:"Simple Error Handler.vi"("error in (no error)"=w1527) -> ()  [unwired: 4 in, 5 out]
              }
              frame True {
                w1532 = u16 0 items=["Simulated", "Radar", "Screens"] ("Data Source")
                n871 = local write "Data Source"(w1532) -> ()
                n872 = One Button Dialog(message="Error initializing Timer board.  Switching to simulation") -> ()  [unwired: 1 in, 1 out]
              }
            }
            "Device S/N" <- w1503
          }
          frame 3 {
          }
        }
        n873 = local write "SUBMIT DATE/TIME"("" ("Empty String Constant")) -> ()
      }
    }
  }
  n874 = while {
    shift-right: [w1535] -> _
    shift-left: "" ("NewVal") -> [w1536]
    stop <- FALSE stop-if-true
    n875 = event shown="[0] Timeout" {
      selector: _ -> [_ _ _ _ _ _ _ _ _ _ _ _ _ _ _ _ _ _]
      dyn-events: _ -> [_ _ _ _ _ _ _ _ _ _ _ _ _ _ _ _ _ _]
      timeout: 200 -> [_ _ _ _ _ _ _ _ _ _ _ _ _ _ _ _ _ _]
      tunnel: w1536 -> [w1543 w1547 w1552 _ w1561 w1593 w1602 w1603 w1620 w1638 w1652 w1691 w1695 w1732 w1764 w1766 w1775 w1782]
      tunnel: [w1543 w1547 w1552 w1553 w1561 w1593 w1602 w1603 w1620 w1638 w1652 w1691 w1695 w1732 w1764 w1766 w1775 w1782] -> w1535
      event Timeout {
        n876 = event-data() -> ()  [unwired: 1 in, 1 out]
        n877 = Get Date/Time String(want seconds? (F)=TRUE) -> (date string=w1541:string, time string=w1540:string)  [unwired: 2 in]
        n878 = call <vilib>:"Space Constant.vi"() -> ("String"=w1542:string)
        n879 = Concatenate Strings(w1541, w1542, w1540) -> (→"timestamp":string)
      }
      event "EXIT": Value Change {
        # "The EXIT button is for normal user exit.\n\nFor tech support, a hidden STOP control can be accessed by Ctrl-Shft-F10.\n(enables view of error messages)"
        n880 = event-data() -> ()  [unwired: 1 in, 5 out]
        n881 = property class="App"() -> ("App.Kind"=w1546:T25)  [unwired: 2 in, 2 out]
        n882 = Two Button Dialog(message="All Unsaved data will be lost.   Do you want to quit the program? ") -> (T button?=w1545:bool)  [unwired: 2 in]
        n883 = case shown="\"Development System\"" w1546 {
          tunnel: w1545 -> [w1548 w1549 w1550]
          frame "invalid app kind", Default {
            n884 = Stop(stop? (T)=w1548) -> ()
          }
          frame "Run Time System" {
            n885 = Quit LabVIEW(quit? (T)=w1549) -> ()
          }
          frame "Development System" {
            n886 = Stop(stop? (T)=w1550) -> ()
          }
        }
      }
      event "STOP": Value Change {
        # "This is for tech support to enable view of error messages.\n\nWhile running, it can be accessed by Ctrl-Shft-F10 (even after being built).\n\nThe control is located just out of view on the FP to the righ of the EXIT button."
        n887 = event-data() -> ()  [unwired: 1 in, 5 out]
        n888 = Stop(stop? (T)=TRUE) -> ()
      }
      event "connStr": Value Change {
        n889 = event-data() -> ("NewVal"=w1553:string)  [unwired: 1 in, 5 out]
      }
      event "projectileType", "QueryLoad": Value Change {
        w1556 = "%x" ("time format string (%c)")
        w1577 = "" ("replace string (\"\")")
        # "This section plots  Impact velocity vs. loadingdata"
        n890 = event-data() -> ()  [unwired: 1 in, 6 out]
        n891 = control-ref of="Powder Type"() -> (w1564:refnum<vi>)
        n892 = control-ref of="projectileType"() -> (w1560:refnum<vi>)
        n893 = call "Dropdown Selection (SubVI).vi"("reference"=w1564) -> ("element"=w1562:string)
        n894 = call "Dropdown Selection (SubVI).vi"("reference"=w1560) -> ("element"=w1563:string)
        n895 = Format Date/Time String(time format string (%c)=w1556, seconds (now)="lkupStartDate") -> (date/time string=w1555:string)  [unwired: 1 in]
        n896 = Format Date/Time String(time format string (%c)=w1556, seconds (now)="lkupEndDate") -> (date/time string=w1554:string)  [unwired: 1 in]
        n897 = call "Trim String.vi"("inStr"=w1562) -> ("outStr"=w1575:string)
        n898 = call "Trim String.vi"("inStr"=w1563) -> ("outStr"=w1576:string)
        n899 = call "Get Projectile Atributes.vi"("connectString"=w1561, "projectile"=w1560) -> ("projectileAttribs"=→"threatDetails":T2)
        n900 = invoke on="v50_table" class="Tbl" method="Reinit To Default"() -> (error out=w1568:errorcluster)  [unwired: 3 in, 2 out]
        n901 = invoke on="Vel.vs.Loading" class="XYGraph (strict)" method="Reinit To Default"(error in=w1568) -> (error out=w1558:errorcluster)  [unwired: 2 in, 2 out]
        n902 = Format Into String(format string="  select top %d shots.loading, shots.avgVel_PB,  shots.date from shots, experiment where shots.expt = experiment.expt and shots.loading >= 0 and shots.date between  #%s# and #%s# and shots.impact between 5000 and 10 and experiment.powder like '%%%s%%' and experiment.threat like '%%%s%%' and experiment.threat<>'' order by shots.loading,shots.impact" ("Format String"), error in=w1558, "maxRecs", w1555, w1554, w1575, w1576) -> (resulting string=w1581:string, error out=w1566:errorcluster)  [unwired: 1 in]
        n903 = Search and Replace String(input string=w1581, search string=" and experiment.powder like '%%'", replace string=w1577, error in=w1566) -> (result string=w1579:string, error out=w1567:errorcluster)  [unwired: 4 in, 2 out]
        n904 = Search and Replace String(input string=w1579, search string="and experiment.threat like '%%'", replace string=w1577, error in=w1567) -> (result string=w1570:string, error out=w1565:errorcluster)  [unwired: 4 in, 2 out]
        n905 = call "Fetch Data (SubVI).vi"("error IN"=w1565, "connectString"=w1561, "query string"=w1570) -> ("recordset data"=w1571:string[][])  [unwired: 1 out]
        "v50_table" <- w1571
        n906 = Fract/Exp String To Number(string=w1571) -> (number=w1585:dbl[][])  [unwired: 3 in, 1 out]
        n907 = Array Size(array=w1571) -> (size(s)=w1573:i32[])
        n908 = Index Array(array=w1573) -> (element=→"ActualNumRecs":i32)  [unwired: 1 in]
        n909 = Index Array(array=w1585, index (col)=1 ("Disabled Index (col)")) -> (element=w1584:dbl[])  [unwired: 1 in]
        n910 = Index Array(array=w1585, index (col)=0 ("Disabled Index (col)")) -> (element=w1583:dbl[])  [unwired: 1 in]
        n911 = Bundle(w1583, w1584) -> (→"Vel.vs.Loading":cluster{dbl[], dbl[]})  [unwired: 1 in]
      }
      event "srchParams": Value Change {
        # "This section returns past panels"
        n912 = event-data() -> ()  [unwired: 1 in, 6 out]
        n913 = control-ref of="pastPanels"() -> (w1590:refnum<vi>)
        n914 = call "queryPanels (SubVI).vi"("connStr"=w1593, "srchParams"="srchParams", "pastPanels"=w1590) -> ("recordset data"=→"pastPanels":string[][], "actualNumPanels"=→"actualNumPanels":i32)  [unwired: 1 in, 1 out]
      }
      event "pastPanels": Mouse Up {
        n915 = event-data() -> ("CtlRef"=w1601:refnum<vi>)  [unwired: 1 in, 7 out]
        n916 = property class="Tbl (strict)"(reference=w1601) -> ("Value"=w1600:string[][], "EditPos"=w1599:T26)  [unwired: 1 in, 2 out]
        n917 = Unbundle By Name(w1599) -> ("Row"=w1598:i32)
        n918 = Index Array(array=w1600, index (row)=w1598, index (col)=0 ("disabled index (col)")) -> (element=w1597:string)
        n919 = Scan From String(input string=w1597, default 1=1 ("Record #")) -> (output 1=w1595:i32)  [unwired: 3 in, 3 out]
        n920 = local write "Record #"(w1595) -> ()
      }
      event "projectileWt": Value Change {
        n921 = event-data() -> ("CtlRef"=w1612:refnum<vi>)  [unwired: 1 in, 5 out]
        n922 = property on="Property Node" class="Ring (strict)"(reference=w1612) -> (reference out=w1607:refnum<vi>, "RingText.Text"=w1611:string)  [unwired: 1 in, 1 out]
        n923 = call "Select Projectile Type.vi"("connectString"=w1603, "projectileWeight"=w1611) -> ("projectileTypes"=w1610:string[])
        n924 = property on="projectileType" class="Ring (strict)"("Strings []"=w1610, "Val(Sgnl)"=u16 0 ("Value (Signaling)")) -> ()  [unwired: 2 in, 2 out]
        n925 = call "Dropdown Selection (SubVI).vi"("reference"=w1607) -> ("element"=w1606:string)
        n926 = Equal?(x=w1606, y="Select . . .") -> (x = y?=w1604:bool)
        n927 = case shown="False" w1604 {
          tunnel: [w1616 sgl 0.0] -> w1608
          tunnel: w1606 -> [w1613 _]
          frame False {
            w1618 = sgl 0.0  # sgl
            n928 = Scan From String(format string="%f " ("Format String"), input string=w1613, default 1=w1618) -> (output 1=w1617:sgl)  [unwired: 2 in, 3 out]
            n929 = Multiply(x=sgl 0.06479891, y=w1617) -> (x*y=w1616:sgl)
          }
          frame True {
          }
        }
        n930 = local write "Projectile Mass"(w1608) -> ()
      }
      event "fabVendor_1", "fabVendor_2", "fabVendor_3", "fabVendor_4", "fabVendor_5", "fabVendor_6", "srchParams.fabVendor_0": Value Change {
        n931 = event-data() -> ("CtlRef"=w1628:refnum<vi>)  [unwired: 1 in, 5 out]
        n932 = property on="Property Node" class="Ring (strict)"(reference=w1628) -> ("Label.Text"=w1624:string, "RingText.Text"=w1625:string)  [unwired: 1 in, 2 out]
        n933 = call "Select Fabric Style.vi"("connectString"=w1620, "Vendor"=w1625) -> ("fabStyles"=w1629:string[])
        n934 = Scan From String(format string="fabVendor_%d", input string=w1624, default 1=0 ("default value 1")) -> (output 1=w1623:i32)  [unwired: 2 in, 3 out]
        n935 = case shown="0" w1623 {
          tunnel: [refnum<vi> refnum ("fabStyle_6") w1631 w1632 w1633 w1634 w1635 w1636 w1637] -> w1622
          frame -1, Default {
          }
          frame 0 {
            n936 = control-ref of="fabStyle_0"() -> (w1631:refnum<vi>)
          }
          frame 1 {
            n937 = control-ref of="fabStyle_1"() -> (w1632:refnum<vi>)
          }
          frame 2 {
            n938 = control-ref of="fabStyle_2"() -> (w1633:refnum<vi>)
          }
          frame 3 {
            n939 = control-ref of="fabStyle_3"() -> (w1634:refnum<vi>)
          }
          frame 4 {
            n940 = control-ref of="fabStyle_4"() -> (w1635:refnum<vi>)
          }
          frame 5 {
            n941 = control-ref of="fabStyle_5"() -> (w1636:refnum<vi>)
          }
          frame 6 {
            n942 = control-ref of="fabStyle_6"() -> (w1637:refnum<vi>)
          }
        }
        n943 = property class="Ring (strict)"(reference=w1622, "Strings []"=w1629, "Val(Sgnl)"=u16 0 ("Value (Signaling)")) -> ()  [unwired: 1 in, 2 out]
      }
      event "fabStyle_1", "fabStyle_2", "fabStyle_3", "fabStyle_4", "fabStyle_5", "fabStyle_6", "srchParams.fabStyle_0": Value Change {
        n944 = event-data() -> ("CtlRef"=w1644:refnum<vi>)  [unwired: 1 in, 5 out]
        n945 = call "Get Fabic Style Atributes.vi"("connectString"=w1638, "Ring Refnum"=w1644) -> ("projectileAttribs"=w1639:T27)
        n946 = property class="Ring (strict)"(reference=w1644) -> ("Label.Text"=w1643:string)  [unwired: 1 in, 2 out]
        n947 = Scan From String(format string="fabStyle_%d", input string=w1643, default 1=0 ("default value 1")) -> (output 1=w1641:i32)  [unwired: 2 in, 3 out]
        n948 = case shown="0" w1641 {
          tunnel: w1639 -> [_ w1645 w1646 w1647 w1648 w1649 w1650 w1651]
          frame -1, Default {
          }
          frame 0 {
            n949 = property on="fabAttribs_0" class="Clust (strict)"("Val(Sgnl)"=w1645) -> ()  [unwired: 2 in, 2 out]
            "fabAttribs_0" <- w1645
          }
          frame 1 {
            n950 = property on="fabAttribs_1" class="Clust (strict)"("Val(Sgnl)"=w1646) -> ()  [unwired: 2 in, 2 out]
            "fabAttribs_1" <- w1646
          }
          frame 2 {
            n951 = property on="fabAttribs_2" class="Clust (strict)"("Val(Sgnl)"=w1647) -> ()  [unwired: 2 in, 2 out]
            "fabAttribs_2" <- w1647
          }
          frame 3 {
            n952 = property on="fabAttribs_3" class="Clust (strict)"("Val(Sgnl)"=w1648) -> ()  [unwired: 2 in, 2 out]
            "fabAttribs_3" <- w1648
          }
          frame 4 {
            n953 = property on="fabAttribs_4" class="Clust (strict)"("Val(Sgnl)"=w1649) -> ()  [unwired: 2 in, 2 out]
            "fabAttribs_4" <- w1649
          }
          frame 5 {
            n954 = property on="fabAttribs_5" class="Clust (strict)"("Val(Sgnl)"=w1650) -> ()  [unwired: 2 in, 2 out]
            "fabAttribs_5" <- w1650
          }
          frame 6 {
            n955 = property on="fabAttribs_6" class="Clust (strict)"("Val(Sgnl)"=w1651) -> ()  [unwired: 2 in, 2 out]
            "fabAttribs_6" <- w1651
          }
        }
      }
      event "Panel Search": Value Change {
        # "This section plots panel V50 data"
        n956 = event-data() -> ()  [unwired: 1 in, 6 out]
        n957 = invoke on="v50 data" class="Tbl" method="Reinit To Default"() -> (error out=w1666:errorcluster)  [unwired: 3 in, 2 out]
        n958 = invoke on="Previous V50 Data" class="WFGraph (strict)" method="Reinit To Default"(error in=w1666) -> (error out=w1665:errorcluster)  [unwired: 2 in, 2 out]
        n959 = control-ref of="queryThreat"() -> (w1657:refnum<vi>)
        n960 = call "Dropdown Selection (SubVI).vi"("reference"=w1657) -> ("element"=w1658:string)
        n961 = Format Into String(format string="SELECT  Experiment.Date, Shots.impact\nFROM Shots, Experiment where Shots.Expt = Experiment.expt\nand Experiment.Date Between #%s# And #%s# AND Experiment.threat Like '%%%s%%'\nORDER BY Experiment.Date" ("SQL statement"), error in=w1665, "beginCUSUM", "endCUSUM", w1658) -> (resulting string=w1656:string, error out=w1655:errorcluster)  [unwired: 1 in]
        n962 = call "Fetch Data (SubVI).vi"("error IN"=w1655, "connectString"=w1652, "query string"=w1656) -> ("error OUT"=w1654:errorcluster, "recordset data"=w1653:string[][])
        n963 = call "Get V50s (SubVI).vi"("recordset data"=w1653) -> ("V50 Array"=w1688:dbl[], "V50 Table"=→"v50 data":string[][], "lastVelocity"=w1670:dbl)
        "CUSUM_lastVel" <- w1670
        n964 = call <vilib>:"Std Deviation and Variance.vi"("X"=w1688, "Weighting (Sample)"=enum16{"Sample", "Population"}."Sample") -> ("mean"=w1686:dbl, "standard deviation"=w1687:dbl)  [unwired: 1 out]
        "Average Velocity" <- w1686
        "CUSUM_stdDev" <- w1687
        n965 = Array Size(array=w1688) -> (size(s)=w1677:i32)
        n966 = Subtract(x=w1686, y=w1670) -> (x-y=w1671:dbl)
        n967 = Absolute Value(x=w1671) -> (abs(x)=w1672:dbl)
        n968 = Multiply(x=3.0, y=w1687) -> (x*y=w1676:dbl)
        n969 = Divide(x=w1672, y=w1687) -> (x/y=w1683:dbl)
        n970 = Subtract(x=w1686, y=w1676) -> (x-y=w1679:dbl)
        n971 = Add(x=w1686, y=w1676) -> (x+y=w1678:dbl)
        n972 = Initialize Array(w1686, w1677) -> (w1659:dbl[])
        n973 = Initialize Array(w1679, w1677) -> (w1680:dbl[])
        n974 = Initialize Array(w1678, w1677) -> (w1681:dbl[])
        n975 = Format Into String(format string="%3.1f" ("Format String"), error in=w1654, w1683) -> (resulting string=w1682:string, error out=w1689:errorcluster)  [unwired: 1 in]
        n976 = Greater?(x=3.0, y=w1683) -> (0:→"In Control":bool)
        n977 = Build Array(w1688, w1659, w1680, w1681) -> (w1662:dbl[][])
        n978 = property on="In Control" class="Bool (strict)"(error in=w1689, "Boolean Text.Text"=w1682) -> (error out=w1690:errorcluster)  [unwired: 1 in, 1 out]
        n979 = Bundle(0.0, 1.0, w1662) -> (→"Previous V50 Data":cluster{dbl, dbl, dbl[][]})  [unwired: 1 in]
        n980 = call <vilib>:"Simple Error Handler.vi"("error in (no error)"=w1690) -> ()  [unwired: 4 in, 5 out]
      }
      event "SHOTS", "Sort by AVG": Value Change {
        n981 = event-data() -> ()  [unwired: 1 in, 6 out]
        n982 = local read "SHOTS"() -> (w1692:T5[])
        n983 = call "Update Shot Table.vi"("Sort by AVG"="Sort by AVG", "shot array"=w1692) -> ("shotTable OUT"=w1694:string[][])
        n984 = local write "Table of Shots"(w1694) -> ()
      }
      event "Layer_1.plyNum", "Layer_2.plyNum", "Layer_3.plyNum", "Layer_4.plyNum", "Layer_5.plyNum", "Layer_6.plyNum", "fabAttribs_1.ozPerYd2", "fabAttribs_2.ozPerYd2", "fabAttribs_3.ozPerYd2", "fabAttribs_4.ozPerYd2", "fabAttribs_5.ozPerYd2", "fabAttribs_6.ozPerYd2": Value Change {
        n985 = event-data() -> ()  [unwired: 1 in, 6 out]
        n986 = local read "Layer_1"() -> (w1701:T3)
        n987 = local read "Layer_2"() -> (w1700:T3)
        n988 = local read "Layer_3"() -> (w1699:T3)
        n989 = local read "Layer_4"() -> (w1698:T3)
        n990 = local read "Layer_5"() -> (w1697:T3)
        n991 = local read "Layer_6"() -> (w1696:T3)
        n992 = Build Array(w1701, w1700, w1699, w1698, w1697, w1696) -> (w1702:T14)
        n993 = local read "fabAttribs_1"() -> (w1704:T4)
        n994 = local read "fabAttribs_2"() -> (w1706:T4)
        n995 = local read "fabAttribs_3"() -> (w1707:T4)
        n996 = local read "fabAttribs_4"() -> (w1708:T4)
        n997 = local read "fabAttribs_5"() -> (w1709:T4)
        n998 = local read "fabAttribs_6"() -> (w1705:T4)
        n999 = Build Array(w1704, w1706, w1707, w1708, w1709, w1705) -> (w1703:T15)
        n1000 = for {
          tunnel: w1702 -> [w1729] mode=indexing
          shift-right: [w1731] -> w1711
          shift-left: 0 -> [w1730]
          tunnel: [w1728] -> w1721 mode=indexing
          tunnel: w1703 -> [w1725] mode=indexing
          n1001 = Unbundle By Name(w1725) -> ("ozPerYd2"=w1726:string)
          n1002 = Unbundle By Name(w1729) -> ("plyNum"=w1727:i32)
          n1003 = Scan From String(input string=w1726, default 1=sgl 0.0 ("default value 1")) -> (output 1=w1724:sgl)  [unwired: 3 in, 3 out]
          n1004 = Add(x=w1730, y=w1727) -> (x+y=w1731:i32)
          n1005 = To Single Precision Float(number=w1727) -> (single precision float=w1723:sgl)
          n1006 = Multiply(x=w1723, y=w1724) -> (x*y=w1728:sgl)
        }
        "totalNumPlies" <- w1711
        n1007 = Divide(x=w1721, y=sgl 144.0) -> (x/y=w1719:sgl[])
        n1008 = Index Array(array=w1719) -> (element #1=→"fab1_totalWt":sgl, element #2=→"fab2_totalWt":sgl, element #3=→"fab3_totalWt":sgl, element #4=→"fab4_totalWt":sgl, element #5=→"fab5_totalWt":sgl, element #6=→"fab6_totalWt":sgl)  [unwired: 6 in]
        n1009 = Add Array Elements(numeric array=w1719) -> (sum=→"totalBAW":sgl)
      }
      event "clayCalArray": Value Change {
        n1010 = event-data() -> ()  [unwired: 1 in, 6 out]
        n1011 = for {
          N: 5 -> [_]
          tunnel: "clayCalArray" -> [w1754] mode=indexing
          shift-right: [w1753] -> w1738
          shift-left: "" -> [w1751]
          shift-right: [w1748] -> w1734
          shift-left: i16[] [] -> [w1747]
          n1012 = Greater Than 0?(x=w1754) -> (x > 0?=w1755:bool)
          n1013 = case shown="False" w1755 {
            tunnel: w1754 -> [_ w1761]
            tunnel: ["##" ("clayCalib") w1763] -> w1752
            tunnel: w1751 -> [w1758 w1762]
            tunnel: [w1758 w1762] -> w1750
            tunnel: [w1756 w1760] -> w1748
            tunnel: w1747 -> [w1756 w1759]
            frame False {
            }
            frame True {
              n1014 = Format Into String(w1761) -> (resulting string=w1763:string)  [unwired: 3 in, 1 out]
              n1015 = Build Array (concatenate)(w1759, w1761) -> (w1760:i16[])
            }
          }
          n1016 = Concatenate Strings(w1750, w1752, "-" ("string")) -> (w1753:string)
        }
        n1017 = String Length(string=w1738) -> (length=w1739:i32)
        n1018 = Add Array Elements(numeric array=w1734) -> (sum=w1745:i16)
        n1019 = Array Size(array=w1734) -> (size(s)=w1746:i32)
        n1020 = Decrement(x=w1739) -> (x-1=w1736:i32)
        n1021 = To Single Precision Float(number=w1745) -> (single precision float=w1744:sgl)
        n1022 = To Single Precision Float(number=w1746) -> (single precision float=w1743:sgl)
        n1023 = String Subset(string=w1738, length (rest)=w1736) -> (substring=w1737:string)  [unwired: 1 in]
        n1024 = Divide(x=w1744, y=w1743) -> (x/y=→"clayAverage":sgl)
        n1025 = local write "clayCalib"(w1737) -> ()
      }
      event "getRecord": Value Change {
        n1026 = event-data() -> ()  [unwired: 1 in, 6 out]
        n1027 = local write "lookupRec"(TRUE ("lookupRec")) -> ()
      }
      event "Method": Value Change {
        n1028 = event-data() -> ("CtlRef"=w1770:refnum<vi>)  [unwired: 1 in, 5 out]
        n1029 = call "Dropdown Selection (SubVI).vi"("reference"=w1770) -> ("element"=w1769:string)
        n1030 = Equal?(x=w1769, y="V50") -> (x = y?=w1767:bool)
        n1031 = property on="minV50" class="DigNum (strict)"("Visible"=w1767) -> ()  [unwired: 2 in, 2 out]
      }
      event "workType": Value Change {
        n1032 = event-data() -> ("CtlRef"=w1771:refnum<vi>)  [unwired: 1 in, 5 out]
        n1033 = call "Dropdown Selection (SubVI).vi"("reference"=w1771) -> ("element"=w1774:string)
        n1034 = Equal?(x=w1774, y="QC") -> (x = y?=w1772:bool)
        n1035 = property on="minV50" class="DigNum (strict)"("Visible"=w1772) -> ()  [unwired: 2 in, 2 out]
      }
      event "rangeSetup": Value Change {
        n1036 = event-data() -> ("NewVal"=w1783:u16)  [unwired: 1 in, 5 out]
        n1037 = Greater Than 0?(x=w1783) -> (x > 0?=w1787:bool)
        n1038 = case shown="0, Default" w1783 {
          tunnel: ["0" ("section") "5.0" ("section") "7.5" ("section") "45.0" ("section")] -> w1778
          frame 0, Default {
          }
          frame 1 {
          }
          frame 2 {
          }
          frame 3 {
          }
        }
        n1039 = local read "configPath"() -> (w1780:path)
        n1040 = Not(x=w1787) -> (.not. x?=w1788:bool)
        n1041 = Select(t=u8 0 ("y"), s=w1787, f=u8 2 ("y")) -> (s? t:f=w1785:u8)
        n1042 = property on="instruct_addShot" class="Str"("Visible"=w1788) -> ()  [unwired: 2 in, 2 out]
        n1043 = property on="Accept Data" class="Bool (strict)"("Disabled"=w1785) -> ()  [unwired: 2 in, 2 out]
        n1044 = call <vilib>:"Open Config Data (compatibility).vi"("configuration file path"=w1780) -> ("error out"=w1792:errorcluster, "refnum"=w1794:T23)  [unwired: 8 in, 1 out]
        n1045 = call-poly <vilib>:"Write Key.vi"("write raw string? (F)"=TRUE, "section"="Ballistic Parameters", "error in (no error)"=w1792, "value"=w1778, "key"="MidPoint To Target Distance", "refnum"=w1794) -> ("error out"=w1791:errorcluster, "refnum out"=w1790:T23)  [unwired: 3 in, 1 out]
        n1046 = call <vilib>:"Close Config Data.vi"("error in (no error)"=w1791, "refnum"=w1790) -> ("error out"=w1779:errorcluster)  [unwired: 8 in, 1 out]
        n1047 = Scan From String(input string=w1778, error in=w1779, default 1=sgl 0.0 ("default value 1")) -> (output 1=w1777:sgl)  [unwired: 2 in, 3 out]
        n1048 = local write "mid_to_targ_dist"(w1777) -> ()
      }
    }
  }
  n1049 = disable-structure shown="Enabled" {
    frame Disabled {
      # "Apparently dead or unreachable code"
      # "DUPONT CONTACT SHOT REPORT (Unused)"
      # "This section prepares a Contact Shot report"
      n1050 = control-ref of="Shot Graph"() -> (w1801:refnum<vi>)
      n1051 = control-ref of="Sample #"() -> (w1800:refnum<vi>)
      n1052 = control-ref of="Report Path"() -> (w1799:refnum<vi>)
      n1053 = call "Contact Report (SubVI).vi"("reportPath_ref"=w1799, "SampleIDref"=w1800, "Shot Graph"=w1801) -> ()
    }
    frame Enabled {
    }
  }
  n1054 = local read "SHOTS"() -> (w1:T5[])
  n1055 = disable-structure shown="Enabled" {
    disable-tunnel: w1 -> [w1802 _]
    frame Disabled {
      # "SET PENETRATION STATUS"
      # "This section is supposed to switch the setting from partial to complete"
      n1056 = Array Size(array=w1802) -> (size(s)=w1812:i32)
      n1057 = Decrement(x=w1812) -> (x-1=w1804:i32)
      n1058 = Index Array(array=w1802, index=w1804) -> (element=w1807:T5)
      n1059 = Unbundle By Name(w1807) -> ("SHOT STATUS"=w1811:u16)
      n1060 = Equal To 0?(x=w1811) -> (x = 0?=w1810:bool)
      n1061 = Select(t=u16 1, s=w1810, f=u16 0) -> (s? t:f=w1806:u16)
      n1062 = local write "Current/sthotstatus"(w1806) -> ()
      n1063 = Bundle By Name(cluster=w1807, "SHOT STATUS"=w1806) -> (w1805:T5)
      n1064 = Replace Array Subset(array=w1802, new element=w1805, index=w1804) -> (w1803:T5[])
      n1065 = stacked-sequence {
        tunnel: w1806 -> [_]
        tunnel: w1803 -> [w1813]
        frame #0 {
          n1066 = call "Update Shot Table.vi"("shot array"=w1813) -> ("shotTable OUT"=w1814:string[][])
          n1067 = local write "Table of Shots"(w1814) -> ()
          n1068 = local write "SHOTS"(w1813) -> ()
        }
      }
    }
    frame Enabled {
    }
  }
